vi "CRYO_MASTER_FULL-old.vi"() -> ()   [LabVIEW 2017]
uses:
  LSI218Data.lvclass
  LSI336Data.lvclass
  USBData.lvclass
  6240AData.lvclass
  <vilib>/DAQmx/create/channels.llb/DAQmx Create Channel (DO-Digital Output).vi
  <vilib>/DAQmx/miscellaneous.llb/DAQmx Fill In Error Info.vi
  <vilib>/DAQmx/create/channels.llb/DAQmx Create Channel (AO-Voltage-Basic).vi
  <vilib>/express/express arith-compare/Formula/XNode/ExpressFormulaBlockNode.xnode
  <vilib>/Analysis/NI_AALBase.lvlib
panel:
  in  "Record interval":i64=10
  out "Cycle #":u32=132
  in  "Measurement Interval (s)":dbl=0.3
  in  "Stop Button":bool
  in  "?":T1(tab)
  out "error out (USB6210/6218 AOUT)":errorcluster
  in  "AOUT 1 Label":string="KIKUSUI_I"
  in  "AOUT 0 Label":string="KIKUSUI_V"
  in  "DOUT Labels":string[](array[string])=["D_V1_NO", "D_V2_NC", "D_CV1"]
  in  "AOUT for Current CTRL":tag="Dev1/ao1"
  in  "AOUT For Voltage CTRL":tag="Dev1/ao0"
  out "AO task out":refnum<k21>="20200912_074213_AO"
  in  "Analog Out ON?":bool=TRUE
  in  "InstName (USB6218)":string="USB6218"
  in  "USB6218 Config":T2(array[cluster])=[{"Label"="F_1", "FileFormat"="%5.5f", "Active?"=TRUE, "Physical CH"="Dev1/ai0", " terminal\n type"=10083, "ConversionType"={"Type"=enum."SimpleProp", "ConversionParameters"=[0.0, 5.0, 0.0, 500.0]}, "VoltageLimits"=[0.0, 5.0]}, {"Label"="F_2", "FileFormat"="%5.5f", "Active?"=TRUE, "Physical CH"="Dev1/ai1", " terminal\n type"=10083, "ConversionType"={"Type"=enum."SimpleProp", "ConversionParameters"=[0.0, 5.0, 0.0, 200.0]}, "VoltageLimits"=[0.0, 5.0]}, {"Label"="F_3", "FileFormat"="%5.5f", "Active?"=TRUE, "Physical CH"="Dev1/ai2", " terminal\n type"=10083, "ConversionType"={"Type"=enum."SimpleProp", "ConversionParameters"=[0.0, 5.0, 0.0, 200.0]}, "VoltageLimits"=[0.0, 5.0]}, {"Label"="F_4", "FileFormat"="%5.5f", "Active?"=TRUE, "Physical CH"="Dev1/ai3", " terminal\n type"=10083, "ConversionType"={"Type"=enum."SimpleProp", "ConversionParameters"=[0.0, 5.0, 0.0, 500.0]}, "VoltageLimits"=[0.0, 5.0]}, {"Label"="F_5", "FileFormat"="%5.5f", "Active?"=TRUE, "Physical CH"="Dev1/ai4", " terminal\n type"=10083, "ConversionType"={"Type"=enum."SimpleProp", "ConversionParameters"=[0.0, 5.0, 0.0, 500.0]}, "VoltageLimits"=[0.0, 5.0]}, {"Label"="I_CV", "FileFormat"="%3.5f", "Active?"=TRUE, "Physical CH"="Dev1/ai5", " terminal\n type"=10083, "ConversionType"={"Type"=enum."SimpleProp", "ConversionParameters"=[0.0, 10.0, 0.0, 2000.0]}, "VoltageLimits"=[0.0, 10.0]}, {"Label"="CV1_answer", "FileFormat"="%3.5f", "Active?"=TRUE, "Physical CH"="Dev1/ai6", " terminal\n type"=10083, "ConversionType"={"Type"=enum."SimpleProp", "ConversionParameters"=[1.0, 5.0, 0.0, 100.0]}, "VoltageLimits"=[0.0, 5.0]}] {"terminal\n type" items=["Default"=-1, "RSE"=10083, "NRSE"=10078, "Differential"=10106, "Pseudodifferential"=12529]}
  out "error out (USB6218)":errorcluster
  out "error out (USB6210/6218 DOUT)":errorcluster
  out "DOUT task out":refnum<k21>="20200912_074213_DO"
  in  "DOUT Physical CH":tag[](array[tag])=["Dev1/port1/line0", "Dev1/port1/line1", "Dev1/port1/line2"]
  in  "Digital Out ON?":bool=TRUE
  in  "USB6210 Config":T2(array[cluster])=[{"Label"="P_ins", "FileFormat"="%5.5e", "Active?"=TRUE, "Physical CH"="Dev2/ai0", " terminal\n type"=10083, "ConversionType"={"Type"=enum."CC-10_LOG", "ConversionParameters"=[0.5, 9.0, 0.0, 1.0]}, "VoltageLimits"=[0.0, 10.0]}, {"Label"="P_4Kres", "FileFormat"="%5.5e", "Active?"=TRUE, "Physical CH"="Dev2/ai1", " terminal\n type"=10083, "ConversionType"={"Type"=enum."SimpleProp", "ConversionParameters"=[1.0, 5.0, 0.0, 200000.0]}, "VoltageLimits"=[0.0, 5.0]}, {"Label"="P_3HeIN", "FileFormat"="%5.5e", "Active?"=TRUE, "Physical CH"="Dev2/ai2", " terminal\n type"=10083, "ConversionType"={"Type"=enum."SimpleProp", "ConversionParameters"=[1.0, 5.0, 0.0, 200000.0]}, "VoltageLimits"=[0.0, 5.0]}, {"Label"="P_SldRTN", "FileFormat"="%5.5e", "Active?"=TRUE, "Physical CH"="Dev2/ai3", " terminal\n type"=10083, "ConversionType"={"Type"=enum."SimpleProp", "ConversionParameters"=[1.0, 5.0, 0.0, 200000.0]}, "VoltageLimits"=[0.0, 5.0]}, {"Label"="P_3Hepot", "FileFormat"="%5.5e", "Active?"=TRUE, "Physical CH"="Dev2/ai4", " terminal\n type"=10083, "ConversionType"={"Type"=enum."SimpleProp", "ConversionParameters"=[0.0, 10.0, 0.0, 133320.0]}, "VoltageLimits"=[0.0, 10.0]}, {"Label"="P_1Kpot", "FileFormat"="%5.5e", "Active?"=TRUE, "Physical CH"="Dev2/ai5", " terminal\n type"=10083, "ConversionType"={"Type"=enum."SimpleProp", "ConversionParameters"=[0.0, 10.0, 0.0, 133320.0]}, "VoltageLimits"=[0.0, 10.0]}, {"Label"="P_Dewar", "FileFormat"="%5.5e", "Active?"=TRUE, "Physical CH"="Dev2/ai6", " terminal\n type"=10083, "ConversionType"={"Type"=enum."SimpleProp", "ConversionParameters"=[1.0, 5.0, 0.0, 200000.0]}, "VoltageLimits"=[0.0, 5.0]}, {"Label"="DP_HEX4", "FileFormat"="%5.5e", "Active?"=TRUE, "Physical CH"="Dev2/ai7", " terminal\n type"=10083, "ConversionType"={"Type"=enum."SimpleProp", "ConversionParameters"=[1.0, 5.0, 0.0, 1000.0]}, "VoltageLimits"=[0.0, 5.0]}, {"Label"="DP_HEX5", "FileFormat"="%5.5e", "Active?"=TRUE, "Physical CH"="Dev2/ai8", " terminal\n type"=10083, "ConversionType"={"Type"=enum."SimpleProp", "ConversionParameters"=[1.0, 5.0, 0.0, 20000.0]}, "VoltageLimits"=[0.0, 5.0]}, {"Label"="L1", "FileFormat"="%5.5f", "Active?"=TRUE, "Physical CH"="Dev2/ai9", " terminal\n type"=10083, "ConversionType"={"Type"=enum."SimpleProp", "ConversionParameters"=[0.0, 10.0, 0.0, 100.0]}, "VoltageLimits"=[0.0, 10.0]}, {"Label"="L2-1", "FileFormat"="%5.5f", "Active?"=TRUE, "Physical CH"="Dev2/ai10", " terminal\n type"=10083, "ConversionType"={"Type"=enum."SimpleProp", "ConversionParameters"=[0.0, 10.0, 0.0, 100.0]}, "VoltageLimits"=[0.0, 10.0]}, {"Label"="L2-2", "FileFormat"="%5.5f", "Active?"=TRUE, "Physical CH"="Dev2/ai11", " terminal\n type"=10083, "ConversionType"={"Type"=enum."SimpleProp", "ConversionParameters"=[0.0, 10.0, 0.0, 100.0]}, "VoltageLimits"=[0.0, 10.0]}, {"Label"="L3", "FileFormat"="%5.5f", "Active?"=TRUE, "Physical CH"="Dev2/ai12", " terminal\n type"=10083, "ConversionType"={"Type"=enum."SimpleProp", "ConversionParameters"=[0.0, 10.0, 0.0, 100.0]}, "VoltageLimits"=[0.0, 10.0]}] {"terminal\n type" items=["Default"=-1, "RSE"=10083, "NRSE"=10078, "Differential"=10106, "Pseudodifferential"=12529]}
  in  "RUN identifier":string="PreCooling"
  in  "Base Path":path=path "C:/LabVIEW/DATA/Precooling"
  in  "InstName (USB6210)":string="USB6210"
  out "error out (USB6210)":errorcluster
  out "File Refn USB AO":refnum<file>
  out "File Refn USB DO":refnum<file>
  out "error out (LSI336)":errorcluster
  in  "InstName (LSI336)":string="LSI336"
  in  "FileFormat (336)":string="%4.4f"
  in  "LSI336Settings(X,Y)":T3(array[cluster])=[{"LSIName"="LSi336X", "Labels"=["T1K3-1", "T1K3-2", "T3He5", "T3He8"], "SensorLocations"=[enum."T1K3-1", enum."T1K3-2", enum."T3He5", enum."T3He8"], "Active?"=TRUE, "VISA res. name"="GPIB0::6::INSTR"}, {"LSIName"="LSi336Y", "Labels"=["T3He6-1", "T3He6-2", "T3He7-1", "T3He7-2"], "SensorLocations"=[enum."T3He6-1", enum."T3He6-2", enum."T3He7-1", enum."T3He7-2"], "Active?"=TRUE, "VISA res. name"="GPIB0::2::INSTR"}]
  in  "FileFormat (218)":string="%4.4f"
  in  "InstName (LSI218)":string="LSI218"
  in  "LSI218Settings(A-F)":T3(array[cluster])=[{"LSIName"="LSI218A", "Labels"=["T3He10", "T3He1-1", "TTH3", "TTH4", "TTH1", "TTH2", "T4He1", "T1K1"], "SensorLocations"=[enum."T3He10", enum."T3He1-1", enum."TTH3", enum."TTH4", enum."TTH1", enum."TTH2", enum."T4He1", enum."T1K1"], "Active?"=TRUE, "VISA res. name"="GPIB0::7::INSTR"}, {"LSIName"="LSI218B", "Labels"=["N.C.", "N.C.", "N.C.", "N.C.", "T3He2-1", "T3He2-2", "T3He3", "T3He1-4"], "SensorLocations"=[enum."N.C.", enum."N.C.", enum."N.C.", enum."T3He1-4", enum."T3He2-1", enum."T3He2-2", enum."T3He3", enum."T3He1-4"], "Active?"=TRUE, "VISA res. name"="GPIB0::4::INSTR"}, {"LSIName"="LSI218C", "Labels"=["T4He3-1", "T4He3-2", "T4He3-3", "T4He3-4", "T4He2-1", "T4He2-2", "T4He4", "T4He5"], "SensorLocations"=[enum."T4He3-1", enum."T4He3-2", enum."T4He3-3", enum."T4He3-4", enum."T4He2-1", enum."T4He2-2", enum."T4He4", enum."T4He5"], "Active?"=TRUE, "VISA res. name"="GPIB0::3::INSTR"}, {"LSIName"="LSI218D", "Labels"=["T4He6", "T4He9", "T3He1-2", "T3He1-3", "T4He7", "T4He8", "T4He10", "T1K6"], "SensorLocations"=[enum."T4He6", enum."T4He9", enum."T3He1-2", enum."T3He1-3", enum."T4He7", enum."T4He8", enum."T4He10", enum."T1K6"], "Active?"=TRUE, "VISA res. name"="GPIB0::5::INSTR"}, {"LSIName"="LSI218E", "Labels"=["TIP1", "N.C.", "TIP2", "N.C.", "TIP3", "TIP4", "TIP5", "N.C."], "SensorLocations"=[enum."TIP1", enum."N.C.", enum."TIP2", enum."N.C.", enum."TIP3", enum."TIP4", enum."TIP5", enum."N.C."], "Active?"=TRUE, "VISA res. name"="GPIB0::11::INSTR"}, {"LSIName"="LSI218F", "Labels"=["T1K2", "T1K4", "T1K5", "T3He4", "T3He9", "TIP6", "N.C.", "N.C."], "SensorLocations"=[enum."T1K2", enum."T1K4", enum."T1K5", enum."T3He4", enum."T3He9", enum."TIP6", enum."N.C.", enum."N.C."], "Active?"=TRUE, "VISA res. name"="GPIB0::8::INSTR"}]
  out "error out (LSI218)":errorcluster
  out "Graph 3":T4(graph) caption="XY Graph"
  out "Graph 1":T4(graph)=[{"TimeArray"=[timestamp(3682708934.7497134 s since 1904-01-01), timestamp(3682708935.064348 s since 1904-01-01), timestamp(3682708935.3896832 s since 1904-01-01), timestamp(3682708935.7026334 s since 1904-01-01), timestamp(3682708936.0021167 s since 1904-01-01), timestamp(3682708936.3049774 s since 1904-01-01), timestamp(3682708936.605407 s since 1904-01-01), timestamp(3682708936.903053 s since 1904-01-01), timestamp(3682708937.3067694 s since 1904-01-01), timestamp(3682708937.611465 s since 1904-01-01), timestamp(3682708937.909672 s since 1904-01-01), timestamp(3682708938.228514 s since 1904-01-01), timestamp(3682708938.527811 s since 1904-01-01), timestamp(3682708938.931336 s since 1904-01-01), timestamp(3682708940.012947 s since 1904-01-01), timestamp(3682708940.32849 s since 1904-01-01), timestamp(3682708940.631708 s since 1904-01-01), timestamp(3682708940.946489 s since 1904-01-01), timestamp(3682708941.244303 s since 1904-01-01), timestamp(3682708941.542656 s since 1904-01-01), timestamp(3682708941.8474927 s since 1904-01-01), timestamp(3682708942.3104415 s since 1904-01-01), timestamp(3682708942.6136575 s since 1904-01-01), timestamp(3682708942.916794 s since 1904-01-01), timestamp(3682708943.238447 s since 1904-01-01), timestamp(3682708943.5371313 s since 1904-01-01), timestamp(3682708943.857245 s since 1904-01-01), timestamp(3682708944.1856494 s since 1904-01-01), timestamp(3682708944.4866023 s since 1904-01-01), timestamp(3682708944.805397 s since 1904-01-01), timestamp(3682708945.111448 s since 1904-01-01), timestamp(3682708945.435288 s since 1904-01-01), timestamp(3682708945.7333007 s since 1904-01-01), timestamp(3682708946.0530386 s since 1904-01-01), timestamp(3682708946.4366784 s since 1904-01-01), timestamp(3682708946.732824 s since 1904-01-01), timestamp(3682708947.0537186 s since 1904-01-01), timestamp(3682708947.3846655 s since 1904-01-01), timestamp(3682708947.712872 s since 1904-01-01), timestamp(3682708948.0188503 s since 1904-01-01), timestamp(3682708948.737391 s since 1904-01-01), timestamp(3682708949.201587 s since 1904-01-01), timestamp(3682708949.502657 s since 1904-01-01), timestamp(3682708949.805978 s since 1904-01-01), timestamp(3682708950.1212378 s since 1904-01-01), timestamp(3682708950.4333377 s since 1904-01-01), timestamp(3682708950.732243 s since 1904-01-01), timestamp(3682708951.1057153 s since 1904-01-01), timestamp(3682708951.4068193 s since 1904-01-01), timestamp(3682708951.8357983 s since 1904-01-01), timestamp(3682708952.143476 s since 1904-01-01), timestamp(3682708952.4476566 s since 1904-01-01), timestamp(3682708952.7855697 s since 1904-01-01), timestamp(3682708953.086301 s since 1904-01-01), timestamp(3682708953.4027033 s since 1904-01-01), timestamp(3682708953.706577 s since 1904-01-01), timestamp(3682708954.023016 s since 1904-01-01), timestamp(3682708954.330558 s since 1904-01-01), timestamp(3682708954.643428 s since 1904-01-01), timestamp(3682708955.050496 s since 1904-01-01), timestamp(3682708955.3527017 s since 1904-01-01), timestamp(3682708955.7328424 s since 1904-01-01), timestamp(3682708956.0574985 s since 1904-01-01), timestamp(3682708956.3904 s since 1904-01-01), timestamp(3682708956.7025185 s since 1904-01-01), timestamp(3682708957.032419 s since 1904-01-01), timestamp(3682708957.351427 s since 1904-01-01), timestamp(3682708957.6656775 s since 1904-01-01), timestamp(3682708958.051097 s since 1904-01-01), timestamp(3682708958.4033985 s since 1904-01-01), timestamp(3682708958.7021422 s since 1904-01-01), timestamp(3682708959.004737 s since 1904-01-01), timestamp(3682708959.3058767 s since 1904-01-01), timestamp(3682708959.6056495 s since 1904-01-01), timestamp(3682708959.9347386 s since 1904-01-01), timestamp(3682708960.252382 s since 1904-01-01), timestamp(3682708960.553459 s since 1904-01-01), timestamp(3682708960.8641214 s since 1904-01-01), timestamp(3682708961.160152 s since 1904-01-01), timestamp(3682708961.487622 s since 1904-01-01), timestamp(3682708961.788169 s since 1904-01-01), timestamp(3682708962.0896144 s since 1904-01-01), timestamp(3682708962.406388 s since 1904-01-01), timestamp(3682708962.70866 s since 1904-01-01), timestamp(3682708963.033897 s since 1904-01-01), timestamp(3682708963.3512735 s since 1904-01-01), timestamp(3682708963.668318 s since 1904-01-01), timestamp(3682708963.9877753 s since 1904-01-01), timestamp(3682708964.2907033 s since 1904-01-01), timestamp(3682708964.606549 s since 1904-01-01), timestamp(3682708964.906368 s since 1904-01-01), timestamp(3682708965.217731 s since 1904-01-01), timestamp(3682708965.5397863 s since 1904-01-01), timestamp(3682708965.8690424 s since 1904-01-01), timestamp(3682708966.190765 s since 1904-01-01), timestamp(3682708966.5023417 s since 1904-01-01), timestamp(3682708966.806744 s since 1904-01-01), timestamp(3682708967.1092105 s since 1904-01-01), timestamp(3682708967.406003 s since 1904-01-01), timestamp(3682708967.710469 s since 1904-01-01), timestamp(3682708968.041528 s since 1904-01-01), timestamp(3682708968.365668 s since 1904-01-01), timestamp(3682708968.8523655 s since 1904-01-01), timestamp(3682708969.1540494 s since 1904-01-01), timestamp(3682708969.4895535 s since 1904-01-01), timestamp(3682708969.7907286 s since 1904-01-01), timestamp(3682708970.105831 s since 1904-01-01), timestamp(3682708970.4602976 s since 1904-01-01), timestamp(3682708970.963533 s since 1904-01-01), timestamp(3682708971.301882 s since 1904-01-01), timestamp(3682708971.6079335 s since 1904-01-01), timestamp(3682708971.9060354 s since 1904-01-01), timestamp(3682708972.2345 s since 1904-01-01), timestamp(3682708972.5527015 s since 1904-01-01), timestamp(3682708972.8548064 s since 1904-01-01), timestamp(3682708973.582567 s since 1904-01-01), timestamp(3682708973.8891873 s since 1904-01-01), timestamp(3682708974.1884327 s since 1904-01-01), timestamp(3682708974.5010185 s since 1904-01-01), timestamp(3682708974.8142066 s since 1904-01-01), timestamp(3682708975.1175103 s since 1904-01-01), timestamp(3682708975.4374647 s since 1904-01-01), timestamp(3682708975.7527 s since 1904-01-01), timestamp(3682708976.0583982 s since 1904-01-01), timestamp(3682708976.3644648 s since 1904-01-01), timestamp(3682708976.689261 s since 1904-01-01), timestamp(3682708977.0021367 s since 1904-01-01), timestamp(3682708977.3057 s since 1904-01-01), timestamp(3682708977.6422114 s since 1904-01-01), timestamp(3682708977.9607697 s since 1904-01-01), timestamp(3682708978.2889266 s since 1904-01-01), timestamp(3682708978.7650247 s since 1904-01-01)], "DataArray"=[102202.16534140152, 100161.43201016451, 100789.60275186355, 100345.60782032329, 102337.00779239179, 101526.30582974949, 102083.76617517172, 102660.95994909719, 100931.02351867667, 101384.88517891317, 103307.21992056293, 101878.21277938908, 100806.04675539682]}] caption="XY Graph"
  in  "FIle suffix 4":string="Graph4"
  in  "Take Screenshot! 4":bool
  in  "FIle suffix 3":string="Graph3"
  in  "Take Screenshot! 3":bool
  in  "FIle suffix 2":string="Graph2"
  in  "Take Screenshot! 2":bool
  in  "FIle suffix 1":string="Graph1"
  in  "Take Screenshot! 1":bool
  in  "log/linear 2":bool
  in  "Tab Control 2":T5(tab)
  in  "Plot selecter (USB6210)\n    1      2     3     4":bool[][](array[boolean])=[[FALSE, FALSE, TRUE, FALSE], [FALSE, FALSE, TRUE, FALSE], [FALSE, FALSE, TRUE, FALSE], [FALSE, FALSE, TRUE, FALSE], [FALSE, FALSE, TRUE, FALSE], [FALSE, FALSE, TRUE, FALSE], [TRUE, FALSE, FALSE, FALSE], [FALSE, FALSE, TRUE, FALSE], [FALSE, FALSE, TRUE, FALSE], [FALSE, FALSE, FALSE, TRUE], [FALSE, FALSE, FALSE, TRUE], [FALSE, FALSE, FALSE, TRUE], [FALSE, FALSE, FALSE, TRUE], [FALSE, FALSE, FALSE, FALSE], [FALSE, FALSE, FALSE, FALSE], [FALSE, FALSE, FALSE, FALSE]]
  out "All Labels (USB6210)":string[](array[string])=["P_ins", "P_4Kres", "P_3HeIN", "P_SldRTN", "P_3Hepot", "P_1Kpot", "P_Dewar", "DP_HEX4", "DP_HEX5", "L1", "L2-1", "L2-2", "L3"]
  out "Last Data \n(USB6210)":dbl[](array[numeric])=[0.0002840544512641805, 101675.94822078843, 101115.19883009115, 101138.22078317008, 101187.0271133805, 101386.92986598553, 102226.83192072672, -14.050296706315413, 60.37240293708335, 100.07360118845727, 0.1408656089962046, 0.11784872774401622, 0.16848586636495688] format="%#_6e"
  out "Time of Last Measurement (USB6210)":timestamp=timestamp(3682708978.7650247 s since 1904-01-01)
  out "USB6210 Status":T6(ring)=enum."Ready"
  out "Last Vol\n(USB6210)":dbl[](array[numeric])=[5.726700799630656, 3.0335189644157685, 3.022303976601823, 3.0227644156634015, 7.5897860121047485, 7.604780217970712, 3.0445366384145345, 0.9437988131747383, 1.0120744805874167, 10.007360118845728, 0.01408656089962046, 0.011784872774401623, 0.016848586636495688] format="%_5f"
  out "Time of Last Measurement (USB6218)":timestamp=timestamp(3682708978.761338 s since 1904-01-01)
  out "USB6218 Status":T6(ring)=enum."Ready"
  out "Last Vol \n(USB6218)":dbl[](array[numeric])=[0.11165481522010053, 0.007099956900383277, 0.005192981435202531, -0.08736109093903988, 0.3091911402370971, 0.017826732521314358, -0.0006594605889951533] format="%_5f"
  out "Last Data \n(USB6218)":dbl[](array[numeric])=[11.165481522010053, 0.28399827601533106, 0.20771925740810127, -8.736109093903988, 30.91911402370971, 0.017826732521314358, -25.01648651472488] format="%#_6e"
  out "All Labels (USB6218)":string[](array[string])=["F_1", "F_2", "F_3", "F_4", "F_5", "I_CV", "CV1_answer"]
  in  "Plot selecter (USB6218)\n    1      2     3     4":bool[][](array[boolean])=[[FALSE, FALSE, TRUE, FALSE], [FALSE, FALSE, TRUE, FALSE], [FALSE, FALSE, TRUE, FALSE], [FALSE, FALSE, TRUE, FALSE], [FALSE, FALSE, TRUE, FALSE], [FALSE, FALSE, TRUE, FALSE], [FALSE, FALSE, FALSE, FALSE], [FALSE, FALSE, TRUE, FALSE], [FALSE, FALSE, TRUE, FALSE], [FALSE, FALSE, FALSE, TRUE], [FALSE, FALSE, FALSE, TRUE], [FALSE, FALSE, FALSE, TRUE], [FALSE, FALSE, FALSE, TRUE], [FALSE, FALSE, FALSE, FALSE], [FALSE, FALSE, FALSE, FALSE], [FALSE, FALSE, FALSE, FALSE]]
  out "Time of Last Measurement (LSI218)":timestamp=timestamp(3682708978.761338 s since 1904-01-01)
  out "LSI218 Status":T7(ring)=enum."Measuring"
  out "Last Data \nLSI218 (1)":dbl[](array[numeric])=[284.43, 290.03, 243.23, 256.15, 171.54, 180.77, 63.049, 117.3, 30.0, 0.0, 0.0, 0.0, 202.72, 191.34, 122.93, 289.61, 292.19, 292.34, 291.95, 292.02, 202.48, 197.55, 192.92, 186.55]
  out "Labels LSI218 (1)":string[](array[string])=["T3He10", "T3He1-1", "TTH3", "TTH4", "TTH1", "TTH2", "T4He1", "T1K1", "N.C.", "N.C.", "N.C.", "N.C.", "T3He2-1", "T3He2-2", "T3He3", "T3He1-4", "T4He3-1", "T4He3-2", "T4He3-3", "T4He3-4", "T4He2-1", "T4He2-2", "T4He4", "T4He5"]
  in  "Plot selecter LSI218(1)\n    1      2     3     4":bool[][](array[boolean])=[[FALSE, FALSE, FALSE, FALSE], [FALSE, FALSE, FALSE, FALSE], [FALSE, FALSE, FALSE, FALSE], [FALSE, FALSE, FALSE, FALSE], [FALSE, FALSE, FALSE, FALSE], [FALSE, FALSE, FALSE, FALSE], [FALSE, FALSE, FALSE, FALSE], [FALSE, FALSE, FALSE, FALSE], [FALSE, FALSE, FALSE, FALSE], [FALSE, FALSE, FALSE, FALSE], [FALSE, FALSE, FALSE, FALSE], [FALSE, FALSE, FALSE, FALSE], [FALSE, FALSE, FALSE, FALSE], [FALSE, FALSE, FALSE, FALSE], [FALSE, FALSE, FALSE, FALSE], [FALSE, FALSE, FALSE, FALSE], [FALSE, FALSE, FALSE, FALSE], [FALSE, FALSE, FALSE, FALSE], [FALSE, FALSE, FALSE, FALSE], [FALSE, FALSE, FALSE, FALSE], [FALSE, FALSE, FALSE, FALSE], [FALSE, FALSE, FALSE, FALSE], [FALSE, FALSE, FALSE, FALSE], [FALSE, FALSE, FALSE, FALSE]]
  out "Active?\n (1)":bool[](array[boolean])=[TRUE, TRUE, TRUE, TRUE, TRUE, TRUE, TRUE, TRUE, TRUE, TRUE, TRUE, TRUE, TRUE, TRUE, TRUE, TRUE, TRUE, TRUE, TRUE, TRUE, TRUE, TRUE, TRUE, TRUE]
  out "Labels LSI218 (2)":string[](array[string])=["T4He6", "T4He9", "T3He1-2", "T3He1-3", "T4He7", "T4He8", "T4He10", "T1K6", "TIP1", "N.C.", "TIP2", "N.C.", "TIP3", "TIP4", "TIP5", "N.C.", "T1K2", "T1K4", "T1K5", "T3He4", "T3He9", "TIP6", "N.C.", "N.C."]
  out "Active?\n(2)":bool[](array[boolean])=[TRUE, TRUE, TRUE, TRUE, TRUE, TRUE, TRUE, TRUE, TRUE, TRUE, TRUE, TRUE, TRUE, TRUE, TRUE, TRUE, TRUE, TRUE, TRUE, TRUE, TRUE, TRUE, TRUE, TRUE]
  out "Last Data \nLSI218 (2)":dbl[](array[numeric])=[192.44, 234.78, 290.18, 290.03, 246.41, 271.83, 269.02, 283.26, 278.46, 0.0, 229.12, 688.49, 197.75, 114.09, 159.57, 688.58, 121.27, 92.631, 95.353, 144.45, 121.36, 152.88, 0.433, 0.0]
  in  "Plot selecter LSI218(2)\n    1      2     3     4":bool[][](array[boolean])=[[FALSE, TRUE, FALSE, FALSE], [FALSE, TRUE, FALSE, FALSE], [FALSE, TRUE, FALSE, FALSE], [FALSE, TRUE, FALSE, FALSE], [FALSE, TRUE, FALSE, FALSE], [FALSE, TRUE, FALSE, FALSE], [FALSE, TRUE, FALSE, FALSE], [FALSE, TRUE, FALSE, FALSE], [FALSE, TRUE, FALSE, FALSE], [FALSE, TRUE, FALSE, FALSE], [FALSE, TRUE, FALSE, FALSE], [FALSE, FALSE, FALSE, FALSE], [FALSE, FALSE, FALSE, FALSE], [FALSE, FALSE, FALSE, FALSE], [FALSE, FALSE, FALSE, FALSE], [FALSE, FALSE, FALSE, FALSE], [FALSE, FALSE, FALSE, FALSE], [FALSE, FALSE, FALSE, FALSE], [FALSE, FALSE, FALSE, FALSE], [FALSE, FALSE, FALSE, FALSE], [FALSE, FALSE, FALSE, FALSE], [FALSE, FALSE, FALSE, FALSE], [FALSE, FALSE, FALSE, FALSE], [FALSE, FALSE, FALSE, FALSE]]
  in  "Plot selecter LSI336 \n     1      2     3     4":bool[][](array[boolean])=[[FALSE, TRUE, FALSE, FALSE], [FALSE, TRUE, FALSE, FALSE], [FALSE, TRUE, FALSE, FALSE], [FALSE, TRUE, FALSE, FALSE], [FALSE, TRUE, FALSE, FALSE], [FALSE, TRUE, FALSE, FALSE], [FALSE, TRUE, FALSE, FALSE], [FALSE, TRUE, FALSE, FALSE]]
  out "Time of Last Measurement (LSI336)":timestamp=timestamp(3682708978.761338 s since 1904-01-01)
  out "Last Data \nLSI336":dbl[](array[numeric])=[94.5454, 94.3475, 128.374, 133.795, 135.029, 135.063, 134.969, 134.048]
  out "Active?\n(LSI336)":bool[](array[boolean])=[TRUE, TRUE, TRUE, TRUE, TRUE, TRUE, TRUE, TRUE]
  out "Labels LSI336":string[](array[string])=["T1K3-1", "T1K3-2", "T3He5", "T3He8", "T3He6-1", "T3He6-2", "T3He7-1", "T3He7-2"]
  out "LSI336 Status":T7(ring)=enum."Measuring"
  in  "log/linear 1":bool
  out "Graph 2":T4(graph) caption="XY Graph"
  out "Graph 4":T4(graph)=[{"TimeArray"=[timestamp(3682708934.7497134 s since 1904-01-01), timestamp(3682708935.064348 s since 1904-01-01), timestamp(3682708935.3896832 s since 1904-01-01), timestamp(3682708935.7026334 s since 1904-01-01), timestamp(3682708936.0021167 s since 1904-01-01), timestamp(3682708936.3049774 s since 1904-01-01), timestamp(3682708936.605407 s since 1904-01-01), timestamp(3682708936.903053 s since 1904-01-01), timestamp(3682708937.3067694 s since 1904-01-01), timestamp(3682708937.611465 s since 1904-01-01), timestamp(3682708937.909672 s since 1904-01-01), timestamp(3682708938.228514 s since 1904-01-01), timestamp(3682708938.527811 s since 1904-01-01), timestamp(3682708938.931336 s since 1904-01-01), timestamp(3682708940.012947 s since 1904-01-01), timestamp(3682708940.32849 s since 1904-01-01), timestamp(3682708940.631708 s since 1904-01-01), timestamp(3682708940.946489 s since 1904-01-01), timestamp(3682708941.244303 s since 1904-01-01), timestamp(3682708941.542656 s since 1904-01-01), timestamp(3682708941.8474927 s since 1904-01-01), timestamp(3682708942.3104415 s since 1904-01-01), timestamp(3682708942.6136575 s since 1904-01-01), timestamp(3682708942.916794 s since 1904-01-01), timestamp(3682708943.238447 s since 1904-01-01), timestamp(3682708943.5371313 s since 1904-01-01), timestamp(3682708943.857245 s since 1904-01-01), timestamp(3682708944.1856494 s since 1904-01-01), timestamp(3682708944.4866023 s since 1904-01-01), timestamp(3682708944.805397 s since 1904-01-01), timestamp(3682708945.111448 s since 1904-01-01), timestamp(3682708945.435288 s since 1904-01-01), timestamp(3682708945.7333007 s since 1904-01-01), timestamp(3682708946.0530386 s since 1904-01-01), timestamp(3682708946.4366784 s since 1904-01-01), timestamp(3682708946.732824 s since 1904-01-01), timestamp(3682708947.0537186 s since 1904-01-01), timestamp(3682708947.3846655 s since 1904-01-01), timestamp(3682708947.712872 s since 1904-01-01), timestamp(3682708948.0188503 s since 1904-01-01), timestamp(3682708948.737391 s since 1904-01-01), timestamp(3682708949.201587 s since 1904-01-01), timestamp(3682708949.502657 s since 1904-01-01), timestamp(3682708949.805978 s since 1904-01-01), timestamp(3682708950.1212378 s since 1904-01-01), timestamp(3682708950.4333377 s since 1904-01-01), timestamp(3682708950.732243 s since 1904-01-01), timestamp(3682708951.1057153 s since 1904-01-01), timestamp(3682708951.4068193 s since 1904-01-01), timestamp(3682708951.8357983 s since 1904-01-01), timestamp(3682708952.143476 s since 1904-01-01), timestamp(3682708952.4476566 s since 1904-01-01), timestamp(3682708952.7855697 s since 1904-01-01), timestamp(3682708953.086301 s since 1904-01-01), timestamp(3682708953.4027033 s since 1904-01-01), timestamp(3682708953.706577 s since 1904-01-01), timestamp(3682708954.023016 s since 1904-01-01), timestamp(3682708954.330558 s since 1904-01-01), timestamp(3682708954.643428 s since 1904-01-01), timestamp(3682708955.050496 s since 1904-01-01), timestamp(3682708955.3527017 s since 1904-01-01), timestamp(3682708955.7328424 s since 1904-01-01), timestamp(3682708956.0574985 s since 1904-01-01), timestamp(3682708956.3904 s since 1904-01-01), timestamp(3682708956.7025185 s since 1904-01-01), timestamp(3682708957.032419 s since 1904-01-01), timestamp(3682708957.351427 s since 1904-01-01), timestamp(3682708957.6656775 s since 1904-01-01), timestamp(3682708958.051097 s since 1904-01-01), timestamp(3682708958.4033985 s since 1904-01-01), timestamp(3682708958.7021422 s since 1904-01-01), timestamp(3682708959.004737 s since 1904-01-01), timestamp(3682708959.3058767 s since 1904-01-01), timestamp(3682708959.6056495 s since 1904-01-01), timestamp(3682708959.9347386 s since 1904-01-01), timestamp(3682708960.252382 s since 1904-01-01), timestamp(3682708960.553459 s since 1904-01-01), timestamp(3682708960.8641214 s since 1904-01-01), timestamp(3682708961.160152 s since 1904-01-01), timestamp(3682708961.487622 s since 1904-01-01), timestamp(3682708961.788169 s since 1904-01-01), timestamp(3682708962.0896144 s since 1904-01-01), timestamp(3682708962.406388 s since 1904-01-01), timestamp(3682708962.70866 s since 1904-01-01), timestamp(3682708963.033897 s since 1904-01-01), timestamp(3682708963.3512735 s since 1904-01-01), timestamp(3682708963.668318 s since 1904-01-01), timestamp(3682708963.9877753 s since 1904-01-01), timestamp(3682708964.2907033 s since 1904-01-01), timestamp(3682708964.606549 s since 1904-01-01), timestamp(3682708964.906368 s since 1904-01-01), timestamp(3682708965.217731 s since 1904-01-01), timestamp(3682708965.5397863 s since 1904-01-01), timestamp(3682708965.8690424 s since 1904-01-01), timestamp(3682708966.190765 s since 1904-01-01), timestamp(3682708966.5023417 s since 1904-01-01), timestamp(3682708966.806744 s since 1904-01-01), timestamp(3682708967.1092105 s since 1904-01-01), timestamp(3682708967.406003 s since 1904-01-01), timestamp(3682708967.710469 s since 1904-01-01), timestamp(3682708968.041528 s since 1904-01-01), timestamp(3682708968.365668 s since 1904-01-01), timestamp(3682708968.8523655 s since 1904-01-01), timestamp(3682708969.1540494 s since 1904-01-01), timestamp(3682708969.4895535 s since 1904-01-01), timestamp(3682708969.7907286 s since 1904-01-01), timestamp(3682708970.105831 s since 1904-01-01), timestamp(3682708970.4602976 s since 1904-01-01), timestamp(3682708970.963533 s since 1904-01-01), timestamp(3682708971.301882 s since 1904-01-01), timestamp(3682708971.6079335 s since 1904-01-01), timestamp(3682708971.9060354 s since 1904-01-01), timestamp(3682708972.2345 s since 1904-01-01), timestamp(3682708972.5527015 s since 1904-01-01), timestamp(3682708972.8548064 s since 1904-01-01), timestamp(3682708973.582567 s since 1904-01-01), timestamp(3682708973.8891873 s since 1904-01-01), timestamp(3682708974.1884327 s since 1904-01-01), timestamp(3682708974.5010185 s since 1904-01-01), timestamp(3682708974.8142066 s since 1904-01-01), timestamp(3682708975.1175103 s since 1904-01-01), timestamp(3682708975.4374647 s since 1904-01-01), timestamp(3682708975.7527 s since 1904-01-01), timestamp(3682708976.0583982 s since 1904-01-01), timestamp(3682708976.3644648 s since 1904-01-01), timestamp(3682708976.689261 s since 1904-01-01), timestamp(3682708977.0021367 s since 1904-01-01), timestamp(3682708977.3057 s since 1904-01-01), timestamp(3682708977.6422114 s since 1904-01-01), timestamp(3682708977.9607697 s since 1904-01-01), timestamp(3682708978.2889266 s since 1904-01-01), timestamp(3682708978.7650247 s since 1904-01-01)], "DataArray"=[100.06505169937662, 100.0913578166008, 100.07097057589947, 100.0722858814967, 100.04006088884337, 100.09201547031509, 100.04006088897802, 100.01375477333622, 100.06833996442191, 100.05058333549653, 100.01441242568171, 100.06899761748156, 100.07688945274376]}, {"TimeArray"=[timestamp(3682708934.7497134 s since 1904-01-01), timestamp(3682708935.064348 s since 1904-01-01), timestamp(3682708935.3896832 s since 1904-01-01), timestamp(3682708935.7026334 s since 1904-01-01), timestamp(3682708936.0021167 s since 1904-01-01), timestamp(3682708936.3049774 s since 1904-01-01), timestamp(3682708936.605407 s since 1904-01-01), timestamp(3682708936.903053 s since 1904-01-01), timestamp(3682708937.3067694 s since 1904-01-01), timestamp(3682708937.611465 s since 1904-01-01), timestamp(3682708937.909672 s since 1904-01-01), timestamp(3682708938.228514 s since 1904-01-01), timestamp(3682708938.527811 s since 1904-01-01), timestamp(3682708938.931336 s since 1904-01-01), timestamp(3682708940.012947 s since 1904-01-01), timestamp(3682708940.32849 s since 1904-01-01), timestamp(3682708940.631708 s since 1904-01-01), timestamp(3682708940.946489 s since 1904-01-01), timestamp(3682708941.244303 s since 1904-01-01), timestamp(3682708941.542656 s since 1904-01-01), timestamp(3682708941.8474927 s since 1904-01-01), timestamp(3682708942.3104415 s since 1904-01-01), timestamp(3682708942.6136575 s since 1904-01-01), timestamp(3682708942.916794 s since 1904-01-01), timestamp(3682708943.238447 s since 1904-01-01), timestamp(3682708943.5371313 s since 1904-01-01), timestamp(3682708943.857245 s since 1904-01-01), timestamp(3682708944.1856494 s since 1904-01-01), timestamp(3682708944.4866023 s since 1904-01-01), timestamp(3682708944.805397 s since 1904-01-01), timestamp(3682708945.111448 s since 1904-01-01), timestamp(3682708945.435288 s since 1904-01-01), timestamp(3682708945.7333007 s since 1904-01-01), timestamp(3682708946.0530386 s since 1904-01-01), timestamp(3682708946.4366784 s since 1904-01-01), timestamp(3682708946.732824 s since 1904-01-01), timestamp(3682708947.0537186 s since 1904-01-01), timestamp(3682708947.3846655 s since 1904-01-01), timestamp(3682708947.712872 s since 1904-01-01), timestamp(3682708948.0188503 s since 1904-01-01), timestamp(3682708948.737391 s since 1904-01-01), timestamp(3682708949.201587 s since 1904-01-01), timestamp(3682708949.502657 s since 1904-01-01), timestamp(3682708949.805978 s since 1904-01-01), timestamp(3682708950.1212378 s since 1904-01-01), timestamp(3682708950.4333377 s since 1904-01-01), timestamp(3682708950.732243 s since 1904-01-01), timestamp(3682708951.1057153 s since 1904-01-01), timestamp(3682708951.4068193 s since 1904-01-01), timestamp(3682708951.8357983 s since 1904-01-01), timestamp(3682708952.143476 s since 1904-01-01), timestamp(3682708952.4476566 s since 1904-01-01), timestamp(3682708952.7855697 s since 1904-01-01), timestamp(3682708953.086301 s since 1904-01-01), timestamp(3682708953.4027033 s since 1904-01-01), timestamp(3682708953.706577 s since 1904-01-01), timestamp(3682708954.023016 s since 1904-01-01), timestamp(3682708954.330558 s since 1904-01-01), timestamp(3682708954.643428 s since 1904-01-01), timestamp(3682708955.050496 s since 1904-01-01), timestamp(3682708955.3527017 s since 1904-01-01), timestamp(3682708955.7328424 s since 1904-01-01), timestamp(3682708956.0574985 s since 1904-01-01), timestamp(3682708956.3904 s since 1904-01-01), timestamp(3682708956.7025185 s since 1904-01-01), timestamp(3682708957.032419 s since 1904-01-01), timestamp(3682708957.351427 s since 1904-01-01), timestamp(3682708957.6656775 s since 1904-01-01), timestamp(3682708958.051097 s since 1904-01-01), timestamp(3682708958.4033985 s since 1904-01-01), timestamp(3682708958.7021422 s since 1904-01-01), timestamp(3682708959.004737 s since 1904-01-01), timestamp(3682708959.3058767 s since 1904-01-01), timestamp(3682708959.6056495 s since 1904-01-01), timestamp(3682708959.9347386 s since 1904-01-01), timestamp(3682708960.252382 s since 1904-01-01), timestamp(3682708960.553459 s since 1904-01-01), timestamp(3682708960.8641214 s since 1904-01-01), timestamp(3682708961.160152 s since 1904-01-01), timestamp(3682708961.487622 s since 1904-01-01), timestamp(3682708961.788169 s since 1904-01-01), timestamp(3682708962.0896144 s since 1904-01-01), timestamp(3682708962.406388 s since 1904-01-01), timestamp(3682708962.70866 s since 1904-01-01), timestamp(3682708963.033897 s since 1904-01-01), timestamp(3682708963.3512735 s since 1904-01-01), timestamp(3682708963.668318 s since 1904-01-01), timestamp(3682708963.9877753 s since 1904-01-01), timestamp(3682708964.2907033 s since 1904-01-01), timestamp(3682708964.606549 s since 1904-01-01), timestamp(3682708964.906368 s since 1904-01-01), timestamp(3682708965.217731 s since 1904-01-01), timestamp(3682708965.5397863 s since 1904-01-01), timestamp(3682708965.8690424 s since 1904-01-01), timestamp(3682708966.190765 s since 1904-01-01), timestamp(3682708966.5023417 s since 1904-01-01), timestamp(3682708966.806744 s since 1904-01-01), timestamp(3682708967.1092105 s since 1904-01-01), timestamp(3682708967.406003 s since 1904-01-01), timestamp(3682708967.710469 s since 1904-01-01), timestamp(3682708968.041528 s since 1904-01-01), timestamp(3682708968.365668 s since 1904-01-01), timestamp(3682708968.8523655 s since 1904-01-01), timestamp(3682708969.1540494 s since 1904-01-01), timestamp(3682708969.4895535 s since 1904-01-01), timestamp(3682708969.7907286 s since 1904-01-01), timestamp(3682708970.105831 s since 1904-01-01), timestamp(3682708970.4602976 s since 1904-01-01), timestamp(3682708970.963533 s since 1904-01-01), timestamp(3682708971.301882 s since 1904-01-01), timestamp(3682708971.6079335 s since 1904-01-01), timestamp(3682708971.9060354 s since 1904-01-01), timestamp(3682708972.2345 s since 1904-01-01), timestamp(3682708972.5527015 s since 1904-01-01), timestamp(3682708972.8548064 s since 1904-01-01), timestamp(3682708973.582567 s since 1904-01-01), timestamp(3682708973.8891873 s since 1904-01-01), timestamp(3682708974.1884327 s since 1904-01-01), timestamp(3682708974.5010185 s since 1904-01-01), timestamp(3682708974.8142066 s since 1904-01-01), timestamp(3682708975.1175103 s since 1904-01-01), timestamp(3682708975.4374647 s since 1904-01-01), timestamp(3682708975.7527 s since 1904-01-01), timestamp(3682708976.0583982 s since 1904-01-01), timestamp(3682708976.3644648 s since 1904-01-01), timestamp(3682708976.689261 s since 1904-01-01), timestamp(3682708977.0021367 s since 1904-01-01), timestamp(3682708977.3057 s since 1904-01-01), timestamp(3682708977.6422114 s since 1904-01-01), timestamp(3682708977.9607697 s since 1904-01-01), timestamp(3682708978.2889266 s since 1904-01-01), timestamp(3682708978.7650247 s since 1904-01-01)], "DataArray"=[0.12705548027836072, 0.09285897110907357, 0.10206572350481419, 0.11587585224461763, 0.10666909978290509, 0.11456060191918477, 0.10272334874086991, 0.10403859909462224, 0.11784872780525776, 0.1349469823940256, 0.10929960051338994, 0.09351659627597492, 0.08891322004336702]}, {"TimeArray"=[timestamp(3682708934.7497134 s since 1904-01-01), timestamp(3682708935.064348 s since 1904-01-01), timestamp(3682708935.3896832 s since 1904-01-01), timestamp(3682708935.7026334 s since 1904-01-01), timestamp(3682708936.0021167 s since 1904-01-01), timestamp(3682708936.3049774 s since 1904-01-01), timestamp(3682708936.605407 s since 1904-01-01), timestamp(3682708936.903053 s since 1904-01-01), timestamp(3682708937.3067694 s since 1904-01-01), timestamp(3682708937.611465 s since 1904-01-01), timestamp(3682708937.909672 s since 1904-01-01), timestamp(3682708938.228514 s since 1904-01-01), timestamp(3682708938.527811 s since 1904-01-01), timestamp(3682708938.931336 s since 1904-01-01), timestamp(3682708940.012947 s since 1904-01-01), timestamp(3682708940.32849 s since 1904-01-01), timestamp(3682708940.631708 s since 1904-01-01), timestamp(3682708940.946489 s since 1904-01-01), timestamp(3682708941.244303 s since 1904-01-01), timestamp(3682708941.542656 s since 1904-01-01), timestamp(3682708941.8474927 s since 1904-01-01), timestamp(3682708942.3104415 s since 1904-01-01), timestamp(3682708942.6136575 s since 1904-01-01), timestamp(3682708942.916794 s since 1904-01-01), timestamp(3682708943.238447 s since 1904-01-01), timestamp(3682708943.5371313 s since 1904-01-01), timestamp(3682708943.857245 s since 1904-01-01), timestamp(3682708944.1856494 s since 1904-01-01), timestamp(3682708944.4866023 s since 1904-01-01), timestamp(3682708944.805397 s since 1904-01-01), timestamp(3682708945.111448 s since 1904-01-01), timestamp(3682708945.435288 s since 1904-01-01), timestamp(3682708945.7333007 s since 1904-01-01), timestamp(3682708946.0530386 s since 1904-01-01), timestamp(3682708946.4366784 s since 1904-01-01), timestamp(3682708946.732824 s since 1904-01-01), timestamp(3682708947.0537186 s since 1904-01-01), timestamp(3682708947.3846655 s since 1904-01-01), timestamp(3682708947.712872 s since 1904-01-01), timestamp(3682708948.0188503 s since 1904-01-01), timestamp(3682708948.737391 s since 1904-01-01), timestamp(3682708949.201587 s since 1904-01-01), timestamp(3682708949.502657 s since 1904-01-01), timestamp(3682708949.805978 s since 1904-01-01), timestamp(3682708950.1212378 s since 1904-01-01), timestamp(3682708950.4333377 s since 1904-01-01), timestamp(3682708950.732243 s since 1904-01-01), timestamp(3682708951.1057153 s since 1904-01-01), timestamp(3682708951.4068193 s since 1904-01-01), timestamp(3682708951.8357983 s since 1904-01-01), timestamp(3682708952.143476 s since 1904-01-01), timestamp(3682708952.4476566 s since 1904-01-01), timestamp(3682708952.7855697 s since 1904-01-01), timestamp(3682708953.086301 s since 1904-01-01), timestamp(3682708953.4027033 s since 1904-01-01), timestamp(3682708953.706577 s since 1904-01-01), timestamp(3682708954.023016 s since 1904-01-01), timestamp(3682708954.330558 s since 1904-01-01), timestamp(3682708954.643428 s since 1904-01-01), timestamp(3682708955.050496 s since 1904-01-01), timestamp(3682708955.3527017 s since 1904-01-01), timestamp(3682708955.7328424 s since 1904-01-01), timestamp(3682708956.0574985 s since 1904-01-01), timestamp(3682708956.3904 s since 1904-01-01), timestamp(3682708956.7025185 s since 1904-01-01), timestamp(3682708957.032419 s since 1904-01-01), timestamp(3682708957.351427 s since 1904-01-01), timestamp(3682708957.6656775 s since 1904-01-01), timestamp(3682708958.051097 s since 1904-01-01), timestamp(3682708958.4033985 s since 1904-01-01), timestamp(3682708958.7021422 s since 1904-01-01), timestamp(3682708959.004737 s since 1904-01-01), timestamp(3682708959.3058767 s since 1904-01-01), timestamp(3682708959.6056495 s since 1904-01-01), timestamp(3682708959.9347386 s since 1904-01-01), timestamp(3682708960.252382 s since 1904-01-01), timestamp(3682708960.553459 s since 1904-01-01), timestamp(3682708960.8641214 s since 1904-01-01), timestamp(3682708961.160152 s since 1904-01-01), timestamp(3682708961.487622 s since 1904-01-01), timestamp(3682708961.788169 s since 1904-01-01), timestamp(3682708962.0896144 s since 1904-01-01), timestamp(3682708962.406388 s since 1904-01-01), timestamp(3682708962.70866 s since 1904-01-01), timestamp(3682708963.033897 s since 1904-01-01), timestamp(3682708963.3512735 s since 1904-01-01), timestamp(3682708963.668318 s since 1904-01-01), timestamp(3682708963.9877753 s since 1904-01-01), timestamp(3682708964.2907033 s since 1904-01-01), timestamp(3682708964.606549 s since 1904-01-01), timestamp(3682708964.906368 s since 1904-01-01), timestamp(3682708965.217731 s since 1904-01-01), timestamp(3682708965.5397863 s since 1904-01-01), timestamp(3682708965.8690424 s since 1904-01-01), timestamp(3682708966.190765 s since 1904-01-01), timestamp(3682708966.5023417 s since 1904-01-01), timestamp(3682708966.806744 s since 1904-01-01), timestamp(3682708967.1092105 s since 1904-01-01), timestamp(3682708967.406003 s since 1904-01-01), timestamp(3682708967.710469 s since 1904-01-01), timestamp(3682708968.041528 s since 1904-01-01), timestamp(3682708968.365668 s since 1904-01-01), timestamp(3682708968.8523655 s since 1904-01-01), timestamp(3682708969.1540494 s since 1904-01-01), timestamp(3682708969.4895535 s since 1904-01-01), timestamp(3682708969.7907286 s since 1904-01-01), timestamp(3682708970.105831 s since 1904-01-01), timestamp(3682708970.4602976 s since 1904-01-01), timestamp(3682708970.963533 s since 1904-01-01), timestamp(3682708971.301882 s since 1904-01-01), timestamp(3682708971.6079335 s since 1904-01-01), timestamp(3682708971.9060354 s since 1904-01-01), timestamp(3682708972.2345 s since 1904-01-01), timestamp(3682708972.5527015 s since 1904-01-01), timestamp(3682708972.8548064 s since 1904-01-01), timestamp(3682708973.582567 s since 1904-01-01), timestamp(3682708973.8891873 s since 1904-01-01), timestamp(3682708974.1884327 s since 1904-01-01), timestamp(3682708974.5010185 s since 1904-01-01), timestamp(3682708974.8142066 s since 1904-01-01), timestamp(3682708975.1175103 s since 1904-01-01), timestamp(3682708975.4374647 s since 1904-01-01), timestamp(3682708975.7527 s since 1904-01-01), timestamp(3682708976.0583982 s since 1904-01-01), timestamp(3682708976.3644648 s since 1904-01-01), timestamp(3682708976.689261 s since 1904-01-01), timestamp(3682708977.0021367 s since 1904-01-01), timestamp(3682708977.3057 s since 1904-01-01), timestamp(3682708977.6422114 s since 1904-01-01), timestamp(3682708977.9607697 s since 1904-01-01), timestamp(3682708978.2889266 s since 1904-01-01), timestamp(3682708978.7650247 s since 1904-01-01)], "DataArray"=[0.12442497956407811, 0.11193010123700953, 0.123109729251026, 0.13691985794157618, 0.11850635302256154, 0.10929960052518167, 0.13100123135211023, 0.1500723614418107, 0.10601147463141988, 0.14152323415016094, 0.16190961461275455, 0.10535384946395471, 0.09943522287031531]}, {"TimeArray"=[timestamp(3682708934.7497134 s since 1904-01-01), timestamp(3682708935.064348 s since 1904-01-01), timestamp(3682708935.3896832 s since 1904-01-01), timestamp(3682708935.7026334 s since 1904-01-01), timestamp(3682708936.0021167 s since 1904-01-01), timestamp(3682708936.3049774 s since 1904-01-01), timestamp(3682708936.605407 s since 1904-01-01), timestamp(3682708936.903053 s since 1904-01-01), timestamp(3682708937.3067694 s since 1904-01-01), timestamp(3682708937.611465 s since 1904-01-01), timestamp(3682708937.909672 s since 1904-01-01), timestamp(3682708938.228514 s since 1904-01-01), timestamp(3682708938.527811 s since 1904-01-01), timestamp(3682708938.931336 s since 1904-01-01), timestamp(3682708940.012947 s since 1904-01-01), timestamp(3682708940.32849 s since 1904-01-01), timestamp(3682708940.631708 s since 1904-01-01), timestamp(3682708940.946489 s since 1904-01-01), timestamp(3682708941.244303 s since 1904-01-01), timestamp(3682708941.542656 s since 1904-01-01), timestamp(3682708941.8474927 s since 1904-01-01), timestamp(3682708942.3104415 s since 1904-01-01), timestamp(3682708942.6136575 s since 1904-01-01), timestamp(3682708942.916794 s since 1904-01-01), timestamp(3682708943.238447 s since 1904-01-01), timestamp(3682708943.5371313 s since 1904-01-01), timestamp(3682708943.857245 s since 1904-01-01), timestamp(3682708944.1856494 s since 1904-01-01), timestamp(3682708944.4866023 s since 1904-01-01), timestamp(3682708944.805397 s since 1904-01-01), timestamp(3682708945.111448 s since 1904-01-01), timestamp(3682708945.435288 s since 1904-01-01), timestamp(3682708945.7333007 s since 1904-01-01), timestamp(3682708946.0530386 s since 1904-01-01), timestamp(3682708946.4366784 s since 1904-01-01), timestamp(3682708946.732824 s since 1904-01-01), timestamp(3682708947.0537186 s since 1904-01-01), timestamp(3682708947.3846655 s since 1904-01-01), timestamp(3682708947.712872 s since 1904-01-01), timestamp(3682708948.0188503 s since 1904-01-01), timestamp(3682708948.737391 s since 1904-01-01), timestamp(3682708949.201587 s since 1904-01-01), timestamp(3682708949.502657 s since 1904-01-01), timestamp(3682708949.805978 s since 1904-01-01), timestamp(3682708950.1212378 s since 1904-01-01), timestamp(3682708950.4333377 s since 1904-01-01), timestamp(3682708950.732243 s since 1904-01-01), timestamp(3682708951.1057153 s since 1904-01-01), timestamp(3682708951.4068193 s since 1904-01-01), timestamp(3682708951.8357983 s since 1904-01-01), timestamp(3682708952.143476 s since 1904-01-01), timestamp(3682708952.4476566 s since 1904-01-01), timestamp(3682708952.7855697 s since 1904-01-01), timestamp(3682708953.086301 s since 1904-01-01), timestamp(3682708953.4027033 s since 1904-01-01), timestamp(3682708953.706577 s since 1904-01-01), timestamp(3682708954.023016 s since 1904-01-01), timestamp(3682708954.330558 s since 1904-01-01), timestamp(3682708954.643428 s since 1904-01-01), timestamp(3682708955.050496 s since 1904-01-01), timestamp(3682708955.3527017 s since 1904-01-01), timestamp(3682708955.7328424 s since 1904-01-01), timestamp(3682708956.0574985 s since 1904-01-01), timestamp(3682708956.3904 s since 1904-01-01), timestamp(3682708956.7025185 s since 1904-01-01), timestamp(3682708957.032419 s since 1904-01-01), timestamp(3682708957.351427 s since 1904-01-01), timestamp(3682708957.6656775 s since 1904-01-01), timestamp(3682708958.051097 s since 1904-01-01), timestamp(3682708958.4033985 s since 1904-01-01), timestamp(3682708958.7021422 s since 1904-01-01), timestamp(3682708959.004737 s since 1904-01-01), timestamp(3682708959.3058767 s since 1904-01-01), timestamp(3682708959.6056495 s since 1904-01-01), timestamp(3682708959.9347386 s since 1904-01-01), timestamp(3682708960.252382 s since 1904-01-01), timestamp(3682708960.553459 s since 1904-01-01), timestamp(3682708960.8641214 s since 1904-01-01), timestamp(3682708961.160152 s since 1904-01-01), timestamp(3682708961.487622 s since 1904-01-01), timestamp(3682708961.788169 s since 1904-01-01), timestamp(3682708962.0896144 s since 1904-01-01), timestamp(3682708962.406388 s since 1904-01-01), timestamp(3682708962.70866 s since 1904-01-01), timestamp(3682708963.033897 s since 1904-01-01), timestamp(3682708963.3512735 s since 1904-01-01), timestamp(3682708963.668318 s since 1904-01-01), timestamp(3682708963.9877753 s since 1904-01-01), timestamp(3682708964.2907033 s since 1904-01-01), timestamp(3682708964.606549 s since 1904-01-01), timestamp(3682708964.906368 s since 1904-01-01), timestamp(3682708965.217731 s since 1904-01-01), timestamp(3682708965.5397863 s since 1904-01-01), timestamp(3682708965.8690424 s since 1904-01-01), timestamp(3682708966.190765 s since 1904-01-01), timestamp(3682708966.5023417 s since 1904-01-01), timestamp(3682708966.806744 s since 1904-01-01), timestamp(3682708967.1092105 s since 1904-01-01), timestamp(3682708967.406003 s since 1904-01-01), timestamp(3682708967.710469 s since 1904-01-01), timestamp(3682708968.041528 s since 1904-01-01), timestamp(3682708968.365668 s since 1904-01-01), timestamp(3682708968.8523655 s since 1904-01-01), timestamp(3682708969.1540494 s since 1904-01-01), timestamp(3682708969.4895535 s since 1904-01-01), timestamp(3682708969.7907286 s since 1904-01-01), timestamp(3682708970.105831 s since 1904-01-01), timestamp(3682708970.4602976 s since 1904-01-01), timestamp(3682708970.963533 s since 1904-01-01), timestamp(3682708971.301882 s since 1904-01-01), timestamp(3682708971.6079335 s since 1904-01-01), timestamp(3682708971.9060354 s since 1904-01-01), timestamp(3682708972.2345 s since 1904-01-01), timestamp(3682708972.5527015 s since 1904-01-01), timestamp(3682708972.8548064 s since 1904-01-01), timestamp(3682708973.582567 s since 1904-01-01), timestamp(3682708973.8891873 s since 1904-01-01), timestamp(3682708974.1884327 s since 1904-01-01), timestamp(3682708974.5010185 s since 1904-01-01), timestamp(3682708974.8142066 s since 1904-01-01), timestamp(3682708975.1175103 s since 1904-01-01), timestamp(3682708975.4374647 s since 1904-01-01), timestamp(3682708975.7527 s since 1904-01-01), timestamp(3682708976.0583982 s since 1904-01-01), timestamp(3682708976.3644648 s since 1904-01-01), timestamp(3682708976.689261 s since 1904-01-01), timestamp(3682708977.0021367 s since 1904-01-01), timestamp(3682708977.3057 s since 1904-01-01), timestamp(3682708977.6422114 s since 1904-01-01), timestamp(3682708977.9607697 s since 1904-01-01), timestamp(3682708978.2889266 s since 1904-01-01), timestamp(3682708978.7650247 s since 1904-01-01)], "DataArray"=[0.16256723973563597, 0.19150274749818202, 0.1842688705024636, 0.1559909879764779, 0.1987366243890375, 0.18098074469775668, 0.18755699642782248, 0.1849264957434181, 0.1921603726689468, 0.14283848451544143, 0.14481136006437864, 0.1928179978537674, 0.20728575167685398]}] caption="XY Graph"
  in  "log/linear 4":bool
  in  "log/linear 3":bool
  out "Fill (false)":bool=TRUE
  in  "Fill state":bool
  out "state 1 (false)":bool=TRUE
  out "state 1":bool
  out "state 2":bool
  out "state 2 (false)":bool=TRUE
  out "Status V2 CTRL":enum16{"Pressurize", "Release"}(ring)
  out "Status V1 CTRL":enum16{"Pressurize", "Release"}(ring)
  out "Lav (%)":dbl=-49199.19854911039 format="%0.2f"
  out "Lstd":dbl=554.7391446242465 format="%0.2f"
  out "Last N M.A. Levels":dbl[](array[numeric]) format="%_5e"
  out "Lstd history":dbl(graph)=554.7391446242465
  out "Lav history":dbl(graph)=-49199.19854911039
  out "Target Index (L)":i32=6
  in  "Auto Fll\nHe level label":string="P_Dewar"
  out "Target Index (P)":i32=6
  in  "Auto Fll\nDewar P. label":string="P_Dewar"
  out "He Level":T8(graph) caption="XY Graph"
  in  "P_safelimit_high (Pa)":dbl=300000.0 format="%_4e"
  in  "P_safelimit_low (Pa)":dbl=100.0 format="%_4e"
  in  "Auto Fill ON?":bool
  out "Pstd history":dbl(graph)=554.7391446242465
  out "Pav history":dbl(graph)=-49199.19854911039
  in  "Mov. Avg Interval":i64=4
  in  "V2 (N.C.)":bool
  in  "V1 (N.O.)":bool=TRUE
  in  "N for sampling":i64=7
  in  "L_low (%)":dbl=5000.0 format="%_3f"
  in  "L_high (%)":dbl=5000.0 format="%_3g"
  in  "P_2_low (Pa)":dbl=103000.0 format="%_4e"
  in  "P_1_low (Pa)":dbl=125000.0 format="%_4g"
  in  "P_2_high (Pa)":dbl=120000.0 format="%_4e"
  in  "P_1_high (Pa)":dbl=130000.0 format="%_4e"
  out "Dewar Pressure":T8(graph) caption="XY Graph"
  out "Last N M.A. Pressures":dbl[](array[numeric]) format="%_5e"
  out "Pav (Pa)":dbl=-49199.19854911039 format="%0.4e"
  out "Pstd":dbl=554.7391446242465 format="%0.4e"
  out "File Refn DewarCTRL":refnum<file>
  out "Error Out (Dewar CTRL":errorcluster
  in  "update current":bool
  out "USB AOUT":dbl[](array[numeric])=[0.18461538461538463, 0.07461374136817528]
  out "Monitor Current (mA)":dbl=0.02085221832695692 min=0.0 max=1.9 format="%_4e"
  out "Graph 7":T9(graph)=[{"TimeArray (USB6218)"=[timestamp(3682708962.51632 s since 1904-01-01), timestamp(3682708963.924918 s since 1904-01-01), timestamp(3682708968.4155784 s since 1904-01-01), timestamp(3682708968.847412 s since 1904-01-01), timestamp(3682708970.9545894 s since 1904-01-01)], "DataArrayConv (USB6218)"=[]}, {"TimeArray (USB6218)"=[], "DataArrayConv (USB6218)"=[]}] caption="XY Graph"
  in  "upper limit (V)\n (Kikusui)":dbl=20.0 format="%_3f"
  in  "lower limit (V) \n(Kikusui)":dbl format="%_3f"
  in  "lower limit (mA) \n(Kikusui)":dbl=4.0 format="%_3f"
  in  "upper limit (mA)\n (Kikusui)":dbl=20.0 format="%_3f"
  in  "lower limit (mA)":dbl=4.0 format="%_3f"
  in  "SetCurrent 2 (mA)":dbl=8.0 format="%_3f"
  in  "upper limit (mA)":dbl=20.0 format="%_3f"
  out "error out (KIKUSI CTRL)":errorcluster
  out "ActualVoltage (V)":dbl[](array[numeric]) format="%_6g"
  out "ActualCurrent (A)":dbl[](array[numeric])=[0.004, 0.008] format="%_3e"
  in  "SetCurrent 1 (mA)":dbl=3.9999999999999996 format="%_3g"
  in  "Output\n (ADCMT)":bool[](array[boolean])=[FALSE, FALSE]
  out "error out (ADCMT6420A)":errorcluster
  in  "Voltage limits (V)":dbl[](array[numeric])=[12.0, 12.0] format="%_3f"
  in  "CtrlLabels":string[](array[string])=["CV2", "CV3"]
  in  "VISA":refnum<visa-resource-name>[](array[refnum])=["GPIB0::1::INSTR", "GPIB0::12::INSTR"]
  out "Initialized?":bool=TRUE
  in  "InstName":string="ADCMT"
  out "Graph 6":T8(graph)=[{"TimeArray"=[timestamp(3682708948.680192 s since 1904-01-01), timestamp(3682708950.913432 s since 1904-01-01), timestamp(3682708951.411795 s since 1904-01-01), timestamp(3682708954.6659913 s since 1904-01-01), timestamp(3682708955.4113503 s since 1904-01-01), timestamp(3682708957.6849513 s since 1904-01-01), timestamp(3682708958.090539 s since 1904-01-01)], "Filtered X"=[0.004, 0.004, 0.004, 0.0041, 0.004, 0.004, 0.004]}, {"TimeArray"=[timestamp(3682708948.680192 s since 1904-01-01), timestamp(3682708950.913432 s since 1904-01-01), timestamp(3682708951.411795 s since 1904-01-01), timestamp(3682708954.6659913 s since 1904-01-01), timestamp(3682708955.4113503 s since 1904-01-01), timestamp(3682708957.6849513 s since 1904-01-01), timestamp(3682708958.090539 s since 1904-01-01)], "Filtered X"=[0.008, 0.008, 0.008, 0.008, 0.008, 0.0081, 0.008]}, {"TimeArray"=[timestamp(3682708948.680192 s since 1904-01-01), timestamp(3682708950.913432 s since 1904-01-01), timestamp(3682708951.411795 s since 1904-01-01), timestamp(3682708954.6659913 s since 1904-01-01), timestamp(3682708955.4113503 s since 1904-01-01), timestamp(3682708957.6849513 s since 1904-01-01), timestamp(3682708958.090539 s since 1904-01-01)], "Filtered X"=[0.004, 0.004, 0.004, 0.0040999999999999995, 0.003999999999999999, 0.003999999999999999, 0.003999999999999999]}, {"TimeArray"=[timestamp(3682708948.680192 s since 1904-01-01), timestamp(3682708950.913432 s since 1904-01-01), timestamp(3682708951.411795 s since 1904-01-01), timestamp(3682708954.6659913 s since 1904-01-01), timestamp(3682708955.4113503 s since 1904-01-01), timestamp(3682708957.6849513 s since 1904-01-01), timestamp(3682708958.090539 s since 1904-01-01)], "Filtered X"=[0.008, 0.008, 0.008, 0.008, 0.008, 0.0081, 0.008]}] caption="XY Graph"
  in  "Initialize":bool
  in  "CONTROL KIKUSUI?":bool=TRUE
  in  "OUTPUT\n(Kikusui)":bool
  in  "Set Voltage (V)\n (Kikusui)":dbl=12.0 min=0.0 max=49.0 format="%_3g"
  in  "Set Current (mA)\n (Kikusui)":dbl=4.99 min=0.0 max=1.9 format="%_3g"
  out "Series 1":string[](array[string])=["P_Dewar"]
  out "Series 2":string[](array[string])=["T4He6", "T4He9", "T3He1-2", "T3He1-3", "T4He7", "T4He8", "T4He10", "T1K6", "TIP1", "N.C.", "TIP2", "T1K3-1", "T1K3-2", "T3He5", "T3He8", "T3He6-1", "T3He6-2", "T3He7-1", "T3He7-2"]
  out "Series 3":string[](array[string])=["P_ins", "P_4Kres", "P_3HeIN", "P_SldRTN", "P_3Hepot", "P_1Kpot", "DP_HEX4", "DP_HEX5", "F_1", "F_2", "F_3", "F_4", "F_5", "I_CV"]
  out "Series 4":string[](array[string])=["L1", "L2-1", "L2-2", "L3"]
  out "Plot errors":errorcluster
  out "LastMeasurementConfig (218)":T10(array[cluster])=[{"LSIName"="LSI218A", "Active?"=TRUE, "LastData"=[284.43, 290.03, 243.23, 256.15, 171.54, 180.77, 63.049, 117.3], "Labels"=["T3He10", "T3He1-1", "TTH3", "TTH4", "TTH1", "TTH2", "T4He1", "T1K1"]}, {"LSIName"="LSI218B", "Active?"=TRUE, "LastData"=[30.0, 0.0, 0.0, 0.0, 202.72, 191.34, 122.93, 289.61], "Labels"=["N.C.", "N.C.", "N.C.", "N.C.", "T3He2-1", "T3He2-2", "T3He3", "T3He1-4"]}, {"LSIName"="LSI218C", "Active?"=TRUE, "LastData"=[292.19, 292.34, 291.95, 292.02, 202.48, 197.55, 192.92, 186.55], "Labels"=["T4He3-1", "T4He3-2", "T4He3-3", "T4He3-4", "T4He2-1", "T4He2-2", "T4He4", "T4He5"]}, {"LSIName"="LSI218D", "Active?"=TRUE, "LastData"=[192.44, 234.78, 290.18, 290.03, 246.41, 271.83, 269.02, 283.26], "Labels"=["T4He6", "T4He9", "T3He1-2", "T3He1-3", "T4He7", "T4He8", "T4He10", "T1K6"]}, {"LSIName"="LSI218E", "Active?"=TRUE, "LastData"=[278.46, 0.0, 229.12, 688.49, 197.75, 114.09, 159.57, 688.58], "Labels"=["TIP1", "N.C.", "TIP2", "N.C.", "TIP3", "TIP4", "TIP5", "N.C."]}, {"LSIName"="LSI218F", "Active?"=TRUE, "LastData"=[121.27, 92.631, 95.353, 144.45, 121.36, 152.88, 0.433, 0.0], "Labels"=["T1K2", "T1K4", "T1K5", "T3He4", "T3He9", "TIP6", "N.C.", "N.C."]}]
  out "DataArrayConv (USB6210)":dbl[][](array[numeric])=[[0.0002837964904784882, 101600.30460296334, 101095.46568969214, 101019.82210515348, 101192.28771374167, 101379.03896406938, 102202.16534140152, -11.509692262573202, 72.86987407092438, 100.06505169937662, 0.12705548027836072, 0.12442497956407811, 0.16256723973563597], [0.0002540201950280979, 101869.9905464041, 101508.2167090379, 100756.71389319496, 101087.95251115608, 101496.52568286558, 100161.43201016451, -12.389448520230106, 123.51753179896008, 100.0913578166008, 0.09285897110907357, 0.11193010123700953, 0.19150274749818202], [0.00028482974060555643, 101809.14675876396, 101118.48766948337, 100758.35831891237, 101239.63309866226, 101521.95190753773, 100789.60275186355, -10.465495581526152, 76.81644379327834, 100.07097057589947, 0.10206572350481419, 0.123109729251026, 0.1842688705024636], [0.00027860177910337677, 101866.70169750709, 101185.90913147827, 100815.91325088433, 101173.87561233125, 101470.22268162873, 100345.60782032329, -10.98348292447815, 90.30056156572597, 100.0722858814967, 0.11587585224461763, 0.13691985794157618, 0.1559909879764779], [0.00024577167564576887, 101715.41444453571, 101085.59913013777, 101031.33307660364, 101180.01298304915, 101378.16219418835, 102337.00779239179, -12.167453922019956, 121.54424751544268, 100.04006088884337, 0.10666909978290509, 0.11850635302256154, 0.1987366243890375], [0.00029394366732651253, 101618.39327990329, 101149.73175900572, 101074.08816587094, 101127.40699909146, 101448.30351791858, 101526.30582974949, -10.235278919276947, 74.18539764095011, 100.09201547031509, 0.11456060191918477, 0.10929960052518167, 0.18098074469775668], [0.00030975494520513706, 101695.68133206986, 100738.62519308273, 100784.66913064543, 101330.81680668671, 101438.65908252355, 102083.76617517172, -11.31236370510344, 99.01590690954754, 100.04006088897802, 0.10272334874086991, 0.13100123135211023, 0.18755699642782248], [0.0002726750992747204, 101738.43641408093, 100944.17848178797, 100957.33387783177, 101234.37249974646, 101339.58446725098, 102660.95994909719, -9.659737486239134, 145.881434544608, 100.01375477333622, 0.10403859909462224, 0.1500723614418107, 0.1849264957434181], [0.00027004531380478555, 101822.30217884819, 101235.24192488367, 100883.33470382096, 101158.09381800564, 101479.86711402163, 100931.02351867667, -13.770748002328748, 77.47420657495452, 100.06833996442191, 0.11784872780525776, 0.10601147463141988, 0.1921603726689468], [0.0003241508978015368, 101746.6585576296, 100873.46815027227, 101042.84406634107, 101257.16842432228, 101414.1096273334, 101384.88517891317, -9.963952281609956, 66.29225573632547, 100.05058333549653, 0.1349469823940256, 0.14152323415016094, 0.14283848451544143], [0.000280464221899836, 101662.79279490249, 100758.35831878404, 101144.79847670182, 101282.59464790425, 101304.51381340383, 103307.21992056293, -10.095504639094866, 159.8588737296336, 100.01441242568171, 0.10929960051338994, 0.16190961461275455, 0.14481136006437864], [0.00024786464375754834, 101753.23625632537, 101259.90832448212, 100843.86847527634, 101144.9423243698, 101432.52171747175, 101878.21277938908, -13.458311205900852, 115.45995143998233, 100.06899761748156, 0.09351659627597492, 0.10535384946395471, 0.1928179978537674], [0.0002743317218481517, 101804.21347256108, 101213.86438690027, 100769.8692892141, 101177.38268030914, 101501.78627352713, 100806.04675539682, -14.214737121827303, 66.62113679397174, 100.07688945274376, 0.08891322004336702, 0.09943522287031531, 0.20728575167685398]]
  out "LastMeasurementConfig (336)":T10(array[cluster])=[{"LSIName"="LSi336X", "Active?"=TRUE, "LastData"=[94.5454, 94.3475, 128.374, 133.795], "Labels"=["T1K3-1", "T1K3-2", "T3He5", "T3He8"]}, {"LSIName"="LSi336Y", "Active?"=TRUE, "LastData"=[135.029, 135.063, 134.969, 134.048], "Labels"=["T3He6-1", "T3He6-2", "T3He7-1", "T3He7-2"]}]
  out "DataArrayConv (USB6218)":dbl[][](array[numeric])=[[11.964438420500317, 0.05384606242159112, 0.10908259391557279, -8.499381084067222, 30.55744634457672, -0.002496639642160084, -25.00169101514697], [11.408785269374608, 0.23007690082860877, 0.14853725930302558, -8.696654424159398, 31.129538854122675, -0.0027597253671516027, -24.99347129318512], [11.68825578939364, 0.17484036946958043, 0.06962792873490953, -8.6802149789511, 30.912538247690556, -0.003943611132105104, -25.010732709300708], [11.632361685392253, 0.12617961563309327, 0.21297987945254448, -9.433141566395845, 30.504840138158723, -0.0011154395877097905, -25.01813045908033], [11.329875946073106, 0.08409463913321968, 0.3221377861789966, -8.995852325758753, 30.78102272877803, -0.0032201253887054583, -24.987717487820795], [11.03725387078261, 0.14985241499203045, 0.29714983142290685, -9.087913218234108, 30.32400629791559, -0.0033516682500984328, -25.00415693173725], [11.405497381010084, 0.10908259417261384, 0.1998283241116452, -8.693366535056605, 30.682386088917767, -0.0030885825294485274, -25.00004707075572], [11.34631538832425, 0.2392829894580274, 0.273477032626091, -8.884064098182353, 31.192008726064962, 0.02144416120447479, -25.007444820519524], [11.671816348179764, 0.4089380490601221, 0.039379351999432544, -8.729533314447908, 30.33058207439542, 0.02118107548098528, -24.981963682453948], [11.786892442144707, 0.23796783348741785, 0.20508894555251794, -8.598017754623585, 30.73499229600657, 0.02624547563560286, -24.9794977658719], [12.122257066147943, 0.14064632601173044, 0.13801601525091467, -8.354713967474565, 31.086796311382603, 0.019931418304363107, -24.995937209783964], [11.60277068731648, 0.002554997645770496, 0.24322845562137518, -9.33121700612929, 30.432506602377853, 0.020062961151207755, -25.00826679273129], [11.53043714284093, 0.151167570083921, 0.13538570442875797, -9.35423222985425, 30.863219928706915, 0.020917989763440756, -24.994293265386126]]
  out "TimeArray (USB6218)":timestamp[](array[timestamp])=[timestamp(3682708934.7457247 s since 1904-01-01), timestamp(3682708935.05737 s since 1904-01-01), timestamp(3682708935.381696 s since 1904-01-01), timestamp(3682708935.6976466 s since 1904-01-01), timestamp(3682708935.997305 s since 1904-01-01), timestamp(3682708936.298069 s since 1904-01-01), timestamp(3682708936.598516 s since 1904-01-01), timestamp(3682708936.898253 s since 1904-01-01), timestamp(3682708937.3017807 s since 1904-01-01), timestamp(3682708937.603601 s since 1904-01-01), timestamp(3682708937.9028106 s since 1904-01-01), timestamp(3682708938.2214966 s since 1904-01-01), timestamp(3682708938.523822 s since 1904-01-01), timestamp(3682708938.9273815 s since 1904-01-01), timestamp(3682708940.0082703 s since 1904-01-01), timestamp(3682708940.3241343 s since 1904-01-01), timestamp(3682708940.6267815 s since 1904-01-01), timestamp(3682708940.939516 s since 1904-01-01), timestamp(3682708941.239446 s since 1904-01-01), timestamp(3682708941.538666 s since 1904-01-01), timestamp(3682708941.840121 s since 1904-01-01), timestamp(3682708942.306481 s since 1904-01-01), timestamp(3682708942.607712 s since 1904-01-01), timestamp(3682708942.9108286 s since 1904-01-01), timestamp(3682708943.2304735 s since 1904-01-01), timestamp(3682708943.5302224 s since 1904-01-01), timestamp(3682708943.862504 s since 1904-01-01), timestamp(3682708944.178786 s since 1904-01-01), timestamp(3682708944.479564 s since 1904-01-01), timestamp(3682708944.7974215 s since 1904-01-01), timestamp(3682708945.1064615 s since 1904-01-01), timestamp(3682708945.427227 s since 1904-01-01), timestamp(3682708945.7283096 s since 1904-01-01), timestamp(3682708946.0490494 s since 1904-01-01), timestamp(3682708946.43248 s since 1904-01-01), timestamp(3682708946.7368135 s since 1904-01-01), timestamp(3682708947.049049 s since 1904-01-01), timestamp(3682708947.3797193 s since 1904-01-01), timestamp(3682708947.7079344 s since 1904-01-01), timestamp(3682708948.0078607 s since 1904-01-01), timestamp(3682708948.730386 s since 1904-01-01), timestamp(3682708949.194605 s since 1904-01-01), timestamp(3682708949.4966736 s since 1904-01-01), timestamp(3682708949.799 s since 1904-01-01), timestamp(3682708950.114288 s since 1904-01-01), timestamp(3682708950.426346 s since 1904-01-01), timestamp(3682708950.7263794 s since 1904-01-01), timestamp(3682708951.0997186 s since 1904-01-01), timestamp(3682708951.3999505 s since 1904-01-01), timestamp(3682708951.8269634 s since 1904-01-01), timestamp(3682708952.1394343 s since 1904-01-01), timestamp(3682708952.4414854 s since 1904-01-01), timestamp(3682708952.7784295 s since 1904-01-01), timestamp(3682708953.081291 s since 1904-01-01), timestamp(3682708953.395766 s since 1904-01-01), timestamp(3682708953.6989856 s since 1904-01-01), timestamp(3682708954.018292 s since 1904-01-01), timestamp(3682708954.3266025 s since 1904-01-01), timestamp(3682708954.652079 s since 1904-01-01), timestamp(3682708955.043474 s since 1904-01-01), timestamp(3682708955.346717 s since 1904-01-01), timestamp(3682708955.7265873 s since 1904-01-01), timestamp(3682708956.049494 s since 1904-01-01), timestamp(3682708956.38338 s since 1904-01-01), timestamp(3682708956.6967216 s since 1904-01-01), timestamp(3682708957.0268736 s since 1904-01-01), timestamp(3682708957.344452 s since 1904-01-01), timestamp(3682708957.659692 s since 1904-01-01), timestamp(3682708958.0427456 s since 1904-01-01), timestamp(3682708958.395813 s since 1904-01-01), timestamp(3682708958.6971207 s since 1904-01-01), timestamp(3682708958.997812 s since 1904-01-01), timestamp(3682708959.299009 s since 1904-01-01), timestamp(3682708959.5986657 s since 1904-01-01), timestamp(3682708959.927756 s since 1904-01-01), timestamp(3682708960.2443895 s since 1904-01-01), timestamp(3682708960.5465074 s since 1904-01-01), timestamp(3682708960.8593345 s since 1904-01-01), timestamp(3682708961.1681266 s since 1904-01-01), timestamp(3682708961.48064 s since 1904-01-01), timestamp(3682708961.7831826 s since 1904-01-01), timestamp(3682708962.084628 s since 1904-01-01), timestamp(3682708962.400445 s since 1904-01-01), timestamp(3682708962.7008 s since 1904-01-01), timestamp(3682708963.0295024 s since 1904-01-01), timestamp(3682708963.3452177 s since 1904-01-01), timestamp(3682708963.6609526 s since 1904-01-01), timestamp(3682708963.9819894 s since 1904-01-01), timestamp(3682708964.284719 s since 1904-01-01), timestamp(3682708964.5991874 s since 1904-01-01), timestamp(3682708964.898812 s since 1904-01-01), timestamp(3682708965.212899 s since 1904-01-01), timestamp(3682708965.533695 s since 1904-01-01), timestamp(3682708965.8616786 s since 1904-01-01), timestamp(3682708966.184785 s since 1904-01-01), timestamp(3682708966.4963593 s since 1904-01-01), timestamp(3682708966.8002353 s since 1904-01-01), timestamp(3682708967.102233 s since 1904-01-01), timestamp(3682708967.4009976 s since 1904-01-01), timestamp(3682708967.702599 s since 1904-01-01), timestamp(3682708968.0344696 s since 1904-01-01), timestamp(3682708968.3587327 s since 1904-01-01), timestamp(3682708968.8484025 s since 1904-01-01), timestamp(3682708969.1487703 s since 1904-01-01), timestamp(3682708969.483566 s since 1904-01-01), timestamp(3682708969.7836742 s since 1904-01-01), timestamp(3682708970.0997343 s since 1904-01-01), timestamp(3682708970.456341 s since 1904-01-01), timestamp(3682708970.959581 s since 1904-01-01), timestamp(3682708971.294749 s since 1904-01-01), timestamp(3682708971.600965 s since 1904-01-01), timestamp(3682708971.9014745 s since 1904-01-01), timestamp(3682708972.230295 s since 1904-01-01), timestamp(3682708972.5446954 s since 1904-01-01), timestamp(3682708972.847607 s since 1904-01-01), timestamp(3682708973.5785775 s since 1904-01-01), timestamp(3682708973.883203 s since 1904-01-01), timestamp(3682708974.1835823 s since 1904-01-01), timestamp(3682708974.497029 s since 1904-01-01), timestamp(3682708974.808202 s since 1904-01-01), timestamp(3682708975.1124954 s since 1904-01-01), timestamp(3682708975.430429 s since 1904-01-01), timestamp(3682708975.7479105 s since 1904-01-01), timestamp(3682708976.0485106 s since 1904-01-01), timestamp(3682708976.3573728 s since 1904-01-01), timestamp(3682708976.6827016 s since 1904-01-01), timestamp(3682708976.9976544 s since 1904-01-01), timestamp(3682708977.297767 s since 1904-01-01), timestamp(3682708977.6352234 s since 1904-01-01), timestamp(3682708977.952658 s since 1904-01-01), timestamp(3682708978.2831464 s since 1904-01-01), timestamp(3682708978.761338 s since 1904-01-01)]
  out "Data Array sizes (6210)":i32[](array[numeric])=[13, 13]
  out "DataArraySize (6218)":i32[](array[numeric])=[13, 7]
  out "TimeArray size (6218)":i32=132
  out "TimeArray (LSI336)":timestamp[](array[timestamp])
  out "TimeArray Size (336)":i32
  out "DataArray (336)":dbl[][](array[numeric])
  out "DataArray size (336)":i32[](array[numeric])
  # "GLOBAL STATUS/CONTROL"
  # "USB6210 Analog inputs Settings"
  # "USB6218 Analog inputs Settings"
  # "USB6218 Digital Output Settings"
  # "USB6218 Analog Output Settings"
  # "Global Settings"
  # "LSI218 Settings"
  # "LSI336 Settings"
  # "Graph screenshots"
  # "Configuration"
  # "Activated only when *FIll state* = TRUE"
  # "Activated only when *FIll state* = TRUE"
  # "Vavle Status"
  # "OPEN"
  # "CLOSED"
  # "ADCMT6240A Control/Status"
  # "ADCMT6240A Initialization"
  # "Set Currents (mA)"
  # "KIKUSUI PWR400H CTRL via USB6218"
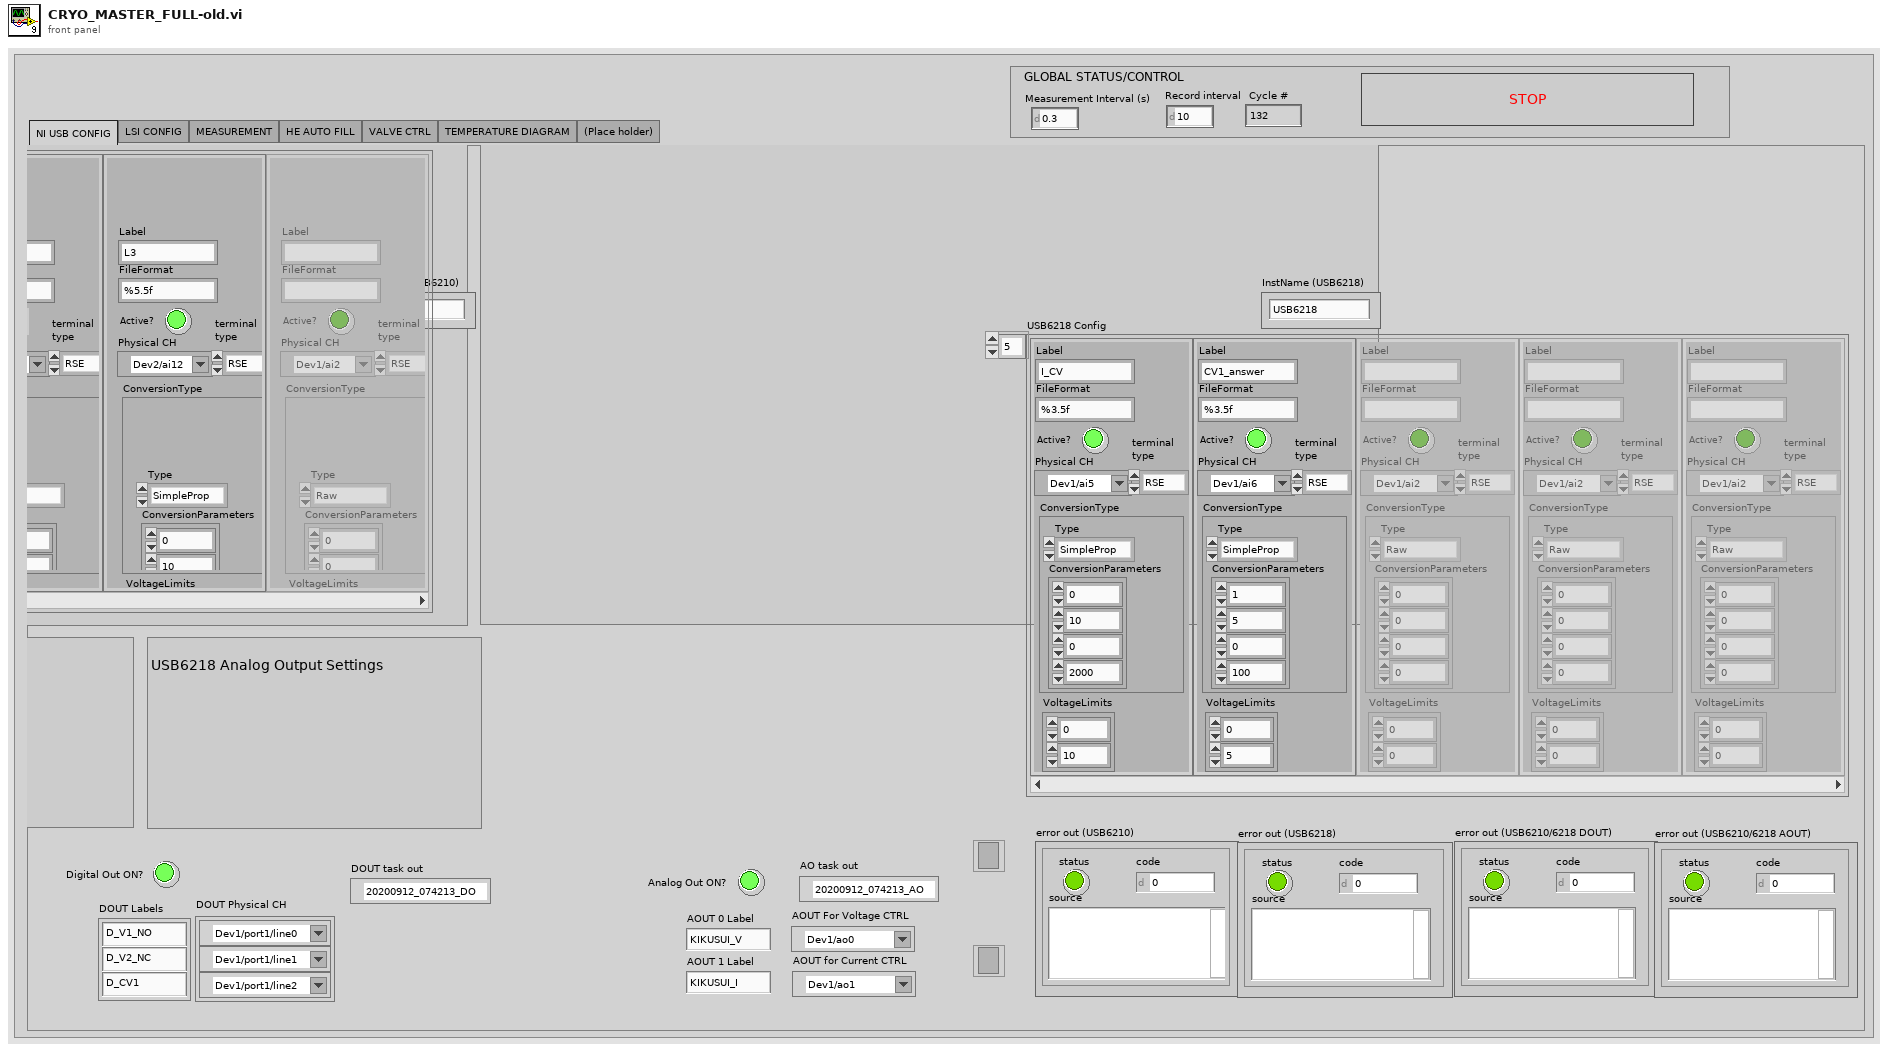
[diagram p1: front panel]
types:
  T1 = enum32{"NI USB CONFIG", "LSI CONFIG", "MEASUREMENT", "HE AUTO FILL", "VALVE CTRL", "TEMPERATURE DIAGRAM", "(Place holder)"}
  T2 = cluster{"Label":string, "FileFormat":string, "Active?":bool, "Physical CH":tag, " terminal\n type":i32, "ConversionType":cluster{"Type":enum16{"Raw", "SimpleProp", "CC-10_COMBINED", "CC-10_LOG", "LeakDet_EXP", "LeakDet_Mantissa", "Baratron"}, "ConversionParameters":dbl[]}, "VoltageLimits":dbl[]}[]
  T3 = cluster{"LSIName":string, "Labels":string[], "SensorLocations":enum16{"N.C.", "T3He1-1", "T3He1-2", "T3He1-3", "T3He1-4", "T3He2-1", "T3He2-2", "T3He3", "T3He4", "T3He5", "T3He6-1", "T3He6-2", "T3He7-1", "T3He7-2", "T3He8", "T3He9", "T3He10", "T4He1", "T4He2-1", "T4He2-2", "T4He3-1", "T4He3-2", "T4He3-3", "T4He3-4", "T4He4", "T4He5", "T4He6", "T4He7", "T4He8", "T4He9", "T4He10", "T1K1", "T1K2", "T1K3-1", "T1K3-2", "T1K4", "T1K5", "T1K6", "TIP1", "TIP2", "TIP3", "TIP4", "TIP5", "TIP6", "TIP7", "TTH1", "TTH2", "TTH3", "TTH4"}[], "Active?":bool, "VISA res. name":refnum<visa-resource-name>}[]
  T4 = cluster{"TimeArray":timestamp[], "DataArray":dbl[]}[]
  T5 = enum32{"USB6210", "USB6218", "Temeprature (1)", "Temperature (2)", "Temperature (3)"}
  T6 = enum16{"Intialized", "Ready", "Measuring", "Terminated"}
  T7 = enum16{"Initialized", "Ready", "Measuring", "Terminated"}
  T8 = cluster{"TimeArray":timestamp[], "Filtered X":dbl[]}[]
  T9 = cluster{"TimeArray (USB6218)":timestamp[], "DataArrayConv (USB6218)":dbl[]}[]
  T10 = cluster{"LSIName":string, "Active?":bool, "LastData":dbl[], "Labels":string[]}[]
  T11 = cluster{"appended array":timestamp[], "ActualCurrentArray":dbl[]}
  T12 = cluster{"appended array":timestamp[], "SetCurrentArray":dbl[]}
  T13 = cluster{"appended array":timestamp[], "SetCurrentArray":dbl[]}[]
  T14 = cluster{"TimeArray (USB6218)":timestamp[], "DataArrayConv (USB6218)":dbl[]}
  T15 = enum16{"open", "replace", "create", "open or create", "replace or create", "replace or create with confirmation"}
  T16 = cluster{"TimeArray":timestamp[], "DataArrayConv":dbl[]}[]
  T17 = cluster{"IndexArray":i64[], "TimeArray":timestamp[], "DataArrayRaw":dbl[][], "DataArrayConv":dbl[][], "LDArray":dbl[]}
  T18 = cluster{"InstName":string, "Active?":bool, "Status":enum16{"Intialized", "Ready", "Measuring", "Terminated"}, "Labels":string[], "LabelLD":string, "FileFormat":string[], "FileFormatLD":string, "ReadLeakDet?":bool}
  T19 = cluster{"TimeArray":timestamp[], "DataArrayConv":dbl[]}
  T20 = cluster{"TimeArray":timestamp[], "M.A. Array":dbl[]}
  T21 = cluster{"TimeArray":timestamp[], "M.A. Array":dbl[]}[]
  T22 = cluster{"TimeArray":timestamp[], "DataArray":dbl[]}
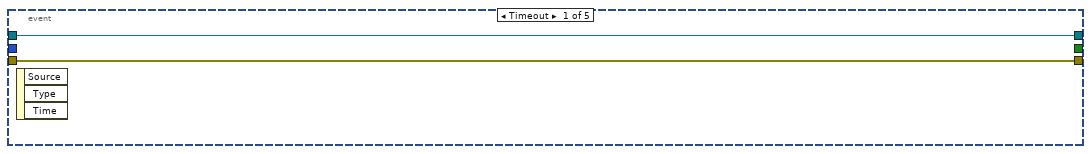
[diagram p3: hidden frame]
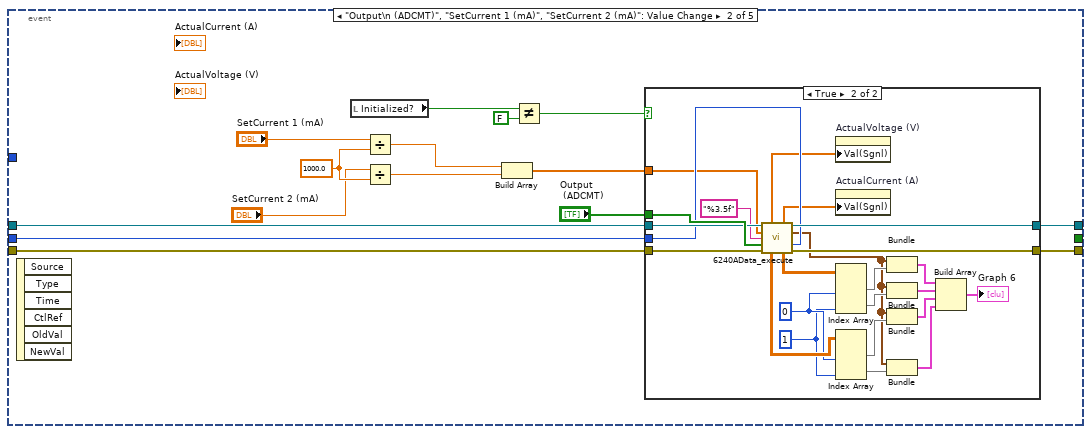
[diagram p4: hidden frame]
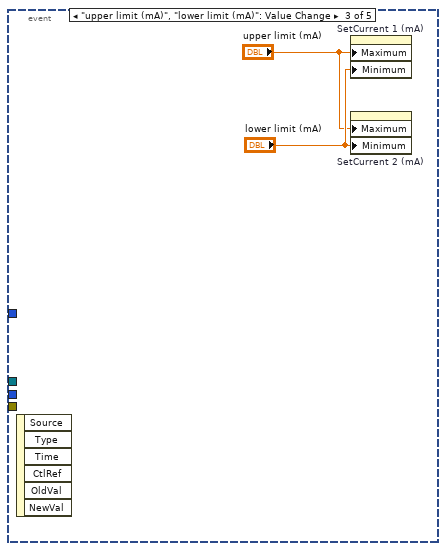
[diagram p6: hidden frame]
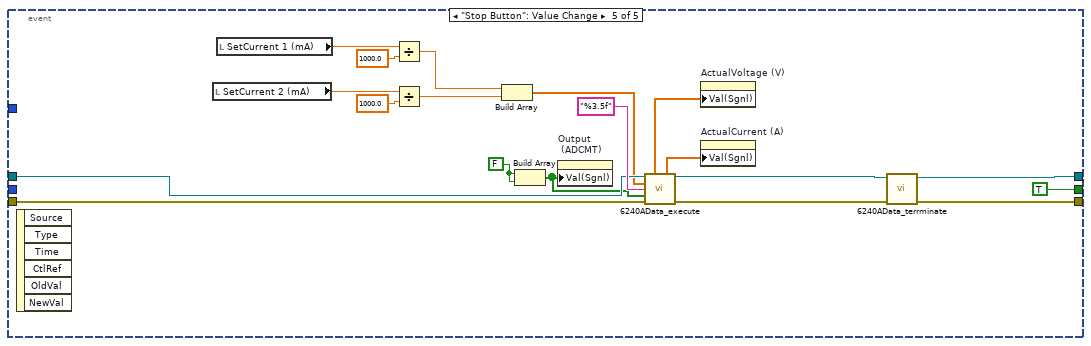
[diagram p8: hidden frame]
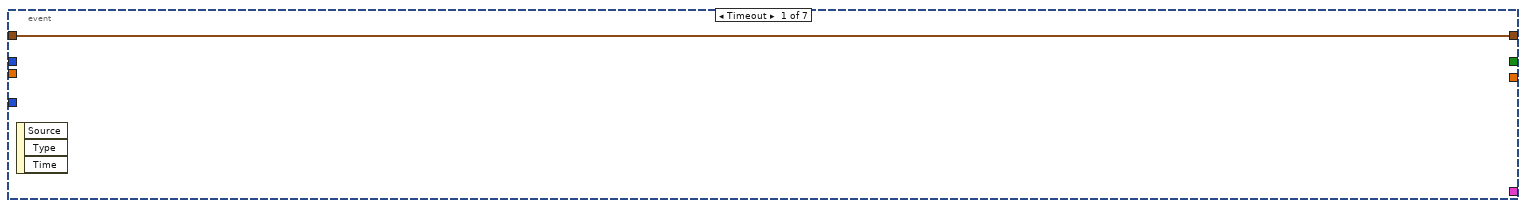
[diagram p9: hidden frame]
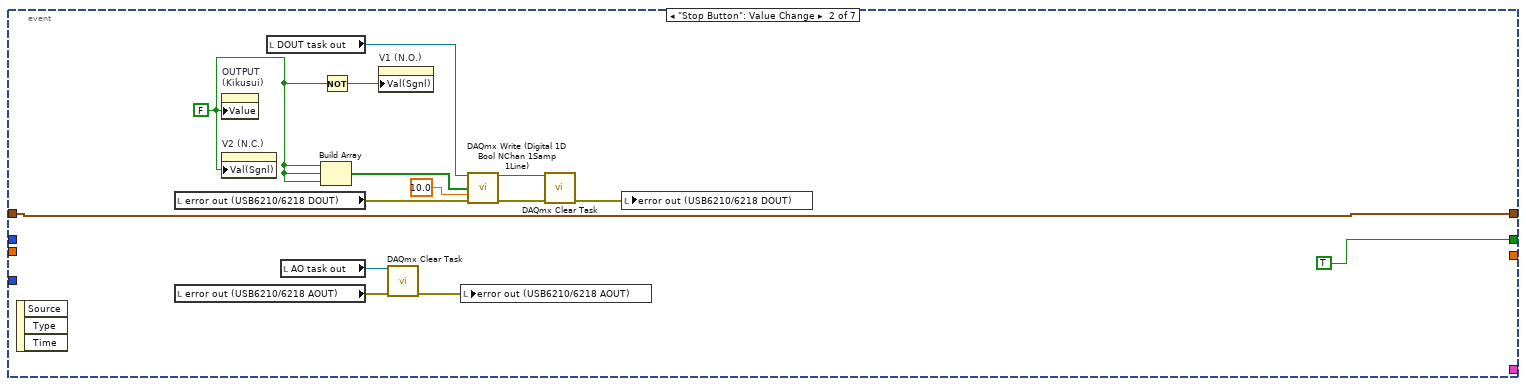
[diagram p10: hidden frame]
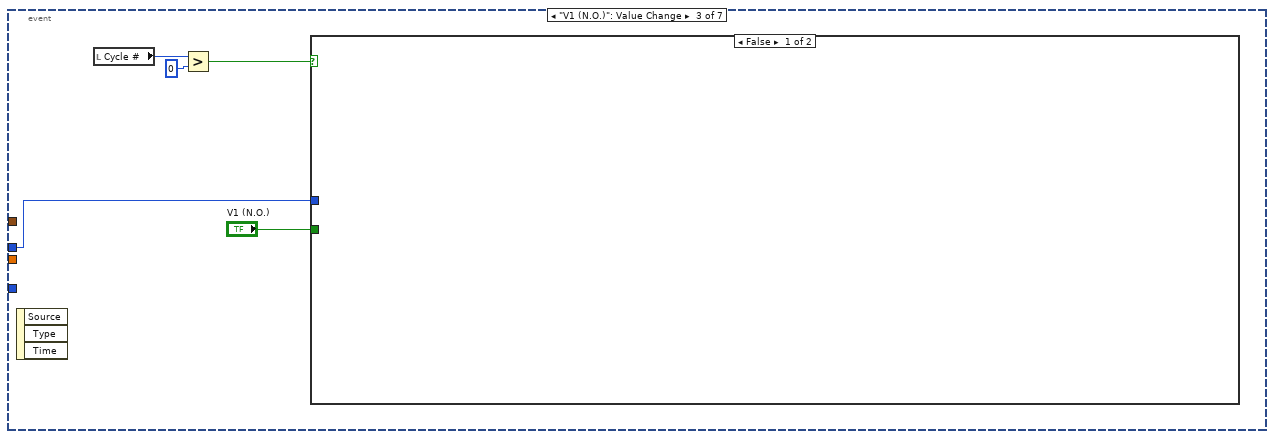
[diagram p11: hidden frame]
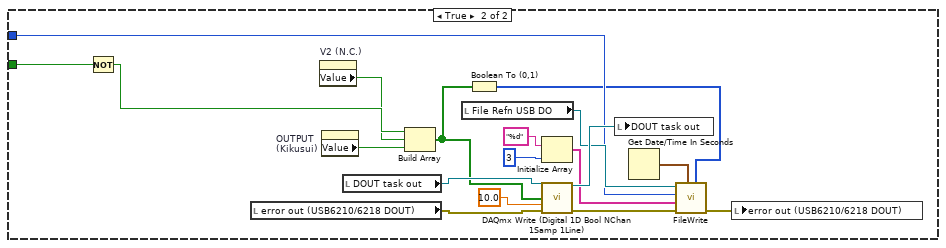
[diagram p12: hidden frame]
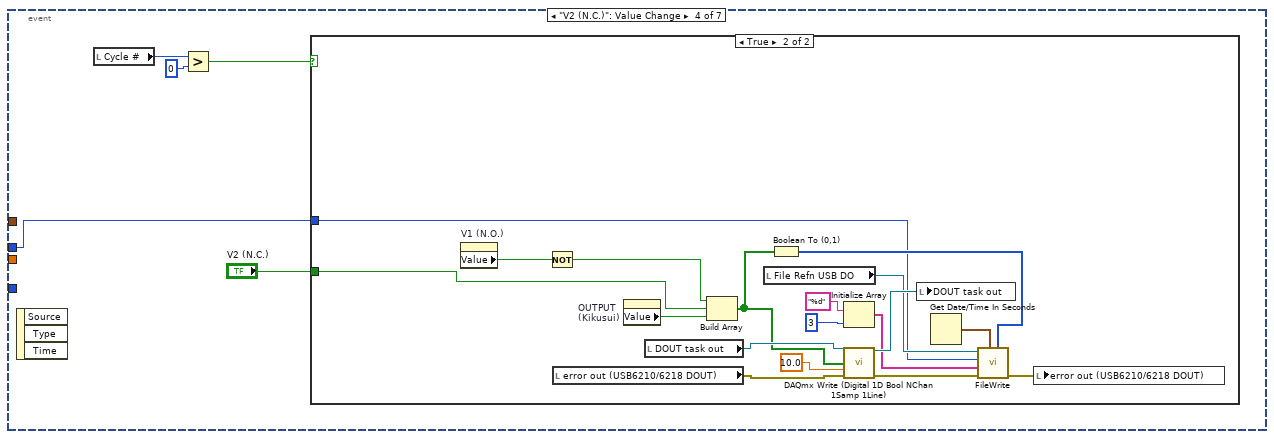
[diagram p13: hidden frame]
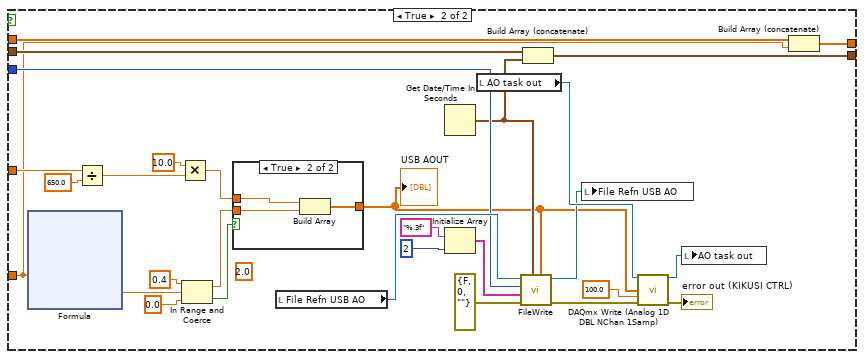
[diagram p15: hidden frame]
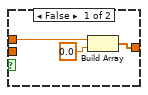
[diagram p16: hidden frame]
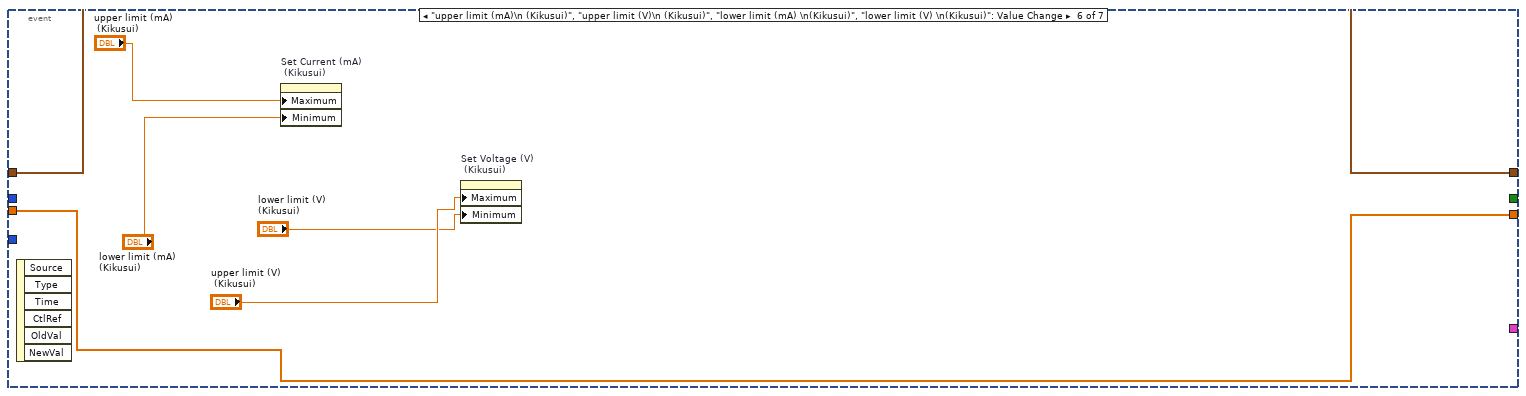
[diagram p17: hidden frame]
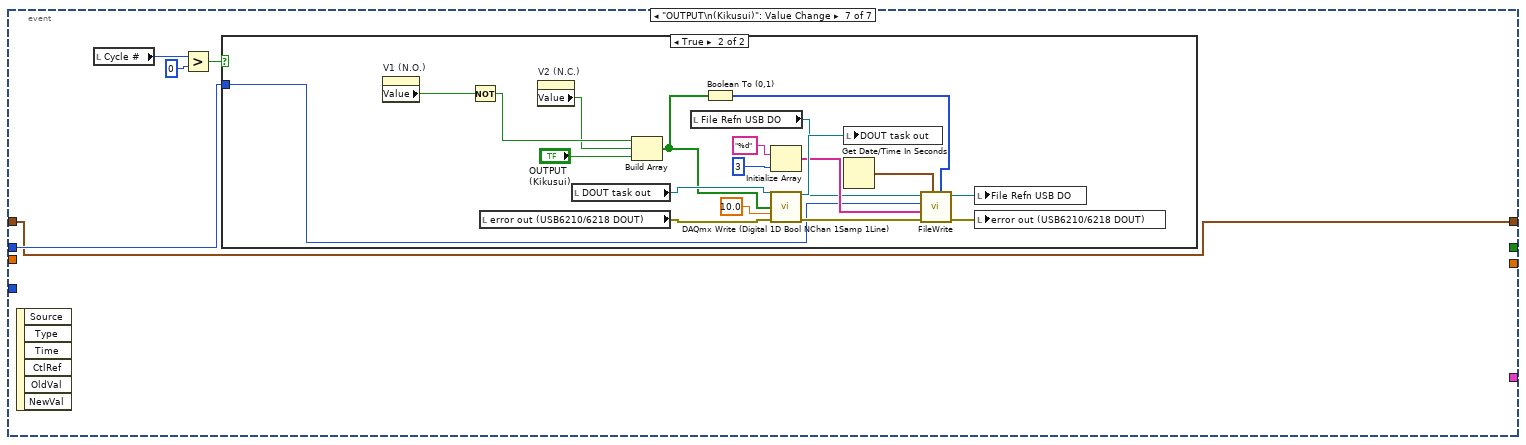
[diagram p18: hidden frame]
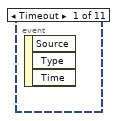
[diagram p20: hidden frame]
diagram:
  w3 = errorcluster {"status"=FALSE, "code"=0, "source"=""} ("error in (no error)")
  n1 = while {
    stop <- w31 stop-if-true
    n2 = event shown="[6] \"Take Screenshot! 1\": Value Change" {
      selector: _ -> [_ _ _ _ _ _ _ _ _ _ _]
      dyn-events: _ -> [_ _ _ _ _ _ _ _ _ _ _]
      timeout: _ -> [_ _ _ _ _ _ _ _ _ _ _]
      tunnel: [_ _ _ _ _ _ _ _ _ _ TRUE] -> w31
      event Timeout {
        n3 = event-data() -> ()  [unwired: 1 in, 3 out]
      }
      event "log/linear 1": Value Change {
        n4 = event-data() -> ()  [unwired: 1 in, 6 out]
        n5 = flat-sequence {
          frame #0 {
            n6 = control-ref of="Graph 1"() -> (w34:refnum<vi>)
            n7 = Boolean To (0,1)(Boolean="log/linear 1") -> (0, 1=w38:i16)
            n8 = property class="XYGraph (strict)"(reference=w34, error in=errorcluster {"status"=FALSE, "code"=0, "source"=""} ("error in (no error)"), "YScale.Mapping Mode"=w38) -> (error out=w36:errorcluster)  [unwired: 1 out]
            n9 = control-ref of="error out (USB6210)"() -> (w37:refnum<vi>)
            n10 = property class="Clust (strict)"(reference=w37, "Val(Sgnl)"=w36) -> ()  [unwired: 1 in, 2 out]
          }
        }
      }
      event "log/linear 2": Value Change {
        n11 = event-data() -> ()  [unwired: 1 in, 6 out]
        n12 = flat-sequence {
          frame #0 {
            n13 = control-ref of="Graph 2"() -> (w42:refnum<vi>)
            n14 = Boolean To (0,1)(Boolean="log/linear 2") -> (0, 1=w44:i16)
            n15 = property class="XYGraph (strict)"(reference=w42, error in=errorcluster {"status"=FALSE, "code"=0, "source"=""} ("error in (no error)"), "YScale.Mapping Mode"=w44) -> (error out=w43:errorcluster)  [unwired: 1 out]
            n16 = control-ref of="error out (USB6210)"() -> (w41:refnum<vi>)
            n17 = property class="Clust (strict)"(reference=w41, "Value"=w43) -> ()  [unwired: 1 in, 2 out]
          }
        }
      }
      event "log/linear 3": Value Change {
        n18 = event-data() -> ()  [unwired: 1 in, 6 out]
        n19 = flat-sequence {
          frame #0 {
            n20 = control-ref of="Graph 3"() -> (w46:refnum<vi>)
            n21 = Boolean To (0,1)(Boolean="log/linear 3") -> (0, 1=w50:i16)
            n22 = property class="XYGraph (strict)"(reference=w46, error in=errorcluster {"status"=FALSE, "code"=0, "source"=""} ("error in (no error)"), "YScale.Mapping Mode"=w50) -> (error out=w49:errorcluster)  [unwired: 1 out]
            n23 = control-ref of="error out (USB6210)"() -> (w48:refnum<vi>)
            n24 = property class="Clust (strict)"(reference=w48, "Value"=w49) -> ()  [unwired: 1 in, 2 out]
          }
        }
      }
      event "log/linear 4": Value Change {
        n25 = event-data() -> ()  [unwired: 1 in, 6 out]
        n26 = flat-sequence {
          frame #0 {
            n27 = control-ref of="Graph 4"() -> (w52:refnum<vi>)
            n28 = Boolean To (0,1)(Boolean="log/linear 4") -> (0, 1=w56:i16)
            n29 = property class="XYGraph (strict)"(reference=w52, error in=errorcluster {"status"=FALSE, "code"=0, "source"=""} ("error in (no error)"), "YScale.Mapping Mode"=w56) -> (error out=w55:errorcluster)  [unwired: 1 out]
            n30 = control-ref of="error out (USB6210)"() -> (w54:refnum<vi>)
            n31 = property class="Clust (strict)"(reference=w54, "Value"=w55) -> ()  [unwired: 1 in, 2 out]
          }
        }
      }
      event "Plot selecter LSI218(1)\n    1      2     3     4", "Plot selecter LSI218(2)\n    1      2     3     4", "Plot selecter (USB6210)\n    1      2     3     4", "Plot selecter LSI336 \n     1      2     3     4", "Plot selecter (USB6218)\n    1      2     3     4": Value Change {
        n32 = event-data() -> ()  [unwired: 1 in, 6 out]
        n33 = local read "All Labels (USB6210)"() -> (w74:string[])
        n34 = local read "All Labels (USB6218)"() -> (w63:string[])
        n35 = local read "Labels LSI218 (1)"() -> (w76:string[])
        n36 = local read "Labels LSI218 (2)"() -> (w77:string[])
        n37 = local read "Labels LSI336"() -> (w69:string[])
        n38 = call "BuildPlotLegends.vi"("Plot selecter \n    1      2     3     4"="Plot selecter (USB6210)\n    1      2     3     4", "AllLabels"=w74) -> ("Series 4"=w86:string[], "Series 3"=w84:string[], "Series 2"=w82:string[], "Series 1"=w80:string[])  [unwired: 6 in]
        n39 = call "BuildPlotLegends_LSI218.vi"("Plot selecter (2)\n    1      2     3     5"="Plot selecter LSI218(2)\n    1      2     3     4", "Plot selecter (1)\n    1      2     3     4"="Plot selecter LSI218(1)\n    1      2     3     4", "Labels (2)"=w77, "Labels (1)"=w76) -> ("Series 4"=w87:string[], "Series 3"=w85:string[], "Series 2"=w83:string[], "Series 1"=w81:string[])  [unwired: 4 in]
        n40 = call "BuildPlotLegends.vi"("Plot selecter \n    1      2     3     4"="Plot selecter LSI336 \n     1      2     3     4", "AllLabels"=w69) -> ("Series 4"=w64:string[], "Series 3"=w65:string[], "Series 2"=w66:string[], "Series 1"=w67:string[])  [unwired: 6 in]
        n41 = call "BuildPlotLegends.vi"("Plot selecter \n    1      2     3     4"="Plot selecter (USB6218)\n    1      2     3     4", "AllLabels"=w63) -> ("Series 4"=w59:string[], "Series 3"=w58:string[], "Series 2"=w60:string[], "Series 1"=w61:string[])  [unwired: 6 in]
        n42 = Build Array (concatenate)(w82, w83, w66, w60) -> (w71:string[])
        "Series 2" <- w71
        n43 = Build Array (concatenate)(w84, w85, w65, w58) -> (w72:string[])
        "Series 3" <- w72
        n44 = Build Array (concatenate)(w86, w87, w64, w59) -> (w73:string[])
        "Series 4" <- w73
        n45 = Build Array (concatenate)(w80, w81, w67, w61) -> (w70:string[])
        "Series 1" <- w70
        n46 = stacked-sequence {
          tunnel: [w97 _ _ _] -> w91
          tunnel: [_ w115 _ _] -> w92
          tunnel: [_ _ w132 _] -> w90
          tunnel: [_ _ _ w148] -> w89
          tunnel: w70 -> [w94 _ _ _]
          tunnel: w71 -> [_ w111 _ _]
          tunnel: w72 -> [_ _ w129 _]
          tunnel: w73 -> [_ _ _ w145]
          frame #0 {
            n47 = Array Size(array=w94) -> (size(s)=w99:i32)
            n48 = control-ref of="Graph 1"() -> (w93:refnum<vi>)
            n49 = for {
              N: 18 -> [_]
              tunnel: w93 -> [w108]
              shift-right: [w106] -> w98
              shift-left: errorcluster {"status"=FALSE, "code"=0, "source"=""} ("error in (no error)") -> [w107]
              i -> [w110]
              n50 = property class="XYGraph (strict)"(reference=w108, error in=w107, "Active Plot"=w110, "Plot.Plot Name"="") -> (error out=w106:errorcluster)  [unwired: 1 out]
            }
            n51 = for {
              N: w99 -> [_]
              tunnel: w93 -> [w104]
              shift-right: [w102] -> w97
              shift-left: w98 -> [w103]
              tunnel: w94 -> [w101] mode=indexing
              i -> [w105]
              n52 = property class="XYGraph (strict)"(reference=w104, error in=w103, "Active Plot"=w105, "Plot.Plot Name"=w101, "Plot.Visible?"=TRUE ("Plot.Visible")) -> (error out=w102:errorcluster)  [unwired: 1 out]
            }
          }
          frame #1 {
            n53 = Array Size(array=w111) -> (size(s)=w117:i32)
            n54 = control-ref of="Graph 2"() -> (w114:refnum<vi>)
            n55 = for {
              N: 18 -> [_]
              shift-right: [w124] -> w116
              shift-left: errorcluster {"status"=FALSE, "code"=0, "source"=""} ("error in (no error)") -> [w125]
              tunnel: w114 -> [w123]
              i -> [w127]
              n56 = property class="XYGraph (strict)"(reference=w123, error in=w125, "Active Plot"=w127, "Plot.Plot Name"="") -> (error out=w124:errorcluster)  [unwired: 1 out]
            }
            n57 = for {
              N: w117 -> [_]
              shift-right: [w120] -> w115
              shift-left: w116 -> [w121]
              tunnel: w111 -> [w119] mode=indexing
              tunnel: w114 -> [w118]
              i -> [w122]
              n58 = property class="XYGraph (strict)"(reference=w118, error in=w121, "Active Plot"=w122, "Plot.Plot Name"=w119) -> (error out=w120:errorcluster)  [unwired: 1 out]
            }
          }
          frame #2 {
            n59 = Array Size(array=w129) -> (size(s)=w134:i32)
            n60 = control-ref of="Graph 3"() -> (w128:refnum<vi>)
            n61 = for {
              N: 18 -> [_]
              tunnel: w128 -> [w142]
              shift-right: [w140] -> w133
              shift-left: errorcluster {"status"=FALSE, "code"=0, "source"=""} ("error in (no error)") -> [w141]
              i -> [w144]
              n62 = property class="XYGraph (strict)"(reference=w142, error in=w141, "Active Plot"=w144, "Plot.Plot Name"="") -> (error out=w140:errorcluster)  [unwired: 1 out]
            }
            n63 = for {
              N: w134 -> [_]
              tunnel: w128 -> [w138]
              shift-right: [w136] -> w132
              shift-left: w133 -> [w137]
              tunnel: w129 -> [w135] mode=indexing
              i -> [w139]
              n64 = property class="XYGraph (strict)"(reference=w138, error in=w137, "Active Plot"=w139, "Plot.Plot Name"=w135) -> (error out=w136:errorcluster)  [unwired: 1 out]
            }
          }
          frame #3 {
            n65 = Array Size(array=w145) -> (size(s)=w151:i32)
            n66 = control-ref of="Graph 4"() -> (w149:refnum<vi>)
            n67 = for {
              N: 18 -> [_]
              tunnel: w149 -> [w159]
              shift-right: [w157] -> w150
              shift-left: errorcluster {"status"=FALSE, "code"=0, "source"=""} ("error in (no error)") -> [w158]
              i -> [w161]
              n68 = property class="XYGraph (strict)"(reference=w159, error in=w158, "Active Plot"=w161, "Plot.Plot Name"="") -> (error out=w157:errorcluster)  [unwired: 1 out]
            }
            n69 = for {
              N: w151 -> [_]
              tunnel: w149 -> [w155]
              shift-right: [w153] -> w148
              shift-left: w150 -> [w154]
              tunnel: w145 -> [w152] mode=indexing
              i -> [w156]
              n70 = property class="XYGraph (strict)"(reference=w155, error in=w154, "Active Plot"=w156, "Plot.Plot Name"=w152) -> (error out=w153:errorcluster)  [unwired: 1 out]
            }
          }
        }
        n71 = Merge Errors(w91, w92, w90, w89) -> (→"Plot errors":errorcluster)
      }
      event "Take Screenshot! 1": Value Change {
        n72 = event-data() -> ()  [unwired: 1 in, 6 out]
        n73 = flat-sequence {
          frame #0 {
            n74 = flat-sequence {
              frame #0 {
                w166 = "_" ("string")
                n75 = Get Date/Time In Seconds() -> (seconds since 1Jan1904=w163:timestamp)
                n76 = local read "RUN identifier"() -> (w169:string)
                n77 = call "LV_UNIXTIME.vi"("current time"=w163) -> ("date/time string"=w167:string)  [unwired: 9 in, 1 out]
                n78 = local read "Base Path"() -> (w170:path)
                n79 = Concatenate Strings(w169, w166, w167, w166, "FIle suffix 1", ".bmp" ("string")) -> (w175:string)
                n80 = control-ref of="Graph 1"() -> (w162:refnum<vi>)
                n81 = Build Path(base path=w170, name or relative path=w175) -> (appended path=w174:path)
                n82 = invoke on="Invoke Node" class="XYGraph (strict)" method="Export Image"(reference=w162, "FileType"=enum32{"BMP", "EPS", "EMF", "PICT"}."BMP" ("File Type"), "Target"=enum32{"File", "Clipboard"}."File", "Path"=w174, "HideGrid"=FALSE ("Hide Grid"), "Overwrite"=TRUE ("Always Overwrite")) -> ()  [unwired: 2 in, 8 out]
              }
              frame #1 {
                n83 = local write "Take Screenshot! 1"(FALSE ("Take Screenshot! 1")) -> ()
              }
            }
          }
        }
      }
      event "Take Screenshot! 2": Value Change {
        n84 = event-data() -> ()  [unwired: 1 in, 6 out]
        n85 = flat-sequence {
          frame #0 {
            n86 = flat-sequence {
              frame #0 {
                w181 = "_" ("string")
                n87 = Get Date/Time In Seconds() -> (seconds since 1Jan1904=w177:timestamp)
                n88 = local read "RUN identifier"() -> (w184:string)
                n89 = call "LV_UNIXTIME.vi"("current time"=w177) -> ("date/time string"=w182:string)  [unwired: 9 in, 1 out]
                n90 = local read "Base Path"() -> (w185:path)
                n91 = Concatenate Strings(w184, w181, w182, w181, "FIle suffix 2", ".bmp" ("string")) -> (w190:string)
                n92 = control-ref of="Graph 2"() -> (w178:refnum<vi>)
                n93 = Build Path(base path=w185, name or relative path=w190) -> (appended path=w189:path)
                n94 = invoke on="Invoke Node" class="XYGraph (strict)" method="Export Image"(reference=w178, "FileType"=enum32{"BMP", "EPS", "EMF", "PICT"}."BMP" ("File Type"), "Target"=enum32{"File", "Clipboard"}."File", "Path"=w189, "HideGrid"=FALSE ("Hide Grid"), "Overwrite"=TRUE ("Always Overwrite")) -> ()  [unwired: 2 in, 8 out]
              }
              frame #1 {
                n95 = local write "Take Screenshot! 2"(FALSE ("Take Screenshot! 1")) -> ()
              }
            }
          }
        }
      }
      event "Take Screenshot! 3": Value Change {
        n96 = event-data() -> ()  [unwired: 1 in, 6 out]
        n97 = flat-sequence {
          frame #0 {
            n98 = flat-sequence {
              frame #0 {
                w196 = "_" ("string")
                n99 = Get Date/Time In Seconds() -> (seconds since 1Jan1904=w194:timestamp)
                n100 = local read "RUN identifier"() -> (w199:string)
                n101 = call "LV_UNIXTIME.vi"("current time"=w194) -> ("date/time string"=w197:string)  [unwired: 9 in, 1 out]
                n102 = local read "Base Path"() -> (w200:path)
                n103 = Concatenate Strings(w199, w196, w197, w196, "FIle suffix 3", ".bmp" ("string")) -> (w205:string)
                n104 = control-ref of="Graph 3"() -> (w192:refnum<vi>)
                n105 = Build Path(base path=w200, name or relative path=w205) -> (appended path=w204:path)
                n106 = invoke on="Invoke Node" class="XYGraph (strict)" method="Export Image"(reference=w192, "FileType"=enum32{"BMP", "EPS", "EMF", "PICT"}."BMP" ("File Type"), "Target"=enum32{"File", "Clipboard"}."File", "Path"=w204, "HideGrid"=FALSE ("Hide Grid"), "Overwrite"=TRUE ("Always Overwrite")) -> ()  [unwired: 2 in, 8 out]
              }
              frame #1 {
                n107 = local write "Take Screenshot! 3"(FALSE ("Take Screenshot! 1")) -> ()
              }
            }
          }
        }
      }
      event "Take Screenshot! 4": Value Change {
        n108 = event-data() -> ()  [unwired: 1 in, 6 out]
        n109 = flat-sequence {
          frame #0 {
            n110 = flat-sequence {
              frame #0 {
                w211 = "_" ("string")
                n111 = Get Date/Time In Seconds() -> (seconds since 1Jan1904=w209:timestamp)
                n112 = local read "RUN identifier"() -> (w214:string)
                n113 = call "LV_UNIXTIME.vi"("current time"=w209) -> ("date/time string"=w212:string)  [unwired: 9 in, 1 out]
                n114 = local read "Base Path"() -> (w215:path)
                n115 = Concatenate Strings(w214, w211, w212, w211, "FIle suffix 4", ".bmp" ("string")) -> (w220:string)
                n116 = control-ref of="Graph 4"() -> (w207:refnum<vi>)
                n117 = Build Path(base path=w215, name or relative path=w220) -> (appended path=w219:path)
                n118 = invoke on="Invoke Node" class="XYGraph (strict)" method="Export Image"(reference=w207, "FileType"=enum32{"BMP", "EPS", "EMF", "PICT"}."BMP" ("File Type"), "Target"=enum32{"File", "Clipboard"}."File", "Path"=w219, "HideGrid"=FALSE ("Hide Grid"), "Overwrite"=TRUE ("Always Overwrite")) -> ()  [unwired: 2 in, 8 out]
              }
              frame #1 {
                n119 = local write "Take Screenshot! 4"(FALSE ("Take Screenshot! 1")) -> ()
              }
            }
          }
        }
      }
      event "Stop Button": Value Change {
        n120 = event-data() -> ()  [unwired: 1 in, 6 out]
      }
    }
    n121 = local write "Take Screenshot! 4"(FALSE ("Take Screenshot! 1")) -> ()
    n122 = local write "Take Screenshot! 1"(FALSE ("Take Screenshot! 1")) -> ()
    n123 = local write "Take Screenshot! 2"(FALSE ("Take Screenshot! 1")) -> ()
    n124 = local write "Take Screenshot! 3"(FALSE ("Take Screenshot! 1")) -> ()
    n125 = Wait (ms)(milliseconds to wait=u32 1000) -> ()  [unwired: 1 out]
  }
  n126 = while {
    shift-right: [w231] -> _
    shift-left: refnum<class "6240AData.lvclass"> refnum ("6240AData.lvclass") -> [w229]
    shift-right: [w227] -> _
    shift-left: errorcluster {"status"=FALSE, "code"=0, "source"=""} ("error in (no error)") -> [w228]
    i -> [w223]
    stop <- w230 stop-if-true
    n127 = Wait (ms)(milliseconds to wait=u32 231) -> ()  [unwired: 1 out]
    n128 = Equal?(x=w223, y=0) -> (x = y?=w225:bool)
    n129 = case shown="True" w225 {
      frame False {
      }
      frame True {
        n130 = property on="Initialized?" class="Bool (strict)"("Val(Sgnl)"=FALSE ("Value (Signaling)")) -> ()  [unwired: 2 in, 2 out]
      }
    }
    n131 = event shown="[3] \"Initialize\": Value Change" {
      selector: _ -> [_ _ _ _ _]
      dyn-events: _ -> [_ _ _ _ _]
      timeout: _ -> [_ _ _ _ _]
      tunnel: [w234 w249 _ w298 w331] -> w231
      tunnel: [_ _ _ _ TRUE ("Value (Signaling)")] -> w230
      tunnel: w229 -> [w234 w248 _ w282 w325]
      tunnel: w228 -> [w233 w247 _ w281 w323]
      tunnel: [w233 w246 _ w296 w330] -> w227
      tunnel: w223 -> [_ w245 _ _ _]
      tunnel: w223 -> [_ _ _ w290 _]
      event Timeout {
        n132 = event-data() -> ()  [unwired: 1 in, 3 out]
      }
      event "Output\n (ADCMT)", "SetCurrent 1 (mA)", "SetCurrent 2 (mA)": Value Change {
        w238 = 1000.0 ("y")
        n133 = event-data() -> ()  [unwired: 1 in, 6 out]
        n134 = local read "Initialized?"() -> (w244:bool)
        n135 = Divide(x="SetCurrent 1 (mA)", y=w238) -> (x/y=w239:dbl)
        n136 = Divide(x="SetCurrent 2 (mA)", y=w238) -> (x/y=w240:dbl)
        n137 = Build Array(w239, w240) -> (w237:dbl[])
        n138 = Not Equal?(x=w244, y=FALSE) -> (x != y?=w242:bool)
        n139 = case shown="True" w242 {
          tunnel: [w251 w275] -> w249
          tunnel: "Output\n (ADCMT)" -> [_ w274]
          tunnel: w248 -> [w251 w273]
          tunnel: w247 -> [w250 w272]
          tunnel: [w250 w271] -> w246
          tunnel: w245 -> [_ w267]
          tunnel: w237 -> [_ w253]
          frame False {
          }
          frame True {
            w260 = 1 ("index (col)")
            w261 = 0 ("disabled index (col)")
            n140 = call-dynamic "6240AData_execute.vi"("6240AData in"=w273, "SetCurrent (A)"=w253, "FileFormat"="%3.5f", "Output status"=w274, "ExecutionIndex"=w267, "error in (no error)"=w272) -> ("ActualVoltage (V)"=w252:dbl[], "ActualCurrent (A)"=w266:dbl[], "6240AData out"=w275:refnum<class "6240AData.lvclass">, "appended array"=w256:timestamp[], "SetCurrentArray"=w262:dbl[][], "ActualCurrentArray"=w269:dbl[][], "error out"=w271:errorcluster)  [unwired: 3 in]
            n141 = property on="ActualVoltage (V)" class="Arr (strict)"("Val(Sgnl)"=w252) -> ()  [unwired: 2 in, 2 out]
            n142 = property on="ActualCurrent (A)" class="Arr (strict)"("Val(Sgnl)"=w266) -> ()  [unwired: 2 in, 2 out]
            n143 = Index Array(array=w269, index (col) #1=w261, index (col) #2=w260) -> (element #1=w270:dbl[], element #2=w264:dbl[])  [unwired: 2 in]
            n144 = Index Array(array=w262, index (col) #1=w261, index (col) #2=w260) -> (element #1=w258:dbl[], element #2=w255:dbl[])  [unwired: 2 in]
            n145 = Bundle("appended array"=w256, "ActualCurrentArray"=w270) -> (w265:T11)  [unwired: 1 in]
            n146 = Bundle("appended array"=w256, "ActualCurrentArray"=w264) -> (w259:T11)  [unwired: 1 in]
            n147 = Bundle("appended array"=w256, "SetCurrentArray"=w258) -> (w257:T12)  [unwired: 1 in]
            n148 = Bundle("appended array"=w256, "SetCurrentArray"=w255) -> (w254:T12)  [unwired: 1 in]
            n149 = Build Array(w265, w259, w257, w254) -> (→"Graph 6":T13)
          }
        }
      }
      event "upper limit (mA)", "lower limit (mA)": Value Change {
        n150 = event-data() -> ()  [unwired: 1 in, 6 out]
        n151 = property on="SetCurrent 1 (mA)" class="DigNum (strict)"("Maximum"="upper limit (mA)", "Minimum"="lower limit (mA)") -> ()  [unwired: 2 in, 2 out]
        n152 = property on="SetCurrent 2 (mA)" class="DigNum (strict)"("Maximum"="upper limit (mA)", "Minimum"="lower limit (mA)") -> ()  [unwired: 2 in, 2 out]
      }
      event "Initialize": Value Change {
        w292 = FALSE
        n153 = event-data() -> ()  [unwired: 1 in, 6 out]
        n154 = local read "Initialized?"() -> (w280:bool)
        n155 = case shown="True" w280 {
          tunnel: w282 -> [w309 w313]
          tunnel: w281 -> [w308 w312]
          tunnel: [w309 w311] -> w279
          tunnel: [w308 w310] -> w278
          frame False {
          }
          frame True {
            n156 = call-dynamic "6240AData_terrminate.vi"("error in (no error)"=w312, "6240AData in"=w313) -> ("error out"=w310:errorcluster, "6240AData out"=w311:refnum<class "6240AData.lvclass">)  [unwired: 8 in]
          }
        }
        n157 = property on="Initialized?" class="Bool (strict)"("Val(Sgnl)"=TRUE ("Value (Signaling)")) -> ()  [unwired: 2 in, 2 out]
        n158 = local read "SetCurrent 1 (mA)"() -> (w288:dbl)
        n159 = local read "SetCurrent 2 (mA)"() -> (w285:dbl)
        n160 = local read "RUN identifier"() -> (w300:string)
        n161 = local read "Base Path"() -> (w301:path)
        n162 = Divide(x=w288, y=1000.0) -> (x/y=w287:dbl)
        n163 = Divide(x=w285, y=1000.0) -> (x/y=w284:dbl)
        n164 = Get Date/Time In Seconds() -> (seconds since 1Jan1904=w307:timestamp)
        n165 = call-dynamic "6240AData_initialize.vi"("6240AData in"=w279, "RunName"=w300, "InstName"="InstName", "start time"=w307, "base path"=w301, "VISA"="VISA", "error in (no error)"=w278, "CtrlLabels"="CtrlLabels", "Voltage limits (V)"="Voltage limits (V)") -> ("6240AData out"=w299:refnum<class "6240AData.lvclass">, "error out"=w297:errorcluster)  [unwired: 5 in]
        n166 = Build Array(w287, w284) -> (w283:dbl[])
        n167 = Build Array(w292, w292) -> (w291:bool[])
        n168 = call-dynamic "6240AData_execute.vi"("6240AData in"=w299, "SetCurrent (A)"=w283, "FileFormat"="%3.5f", "Output status"=w291, "ExecutionIndex"=w290, "error in (no error)"=w297) -> ("ActualVoltage (V)"=w294:dbl[], "ActualCurrent (A)"=w293:dbl[], "6240AData out"=w298:refnum<class "6240AData.lvclass">, "error out"=w296:errorcluster)  [unwired: 3 in, 3 out]
        n169 = property on="ActualVoltage (V)" class="Arr (strict)"("Val(Sgnl)"=w294) -> ()  [unwired: 2 in, 2 out]
        n170 = property on="ActualCurrent (A)" class="Arr (strict)"("Val(Sgnl)"=w293) -> ()  [unwired: 2 in, 2 out]
      }
      event "Stop Button": Value Change {
        w329 = FALSE
        n171 = event-data() -> ()  [unwired: 1 in, 6 out]
        n172 = local read "SetCurrent 2 (mA)"() -> (w315:dbl)
        n173 = local read "SetCurrent 1 (mA)"() -> (w319:dbl)
        n174 = Divide(x=w319, y=1000.0) -> (x/y=w317:dbl)
        n175 = Divide(x=w315, y=1000.0) -> (x/y=w314:dbl)
        n176 = Build Array(w317, w314) -> (w321:dbl[])
        n177 = Build Array(w329, w329) -> (w320:bool[])
        n178 = property on="Output\n (ADCMT)" class="Arr (strict)"("Val(Sgnl)"=w320) -> ()  [unwired: 2 in, 2 out]
        n179 = call-dynamic "6240AData_execute.vi"("6240AData in"=w325, "SetCurrent (A)"=w321, "FileFormat"="%3.5f", "Output status"=w320, "error in (no error)"=w323) -> ("ActualVoltage (V)"=w326:dbl[], "ActualCurrent (A)"=w327:dbl[], "6240AData out"=w324:refnum<class "6240AData.lvclass">, "error out"=w322:errorcluster)  [unwired: 4 in, 3 out]
        n180 = property on="ActualVoltage (V)" class="Arr (strict)"("Val(Sgnl)"=w326) -> ()  [unwired: 2 in, 2 out]
        n181 = property on="ActualCurrent (A)" class="Arr (strict)"("Val(Sgnl)"=w327) -> ()  [unwired: 2 in, 2 out]
        n182 = call-dynamic "6240AData_terrminate.vi"("error in (no error)"=w322, "6240AData in"=w324) -> ("error out"=w330:errorcluster, "6240AData out"=w331:refnum<class "6240AData.lvclass">)  [unwired: 8 in]
      }
    }
    "error out (ADCMT6420A)" <- w227
  }
  n183 = while {
    shift-right: [w334] -> _
    shift-left: dbl[] [] -> [w340]
    shift-right: [w337] -> _
    shift-left: timestamp[] [] -> [w339]
    i -> [w338]
    stop <- w341 stop-if-true
    n184 = Wait (ms)(milliseconds to wait=u32 225) -> ()  [unwired: 1 out]
    n185 = event shown="[4] \"update current\", \"Set Voltage (V)  (Kikusui)\", \"Set Current (mA)  (Kikusui)\": Value Change" {
      selector: _ -> [_ _ _ _ _ _ _]
      dyn-events: _ -> [_ _ _ _ _ _ _]
      timeout: _ -> [_ _ _ _ _ _ _]
      tunnel: [_ TRUE _ _ _ _ _] -> w341
      tunnel: w338 -> [_ _ _ _ w419 _ _]
      tunnel: [_ _ _ _ w418 w477 _] -> w334
      tunnel: w340 -> [_ _ _ _ w415 w477 _]
      tunnel: [w343 w353 _ _ w417 w476 w482] -> w337
      tunnel: w339 -> [w343 w353 _ _ w416 w476 w482]
      tunnel: w338 -> [_ _ w358 w381 _ _ w483]
      tunnel: [_ _ _ _ w404 _ _] -> w333
      event Timeout {
        n186 = event-data() -> ()  [unwired: 1 in, 3 out]
      }
      event "Stop Button": Value Change {
        w344 = FALSE
        n187 = event-data() -> ()  [unwired: 1 in, 3 out]
        n188 = local read "error out (USB6210/6218 DOUT)"() -> (w352:errorcluster)
        n189 = local read "error out (USB6210/6218 AOUT)"() -> (w349:errorcluster)
        n190 = property on="OUTPUT\n(Kikusui)" class="Bool (strict)"("Value"=w344) -> ()  [unwired: 2 in, 2 out]
        n191 = property on="V2 (N.C.)" class="Bool (strict)"("Val(Sgnl)"=w344) -> ()  [unwired: 2 in, 2 out]
        n192 = local read "DOUT task out"() -> (w348:refnum<k21>)
        n193 = local read "AO task out"() -> (w355:refnum<k21>)
        n194 = Build Array(w344, w344, w344) -> (w351:bool[])
        n195 = Not(x=w344) -> (.not. x?=w345:bool)
        n196 = property on="V1 (N.O.)" class="Bool (strict)"("Val(Sgnl)"=w345) -> ()  [unwired: 2 in, 2 out]
        n197 = call <vilib>:"DAQmx Clear Task.vi"("task in"=w355, "error in"=w349) -> ("error out"=w354:errorcluster)  [unwired: 13 in]
        n198 = local write "error out (USB6210/6218 AOUT)"(w354) -> ()
        n199 = call <vilib>:"DAQmx Write (Digital 1D Bool NChan 1Samp 1Line).vi"("task/channels in"=w348, "data"=w351, "timeout"=10.0, "error in"=w352) -> ("task out"=w347:refnum<k21>, "error out"=w346:errorcluster)  [unwired: 9 in, 1 out]
        n200 = call <vilib>:"DAQmx Clear Task.vi"("task in"=w347, "error in"=w346) -> ("error out"=w356:errorcluster)  [unwired: 13 in]
        n201 = local write "error out (USB6210/6218 DOUT)"(w356) -> ()
      }
      event "V1 (N.O.)": Value Change {
        n202 = event-data() -> ()  [unwired: 1 in, 3 out]
        n203 = local read "Cycle #"() -> (w361:u32)
        n204 = Greater?(x=w361, y=u32 0) -> (0:w359:bool)
        n205 = case shown="False" w359 {
          tunnel: "V1 (N.O.)" -> [_ w375]
          tunnel: w358 -> [_ w370]
          frame False {
          }
          frame True {
            n206 = Not(x=w375) -> (.not. x?=w377:bool)
            n207 = local read "error out (USB6210/6218 DOUT)"() -> (w376:errorcluster)
            n208 = property on="V2 (N.C.)" class="Bool (strict)"() -> ("Value"=w374:bool)  [unwired: 2 in, 2 out]
            n209 = property on="OUTPUT\n(Kikusui)" class="Bool (strict)"() -> ("Value"=w373:bool)  [unwired: 2 in, 2 out]
            n210 = local read "DOUT task out"() -> (w380:refnum<k21>)
            n211 = Build Array(w377, w374, w373) -> (w366:bool[])
            n212 = local read "File Refn USB DO"() -> (w371:refnum<file>)
            n213 = Boolean To (0,1)(Boolean=w366) -> (0, 1=w365:i16[])
            n214 = Initialize Array("%d" ("element"), 3 ("dimension size")) -> (w369:string[])
            n215 = call <vilib>:"DAQmx Write (Digital 1D Bool NChan 1Samp 1Line).vi"("task/channels in"=w380, "data"=w366, "timeout"=10.0, "error in"=w376) -> ("task out"=w378:refnum<k21>, "error out"=w364:errorcluster)  [unwired: 9 in, 1 out]
            n216 = local write "DOUT task out"(w378) -> ()
            n217 = Get Date/Time In Seconds() -> (seconds since 1Jan1904=w372:timestamp)
            n218 = call "FileWrite.vi"("DataArray"=w365, "Time Stamp"=w372, "Error In"=w364, "FileFormat"=w369, "Index"=w370, "refnum in"=w371) -> ("Error Out"=w363:errorcluster)  [unwired: 4 in, 1 out]
            n219 = local write "error out (USB6210/6218 DOUT)"(w363) -> ()
          }
        }
      }
      event "V2 (N.C.)": Value Change {
        n220 = event-data() -> ()  [unwired: 1 in, 3 out]
        n221 = local read "Cycle #"() -> (w384:u32)
        n222 = Greater?(x=w384, y=u32 0) -> (0:w382:bool)
        n223 = case shown="True" w382 {
          tunnel: "V2 (N.C.)" -> [_ w399]
          tunnel: w381 -> [_ w391]
          frame False {
          }
          frame True {
            n224 = property on="V1 (N.O.)" class="Bool (strict)"() -> ("Value"=w398:bool)  [unwired: 2 in, 2 out]
            n225 = Not(x=w398) -> (.not. x?=w397:bool)
            n226 = local read "error out (USB6210/6218 DOUT)"() -> (w402:errorcluster)
            n227 = property on="OUTPUT\n(Kikusui)" class="Bool (strict)"() -> ("Value"=w396:bool)  [unwired: 2 in, 2 out]
            n228 = local read "DOUT task out"() -> (w403:refnum<k21>)
            n229 = Build Array(w397, w399, w396) -> (w394:bool[])
            n230 = local read "File Refn USB DO"() -> (w395:refnum<file>)
            n231 = Boolean To (0,1)(Boolean=w394) -> (0, 1=w393:i16[])
            n232 = Initialize Array("%d" ("element"), 3 ("dimension size")) -> (w388:string[])
            n233 = call <vilib>:"DAQmx Write (Digital 1D Bool NChan 1Samp 1Line).vi"("task/channels in"=w403, "data"=w394, "timeout"=10.0, "error in"=w402) -> ("task out"=w400:refnum<k21>, "error out"=w387:errorcluster)  [unwired: 9 in, 1 out]
            n234 = local write "DOUT task out"(w400) -> ()
            n235 = Get Date/Time In Seconds() -> (seconds since 1Jan1904=w392:timestamp)
            n236 = call "FileWrite.vi"("DataArray"=w393, "Time Stamp"=w392, "Error In"=w387, "FileFormat"=w388, "Index"=w391, "refnum in"=w395) -> ("Error Out"=w386:errorcluster)  [unwired: 4 in, 1 out]
            n237 = local write "error out (USB6210/6218 DOUT)"(w386) -> ()
          }
        }
      }
      event "update current", "Set Voltage (V)\n (Kikusui)", "Set Current (mA)\n (Kikusui)": Value Change {
        n238 = event-data() -> ()  [unwired: 1 in, 3 out]
        n239 = case shown="False" "CONTROL KIKUSUI?" {
          tunnel: w419 -> [_ w450]
          tunnel: [w421 w443] -> w418
          tunnel: [w424 w442] -> w417
          tunnel: w416 -> [w426 w445]
          tunnel: w415 -> [w422 w444]
          tunnel: "Set Voltage (V)\n (Kikusui)" -> [_ w435]
          tunnel: "Set Current (mA)\n (Kikusui)" -> [_ w433]
          frame False {
            w423 = 0.0 ("element")
            n240 = Get Date/Time In Seconds() -> (seconds since 1Jan1904=w425:timestamp)
            n241 = local read "AO task out"() -> (w431:refnum<k21>)
            n242 = Build Array (concatenate)(w422, w423) -> (w421:dbl[])
            n243 = Build Array (concatenate)(w426, w425) -> (w424:timestamp[])
            n244 = Build Array(w423, w423) -> (w429:dbl[])
            n245 = call <vilib>:"DAQmx Write (Analog 1D DBL NChan 1Samp).vi"("task/channels in"=w431, "data"=w429, "timeout"=100.0, "error in"=errorcluster {"status"=FALSE, "code"=0, "source"=""}) -> ("task out"=w432:refnum<k21>, "error out"=w427:errorcluster)  [unwired: 9 in, 1 out]
            n246 = local write "AO task out"(w432) -> ()
            n247 = local write "error out (KIKUSI CTRL)"(w427) -> ()
          }
          frame True {
            (unwired) 2.0 ("y")
            n248 = xnode "Formula"("X1"=w433) -> ("Result"=w439:dbl)  [unwired: 1 in, 1 out]
            n249 = Divide(x=w435, y=650.0) -> (x/y=w457:dbl)
            n250 = Multiply(x=10.0 ("y"), y=w457) -> (x*y=w437:dbl)
            n251 = In Range and Coerce(upper limit=0.4, x=w439, lower limit=0.0 ("y")) -> (coerced(x)=w436:dbl, In Range?=w438:bool)
            n252 = case shown="True" w438 {
              tunnel: w437 -> [w464 w467]
              tunnel: w436 -> [_ w466]
              tunnel: [w462 w465] -> w434
              frame False {
                n253 = Build Array(w464, 0.0 ("element")) -> (w462:dbl[])
              }
              frame True {
                n254 = Build Array(w467, w466) -> (w465:dbl[])
              }
            }
            "USB AOUT" <- w434
            n255 = local read "File Refn USB AO"() -> (w451:refnum<file>)
            n256 = Get Date/Time In Seconds() -> (seconds since 1Jan1904=w446:timestamp)
            n257 = Initialize Array("%.3f", 2 ("dimension size")) -> (w452:string[])
            n258 = local read "AO task out"() -> (w459:refnum<k21>)
            n259 = call "FileWrite.vi"("DataArray"=w434, "Time Stamp"=w446, "Error In"=errorcluster {"status"=FALSE, "code"=0, "source"=""} ("error in"), "FileFormat"=w452, "Index"=w450, "refnum in"=w451) -> ("Error Out"=w448:errorcluster, "Byte Stream File Refnum"=w447:refnum<file>)  [unwired: 4 in]
            n260 = Build Array (concatenate)(w445, w446) -> (w442:timestamp[])
            n261 = local write "File Refn USB AO"(w447) -> ()
            n262 = call <vilib>:"DAQmx Write (Analog 1D DBL NChan 1Samp).vi"("task/channels in"=w459, "data"=w434, "timeout"=100.0, "error in"=w448) -> ("task out"=w460:refnum<k21>, "error out"=→"error out (KIKUSI CTRL)":errorcluster)  [unwired: 9 in, 1 out]
            n263 = local write "AO task out"(w460) -> ()
            n264 = Build Array (concatenate)(w444, w433) -> (w443:dbl[])
          }
        }
        n265 = local read "All Labels (USB6218)"() -> (w411:string[])
        n266 = local read "DataArrayConv (USB6218)"() -> (w410:dbl[][])
        n267 = local read "Last Data \n(USB6218)"() -> (w406:dbl[])
        n268 = local read "TimeArray (USB6218)"() -> (w408:timestamp[])
        n269 = Search 1D Array(1D array=w411, element="I_CV") -> (index of element=w412:i32)  [unwired: 1 in]
        n270 = Index Array(array=w410, index (row)=w412) -> (element=w409:dbl[])  [unwired: 1 in]
        n271 = Index Array(array=w406, index=w412) -> (element=→"Monitor Current (mA)":dbl)
        n272 = Bundle("TimeArray (USB6218)"=w408, "DataArrayConv (USB6218)"=w409) -> (w404:T14)  [unwired: 1 in]
      }
      event "upper limit (mA)\n (Kikusui)", "upper limit (V)\n (Kikusui)", "lower limit (mA) \n(Kikusui)", "lower limit (V) \n(Kikusui)": Value Change {
        n273 = event-data() -> ()  [unwired: 1 in, 6 out]
        n274 = property on="Set Current (mA)\n (Kikusui)" class="DigNum (strict)"("Maximum"="upper limit (mA)\n (Kikusui)", "Minimum"="lower limit (mA) \n(Kikusui)") -> ()  [unwired: 2 in, 2 out]
        n275 = property on="Set Voltage (V)\n (Kikusui)" class="DigNum (strict)"("Maximum"="upper limit (V)\n (Kikusui)", "Minimum"="lower limit (V) \n(Kikusui)") -> ()  [unwired: 2 in, 2 out]
      }
      event "OUTPUT\n(Kikusui)": Value Change {
        n276 = event-data() -> ()  [unwired: 1 in, 6 out]
        n277 = local read "Cycle #"() -> (w486:u32)
        n278 = Greater?(x=w486, y=u32 0) -> (0:w484:bool)
        n279 = case shown="True" w484 {
          tunnel: w483 -> [_ w490]
          frame False {
          }
          frame True {
            n280 = property on="V1 (N.O.)" class="Bool (strict)"() -> ("Value"=w501:bool)  [unwired: 2 in, 2 out]
            n281 = Not(x=w501) -> (.not. x?=w500:bool)
            n282 = local read "error out (USB6210/6218 DOUT)"() -> (w504:errorcluster)
            n283 = property on="V2 (N.C.)" class="Bool (strict)"() -> ("Value"=w499:bool)  [unwired: 2 in, 2 out]
            n284 = local read "DOUT task out"() -> (w505:refnum<k21>)
            n285 = Build Array(w500, w499, "OUTPUT\n(Kikusui)") -> (w488:bool[])
            n286 = local read "File Refn USB DO"() -> (w491:refnum<file>)
            n287 = Boolean To (0,1)(Boolean=w488) -> (0, 1=w487:i16[])
            n288 = Initialize Array("%d" ("element"), 3 ("dimension size")) -> (w493:string[])
            n289 = call <vilib>:"DAQmx Write (Digital 1D Bool NChan 1Samp 1Line).vi"("task/channels in"=w505, "data"=w488, "timeout"=10.0, "error in"=w504) -> ("task out"=w502:refnum<k21>, "error out"=w495:errorcluster)  [unwired: 9 in, 1 out]
            n290 = local write "DOUT task out"(w502) -> ()
            n291 = Get Date/Time In Seconds() -> (seconds since 1Jan1904=w492:timestamp)
            n292 = call "FileWrite.vi"("DataArray"=w487, "Time Stamp"=w492, "Error In"=w495, "FileFormat"=w493, "Index"=w490, "refnum in"=w491) -> ("Error Out"=w494:errorcluster, "Byte Stream File Refnum"=w489:refnum<file>)  [unwired: 4 in]
            n293 = local write "File Refn USB DO"(w489) -> ()
            n294 = local write "error out (USB6210/6218 DOUT)"(w494) -> ()
          }
        }
      }
    }
    n295 = Bundle(w337, w334) -> (w336:cluster{timestamp[], dbl[]})  [unwired: 1 in]
    n296 = Build Array(w336, w333) -> (→"Graph 7":T9)
  }
  n297 = while {
    shift-right: [w578] -> w24
    shift-left: refnum<class "USBData.lvclass"> refnum ("USBData.lvclass") -> [w582]
    shift-right: [w574] -> w23
    shift-left: errorcluster {"status"=FALSE, "code"=0, "source"=""} ("error in (no error)") -> [w581]
    tunnel: "RUN identifier" -> [w516]
    tunnel: "Base Path" -> [w515]
    shift-right: [w556] -> w17
    shift-left: errorcluster {"status"=FALSE, "code"=0, "source"=""} ("error in (no error)") -> [w572]
    shift-right: [w557] -> w18
    shift-left: refnum<class "LSI218Data.lvclass"> refnum ("LSI218Data.lvclass") -> [w571]
    shift-right: [w544] -> w14
    shift-left: refnum<class "LSI336Data.lvclass"> refnum ("LSI336Data.lvclass") -> [w553]
    shift-right: [w543] -> w13
    shift-left: w3 -> [w552]
    shift-right: [w532] -> _
    shift-left: errorcluster {"status"=FALSE, "code"=0, "source"=""} ("error in") -> [w533]
    shift-right: [w521] -> w7
    shift-left: refnum<class "USBData.lvclass"> refnum ("USBData.lvclass") -> [w530]
    shift-right: [w520] -> w6
    shift-left: errorcluster {"status"=FALSE, "code"=0, "source"=""} ("error in (no error)") -> [w529]
    shift-right: [w514] -> _
    shift-left: w3 -> [w513]
    i -> [w528]
    stop <- "Stop Button" stop-if-true
    w539 = u32 24 ("Number of Rows")
    w549 = T16 [] ("appended array")
    w566 = T16 [] ("appended array")
    n298 = control-ref of="Plot selecter LSI218(2)\n    1      2     3     4"() -> (w537:refnum<vi>)
    n299 = control-ref of="Plot selecter LSI218(1)\n    1      2     3     4"() -> (w538:refnum<vi>)
    n300 = control-ref of="Plot selecter LSI336 \n     1      2     3     4"() -> (w536:refnum<vi>)
    n301 = Equal?(x=w528, y=0) -> (x = y?=w517:bool)
    n302 = And(x="Analog Out ON?", y=w517) -> (x .and. y?=w518:bool)
    n303 = property on="Property Node" class="Arr (strict)"(reference=w538, "Number of Rows"=w539) -> ()  [unwired: 1 in, 2 out]
    n304 = property on="Property Node" class="Arr (strict)"(reference=w537, "Number of Rows"=w539) -> ()  [unwired: 1 in, 2 out]
    n305 = case shown="False" w517 {
      tunnel: [w1122 w1134] -> w543
      tunnel: [w1112 w1133] -> w551
      tunnel: [w1121 w1132] -> w544
      tunnel: [w1120 timestamp[] [] ("TimeArray")] -> w509
      tunnel: [w1119 dbl[][] [] ("DataArray")] -> w507
      tunnel: w553 -> [w1118 w1129]
      tunnel: w552 -> [w1117 w1128]
      tunnel: w516 -> [_ w1126]
      tunnel: w528 -> [w1113 _]
      tunnel: w515 -> [_ w1123]
      frame False {
        n306 = local read "Record interval"() -> (w1110:i64)
        n307 = call-dynamic "LSI336Data_measure.vi"("LSI336Data in"=w1118, "MeasurementIndex"=w1113, "error in (no error)"=w1117, "save every ... measurements"=w1110) -> ("Active?"=→"Active?\n(LSI336)":bool[], "TimeMeasuremeent"=→"Time of Last Measurement (LSI336)":timestamp, "LSI336Data out"=w1121:refnum<class "LSI336Data.lvclass">, "LastData"=→"Last Data \nLSI336":dbl[], "LastMeasurementConfig"=→"LastMeasurementConfig (336)":T10, "DataArray"=w1119:dbl[][], "Status"=w1112:u16, "TimeArray"=w1120:timestamp[], "error out"=w1122:errorcluster)  [unwired: 3 in]
      }
      frame True {
        n308 = Get Date/Time In Seconds() -> (seconds since 1Jan1904=w1135:timestamp)
        n309 = call-dynamic "LSI336Data_initialize.vi"("LSI336Data in"=w1129, "RunName"=w1126, "InstName"="InstName (LSI336)", "FileFormat"="FileFormat (336)", "LSI336Settings(X, Y)"="LSI336Settings(X,Y)", "RUN start time"=w1135, "error in (no error)"=w1128, "base path"=w1123) -> ("LSI336Data out"=w1132:refnum<class "LSI336Data.lvclass">, "Status"=w1133:T7, "AllLabels"=→"Labels LSI336":string[], "error out"=w1134:errorcluster)  [unwired: 4 in]
      }
    }
    "LSI336 Status" <- w551
    "error out (LSI336)" <- w543
    "TimeArray (LSI336)" <- w509
    "DataArray (336)" <- w507
    n310 = case shown="False" w517 {
      tunnel: w582 -> [w1269 w1293]
      tunnel: w581 -> [w1263 w1291]
      tunnel: w528 -> [w1254 _]
      tunnel: [w1261 w1288] -> w574
      tunnel: [w1258 w1287] -> w531
      tunnel: [w1259 w1286] -> w578
      tunnel: [w1249 w1281] -> w579
      tunnel: w516 -> [_ w1279]
      tunnel: w515 -> [_ w1278]
      tunnel: [w1248 w1275] -> w510
      frame False {
        n311 = call-dynamic "USBData_measure.vi"("USBData in"=w1269, "DAQ sample #"=i64 5, "DAQ timeout"=100.0 ("DAQ timeout (def: 100)"), "MeasurementIndex"=w1254, "error in (no error)"=w1263, "save every ... measurements"="Record interval") -> ("USBData out"=w1268:refnum<class "USBData.lvclass">, "TimeMeasuremeent"=w1265:timestamp, "Status"=→"USB6210 Status":T6, "LastDataAcquired"=w1250:dbl[], "error out"=w1264:errorcluster)  [unwired: 3 in, 2 out]
        "Time of Last Measurement (USB6210)" <- w1265
        "Last Vol\n(USB6210)" <- w1250
        n312 = call-dynamic "USBData_convert.vi"("Save every ... measurements"="Record interval", "MeasurementIndex"=w1254, "error in (no error)"=w1264, "LastDataAcquired"=w1250, "TimeMeasuremeent"=w1265, "USBData in"=w1268) -> ("error out"=w1262:errorcluster, "LeakDet_FULL"=w1257:dbl, "LastDataConverted"=w1251:dbl[], "USBData out"=w1260:refnum<class "USBData.lvclass">)  [unwired: 2 in]
        n313 = call "USBData_read.vi"("USBData in"=w1260, "error in (no error)"=w1262) -> ("Status"=w1252:T6, "USBData out"=w1259:refnum<class "USBData.lvclass">, "Data"=w1258:T17, "Basic"=w1249:T18, "error out"=w1261:errorcluster)  [unwired: 2 in, 2 out]
        n314 = local write "USB6210 Status"(w1252) -> ()
        n315 = Unbundle By Name(w1249) -> ("ReadLeakDet?"=w1256:bool)
        n316 = Unbundle By Name(w1249) -> ("Labels"=w1248:string[])
        n317 = case shown="False" w1256 {
          tunnel: w1251 -> [w1270 w1273]
          tunnel: w1257 -> [_ w1272]
          tunnel: [w1270 w1271] -> w1255
          frame False {
          }
          frame True {
            n318 = Build Array (concatenate)(w1273, w1272) -> (w1271:dbl[])
          }
        }
        "Last Data \n(USB6210)" <- w1255
      }
      frame True {
        n319 = Get Date/Time In Seconds() -> (seconds since 1Jan1904=w1280:timestamp)
        n320 = call-dynamic "USBData_initialize.vi"("USBData in"=w1293, "SeriesSetting"="USB6210 Config", "BasePath"=w1278, "RunName"=w1279, "FileName"="InstName (USB6210)", "error in (no error)"=w1291, "RUN start time"=w1280) -> ("Status"=w1274:T6, "USBData out"=w1289:refnum<class "USBData.lvclass">, "error out"=w1290:errorcluster)  [unwired: 4 in, 2 out]
        n321 = local write "USB6210 Status"(w1274) -> ()
        n322 = call "USBData_read.vi"("USBData in"=w1289, "error in (no error)"=w1290) -> ("Status"=w1277:T6, "USBData out"=w1286:refnum<class "USBData.lvclass">, "Data"=w1287:T17, "Basic"=w1281:T18, "error out"=w1288:errorcluster)  [unwired: 2 in, 2 out]
        n323 = local write "USB6210 Status"(w1277) -> ()
        n324 = Unbundle By Name(w1281) -> ("ReadLeakDet?"=w1285:bool, "Labels"=w1275:string[])
        n325 = Array Size(array=w1275) -> (size(s)=w1284:i32)
        n326 = case shown="True" w1285 {
          tunnel: w1284 -> [w1294 w1296]
          tunnel: [w1294 w1295] -> w1282
          frame False {
          }
          frame True {
            n327 = Add(x=w1296, y=1) -> (x+y=w1295:i32)
          }
        }
        n328 = Initialize Array(TRUE ("Activate 2"), w1282) -> ()  [unwired: 1 out]
      }
    }
    "error out (USB6210)" <- w574
    n329 = case shown="False" w517 {
      tunnel: [w799 w827] -> w520
      tunnel: [w796 w826] -> w527
      tunnel: [w797 w825] -> w521
      tunnel: [w788 w820] -> w526
      tunnel: [w787 w817] -> _
      tunnel: w530 -> [w786 w815]
      tunnel: w515 -> [_ w814]
      tunnel: w516 -> [_ w813]
      tunnel: w529 -> [w785 w812]
      tunnel: w528 -> [w784 _]
      frame False {
        n330 = local read "Record interval"() -> (w783:i64)
        n331 = call-dynamic "USBData_measure.vi"("USBData in"=w786, "DAQ sample #"=i64 5, "DAQ timeout"=100.0 ("DAQ timeout (def: 100)"), "MeasurementIndex"=w784, "error in (no error)"=w785, "save every ... measurements"=w783) -> ("USBData out"=w805:refnum<class "USBData.lvclass">, "TimeMeasuremeent"=w802:timestamp, "Status"=→"USB6218 Status":T6, "LastDataAcquired"=w789:dbl[], "error out"=w801:errorcluster)  [unwired: 3 in, 2 out]
        "Time of Last Measurement (USB6218)" <- w802
        "Last Vol \n(USB6218)" <- w789
        n332 = call-dynamic "USBData_convert.vi"("Save every ... measurements"=w783, "MeasurementIndex"=w784, "error in (no error)"=w801, "LastDataAcquired"=w789, "TimeMeasuremeent"=w802, "USBData in"=w805) -> ("error out"=w800:errorcluster, "LeakDet_FULL"=w795:dbl, "LastDataConverted"=w790:dbl[], "USBData out"=w798:refnum<class "USBData.lvclass">)  [unwired: 2 in]
        n333 = call "USBData_read.vi"("USBData in"=w798, "error in (no error)"=w800) -> ("Status"=w791:T6, "USBData out"=w797:refnum<class "USBData.lvclass">, "Data"=w796:T17, "Basic"=w788:T18, "error out"=w799:errorcluster)  [unwired: 2 in, 2 out]
        n334 = local write "USB6218 Status"(w791) -> ()
        n335 = Unbundle By Name(w788) -> ("ReadLeakDet?"=w794:bool)
        n336 = Unbundle By Name(w788) -> ("Labels"=w787:string[])
        n337 = case shown="True" w794 {
          tunnel: w790 -> [w806 w809]
          tunnel: w795 -> [_ w808]
          tunnel: [w806 w807] -> w793
          frame False {
          }
          frame True {
            n338 = Build Array (concatenate)(w809, w808) -> (w807:dbl[])
          }
        }
        "Last Data \n(USB6218)" <- w793
      }
      frame True {
        n339 = Get Date/Time In Seconds() -> (seconds since 1Jan1904=w819:timestamp)
        n340 = call-dynamic "USBData_initialize.vi"("USBData in"=w815, "SeriesSetting"="USB6218 Config", "BasePath"=w814, "RunName"=w813, "FileName"="InstName (USB6218)", "error in (no error)"=w812, "RUN start time"=w819) -> ("Status"=w810:T6, "USBData out"=w828:refnum<class "USBData.lvclass">, "error out"=w829:errorcluster)  [unwired: 4 in, 2 out]
        n341 = local write "USB6218 Status"(w810) -> ()
        n342 = call "USBData_read.vi"("USBData in"=w828, "error in (no error)"=w829) -> ("Status"=w818:T6, "USBData out"=w825:refnum<class "USBData.lvclass">, "Data"=w826:T17, "Basic"=w820:T18, "error out"=w827:errorcluster)  [unwired: 2 in, 2 out]
        n343 = local write "USB6218 Status"(w818) -> ()
        n344 = Unbundle By Name(w820) -> ("ReadLeakDet?"=w824:bool, "Labels"=w817:string[])
        n345 = Array Size(array=w817) -> (size(s)=w823:i32)
        n346 = case shown="True" w824 {
          tunnel: w823 -> [w830 w832]
          tunnel: [w830 w831] -> w821
          frame False {
          }
          frame True {
            n347 = Add(x=w832, y=1) -> (x+y=w831:i32)
          }
        }
        n348 = Initialize Array(TRUE ("Activate 2"), w821) -> ()  [unwired: 1 out]
      }
    }
    "error out (USB6218)" <- w520
    n349 = case shown="True" w517 {
      tunnel: [w1228 w1243] -> w556
      tunnel: [w1223 w1242] -> w573
      tunnel: [w1226 w1241] -> w557
      tunnel: w528 -> [w1227 _]
      tunnel: w572 -> [w1217 w1236]
      tunnel: w571 -> [w1218 w1235]
      tunnel: w516 -> [_ w1234]
      tunnel: w515 -> [_ w1233]
      tunnel: [w1215 timestamp[] [] ("TimeArray")] -> w570
      tunnel: [w1214 dbl[][] [] ("DataArray")] -> w569
      frame False {
        w1221 = 24 ("index")
        n350 = local read "Record interval"() -> (w1212:i64)
        n351 = call-dynamic "LSI218Data_measure.vi"("LSI218Data in"=w1218, "MeasurementIndex"=w1227, "error in (no error)"=w1217, "save every ... measurements"=w1212) -> ("TimeMeasuremeent"=→"Time of Last Measurement (LSI218)":timestamp, "Active?"=w1222:bool[], "LSI218Data out"=w1226:refnum<class "LSI218Data.lvclass">, "LastMeasurementConfig"=→"LastMeasurementConfig (218)":T10, "LastData"=w1216:dbl[], "Status"=w1223:u16, "TimeArray"=w1215:timestamp[], "DataArray"=w1214:dbl[][], "error out"=w1228:errorcluster)  [unwired: 3 in]
        n352 = Split 1D Array(array=w1222, index=w1221) -> (first subarray=→"Active?\n (1)":bool[], second subarray=→"Active?\n(2)":bool[])
        n353 = Split 1D Array(array=w1216, index=w1221) -> (first subarray=→"Last Data \nLSI218 (1)":dbl[], second subarray=→"Last Data \nLSI218 (2)":dbl[])
      }
      frame True {
        n354 = Get Date/Time In Seconds() -> (seconds since 1Jan1904=w1244:timestamp)
        n355 = call-dynamic "LSI218Data_initialize.vi"("LSI218Settings(A-F)"="LSI218Settings(A-F)", "FileFormat"="FileFormat (218)", "RUN start time"=w1244, "base path"=w1233, "error in (no error)"=w1236, "InstName"="InstName (LSI218)", "RunName"=w1234, "LSI218Data in"=w1235) -> ("error out"=w1243:errorcluster, "Status"=w1242:T7, "AllLabels"=w1232:string[], "LSI218Data out"=w1241:refnum<class "LSI218Data.lvclass">)
        n356 = Split 1D Array(array=w1232, index=24) -> (first subarray=→"Labels LSI218 (1)":string[], second subarray=→"Labels LSI218 (2)":string[])
      }
    }
    "LSI218 Status" <- w573
    "error out (LSI218)" <- w556
    n357 = property on="Property Node" class="Arr (strict)"(reference=w536, "Number of Rows"=u32 8) -> ()  [unwired: 1 in, 2 out]
    n358 = case shown="True" w518 {
      tunnel: w515 -> [_ w599]
      tunnel: w516 -> [_ w598]
      tunnel: [w584 w586] -> w514
      tunnel: w513 -> [w584 w585]
      frame False {
      }
      frame True {
        w597 = "_"
        w607 = 10.0 ("V_lim_max")
        w606 = 0.0 ("V_lim_min")
        w605 = -1 items=["Default"=-1, "RSE"=10083, "Differential"=10106, "Pseudodifferential"=12529] ("output terminal configuration")
        w604 = 10348 items=["Volts"=10348, "From Custom Scale"=10065] ("units")
        n359 = Get Date/Time In Seconds() -> (seconds since 1Jan1904=w602:timestamp)
        n360 = call "LV_UNIXTIME.vi"("current time"=w602) -> ("date/time string"=w595:string)  [unwired: 9 in, 1 out]
        n361 = Concatenate Strings(w595, "_AO" ("string")) -> (w609:string)
        n362 = Concatenate Strings(w598, w597, w595, w597, "USB_AOUT.csv" ("string")) -> (w600:string)
        n363 = Build Path(base path=w599, name or relative path=w600) -> (appended path=w594:path)
        n364 = Open/Create/Replace File(file path (use dialog)=w594, operation (0:open)=T15."open or create") -> (refnum out=w592:refnum<file>)  [unwired: 4 in, 2 out]
        n365 = Build Array("AOUT 0 Label", "AOUT 1 Label") -> (w588:string[])
        n366 = call "FileIntialize.vi"("Error In"=w585, "Labels"=w588, "refnum in"=w592) -> ("Error Out"=w587:errorcluster, "File Refnum"=→"File Refn USB AO":refnum<file>)  [unwired: 7 in]
        n367 = call <vilib>:"DAQmx Create Task.vi"("new task name"=w609, "auto cleanup"=FALSE, "error in"=w587) -> ("task out"=w608:refnum<k21>, "error out"=w610:errorcluster)  [unwired: 11 in]
        n368 = call-poly <vilib>:"DAQmx Create Virtual Channel.vi"("task in"=w608, "maximum value"=w607, "minimum value"=w606, "output terminal configuration"=w605, "physical channels"="AOUT For Voltage CTRL", "units"=w604, "error in"=w610) -> ("task out"=w612:refnum<k21>, "error out"=w613:errorcluster)  [unwired: 7 in]
        n369 = call-poly <vilib>:"DAQmx Create Virtual Channel.vi"("task in"=w612, "maximum value"=w607, "minimum value"=w606, "physical channels"="AOUT for Current CTRL", "error in"=w613) -> ("task out"=w615:refnum<k21>, "error out"=w614:errorcluster)  [unwired: 9 in]
        n370 = call <vilib>:"DAQmx Start Task.vi"("task/channels in"=w615, "error in"=w614) -> ("task out"=→"AO task out":refnum<k21>, "error out"=w586:errorcluster)  [unwired: 12 in]
      }
    }
    "error out (USB6210/6218 AOUT)" <- w514
    n371 = Multiply(x="Measurement Interval (s)", y=u32 1000) -> (x*y=w575:dbl)
    n372 = Wait (ms)(milliseconds to wait=w575) -> ()  [unwired: 1 out]
    n373 = case shown="True" "Digital Out ON?" {
      tunnel: w517 -> [_ w841]
      tunnel: w533 -> [w834 w840]
      tunnel: [w834 w839] -> w532
      tunnel: w531 -> [_ w838]
      tunnel: w516 -> [_ w837]
      tunnel: w515 -> [_ w836]
      tunnel: w510 -> [_ w835]
      frame False {
      }
      frame True {
        n374 = case shown="False" w841 {
          tunnel: w840 -> [w856 w1016]
          tunnel: [w856 w1037] -> w839
          tunnel: w838 -> [w857 _]
          tunnel: w837 -> [_ w1025]
          tunnel: w836 -> [_ w1008]
          tunnel: w835 -> [_ _]
          frame False {
            n375 = flat-sequence {
              frame #0 {
              }
            }
            n376 = local read "All Labels (USB6210)"() -> (w845:string[])
            n377 = Multiply(x="N for sampling", y=i64 2) -> (x*y=w851:i64)
            n378 = local read "Cycle #"() -> (w855:u32)
            n379 = Add(x=w851, y="Mov. Avg Interval") -> (x+y=w853:i64)
            n380 = Search 1D Array(1D array=w845, element="Auto Fll\nDewar P. label") -> (index of element=→"Target Index (P)":i32)  [unwired: 1 in]
            n381 = Search 1D Array(1D array=w845, element="Auto Fll\nHe level label") -> (index of element=→"Target Index (L)":i32)  [unwired: 1 in]
            n382 = Greater?(x=w855, y=w853) -> (0:w849:bool)
            n383 = And(x=w849, y="Auto Fill ON?") -> (x .and. y?=w847:bool)
            n384 = case shown="True" w847 {
              tunnel: w857 -> [_ w888]
              tunnel: "Mov. Avg Interval" -> [_ w872]
              tunnel: w851 -> [_ w868]
              tunnel: "N for sampling" -> [_ w870]
              frame False {
              }
              frame True {
                n385 = local read "Pstd"() -> (→"Pstd history":dbl)
                n386 = local read "Lstd"() -> (→"Lstd history":dbl)
                n387 = local read "Pav (Pa)"() -> (→"Pav history":dbl)
                n388 = local read "Lav (%)"() -> (→"Lav history":dbl)
                n389 = local read "Target Index (P)"() -> (w889:i32)
                n390 = local read "Target Index (L)"() -> (w875:i32)
                n391 = Unbundle By Name(w888) -> ("TimeArray"=w886:timestamp[], "DataArrayConv"=w887:dbl[][])
                n392 = Index Array(array=w887, index (col) #1=w889, index (col) #2=w875) -> (element #1=w874:dbl[], element #2=w869:dbl[])  [unwired: 2 in]
                n393 = Delete From Array(array=w874, length=w868) -> (deleted portion=w883:dbl[])  [unwired: 1 in, 1 out]
                n394 = Delete From Array(array=w869, length=w868) -> (deleted portion=w867:dbl[])  [unwired: 1 in, 1 out]
                n395 = call "MovingAverage.vi"("Moving Average interval"=w872, "Input Array"=w869) -> ("M.A. Array"=w871:dbl[])  [unwired: 9 in]
                n396 = call "MovingAverage.vi"("Moving Average interval"=w872, "Input Array"=w874) -> ("M.A. Array"=w873:dbl[])  [unwired: 9 in]
                n397 = Delete From Array(array=w873, length=w868) -> (deleted portion=w884:dbl[])  [unwired: 1 in, 1 out]
                n398 = Delete From Array(array=w873, length=w870) -> (deleted portion=w880:dbl[])  [unwired: 1 in, 1 out]
                "Last N M.A. Pressures" <- w880
                n399 = Delete From Array(array=w871, length=w870) -> (deleted portion=w862:dbl[])  [unwired: 1 in, 1 out]
                "Last N M.A. Levels" <- w862
                n400 = Delete From Array(array=w886, length=w868) -> (deleted portion=w864:timestamp[])  [unwired: 1 in, 1 out]
                n401 = Bundle("TimeArray"=w864, "DataArrayConv"=w883) -> (w882:T19)  [unwired: 1 in]
                n402 = Bundle("TimeArray"=w864, "M.A. Array"=w884) -> (w885:T20)  [unwired: 1 in]
                n403 = Bundle("TimeArray"=w864, "DataArrayConv"=w867) -> (w866:T19)  [unwired: 1 in]
                n404 = Bundle("TimeArray"=w864, "M.A. Array"=w862) -> (w863:T20)  [unwired: 1 in]
                n405 = Array Size(array=w880) -> (size(s)=w879:i32)
                n406 = Equal?(x=w879, y=w870) -> (x = y?=w878:bool)
                n407 = Build Array(w882, w885) -> (→"Dewar Pressure":T21)
                n408 = Build Array(w866, w863) -> (→"He Level":T21)
                n409 = case shown="True" w878 {
                  tunnel: [w993 w998] -> w861
                  tunnel: w880 -> [_ w999]
                  tunnel: w862 -> [_ w996]
                  tunnel: [w993 w994] -> w860
                  frame False {
                    w993 = nan ("mean")
                  }
                  frame True {
                    n410 = call <vilib>:"Std Deviation and Variance.vi"("X"=w999) -> ("mean"=w998:dbl, "standard deviation"=w997:dbl)  [unwired: 1 in, 1 out]
                    n411 = call <vilib>:"Std Deviation and Variance.vi"("X"=w996) -> ("mean"=w994:dbl, "standard deviation"=w995:dbl)  [unwired: 1 in, 1 out]
                    n412 = local write "Pstd"(w997) -> ()
                    n413 = local write "Lstd"(w995) -> ()
                    n414 = local write "Pav (Pa)"(w998) -> ()
                    n415 = local write "Lav (%)"(w994) -> ()
                  }
                }
                n416 = flat-sequence {
                  tunnel: w861 -> [w890]
                  tunnel: w860 -> [w891]
                  frame #0 {
                    n417 = flat-sequence {
                      tunnel: w891 -> [w893]
                      tunnel: w890 -> [w892]
                      tunnel: w890 -> [w961]
                      frame #0 {
                        n418 = stacked-sequence {
                          tunnel: w893 -> [w900 w904 _ _ _ _]
                          tunnel: w892 -> [_ _ w918 w927 w936 w945]
                          frame #0 {
                            n419 = local read "L_low (%)"() -> (w899:dbl)
                            n420 = local read "Fill state"() -> (w897:bool)
                            n421 = Less?(x=w900, y=w899) -> (x < y?=w896:bool)
                            n422 = Equal?(x=w897, y=FALSE) -> (x = y?=w895:bool)
                            n423 = And(x=w896, y=w895) -> (x .and. y?=w894:bool)
                            n424 = case shown="False" w894 {
                              frame False {
                              }
                              frame True {
                                w902 = TRUE ("Value (Signaling)")
                                n425 = property on="Fill state" class="Bool (strict)"("Val(Sgnl)"=w902) -> ()  [unwired: 2 in, 2 out]
                                n426 = Not(x=w902) -> (.not. x?=w901:bool)
                                n427 = property on="Fill (false)" class="Bool (strict)"("Val(Sgnl)"=w901) -> ()  [unwired: 2 in, 2 out]
                              }
                            }
                          }
                          frame #1 {
                            n428 = local read "L_high (%)"() -> (w905:dbl)
                            n429 = local read "Fill state"() -> (w908:bool)
                            n430 = Greater?(x=w904, y=w905) -> (0:w903:bool)
                            n431 = Equal?(x=w908, y=TRUE) -> (x = y?=w907:bool)
                            n432 = And(x=w903, y=w907) -> (x .and. y?=w906:bool)
                            n433 = case shown="True" w906 {
                              frame False {
                              }
                              frame True {
                                w910 = FALSE ("Value (Signaling)")
                                n434 = property on="Fill state" class="Bool (strict)"("Val(Sgnl)"=w910) -> ()  [unwired: 2 in, 2 out]
                                n435 = Not(x=w910) -> (.not. x?=w911:bool)
                                n436 = property on="Fill (false)" class="Bool (strict)"("Val(Sgnl)"=w911) -> ()  [unwired: 2 in, 2 out]
                              }
                            }
                          }
                          frame #2 {
                            n437 = local read "P_1_low (Pa)"() -> (w917:dbl)
                            n438 = property on="state 1" class="Bool (strict)"() -> ("Value"=w915:bool)  [unwired: 2 in, 2 out]
                            n439 = Less?(x=w918, y=w917) -> (x < y?=w914:bool)
                            n440 = Equal?(x=w915, y=FALSE) -> (x = y?=w913:bool)
                            n441 = And(x=w913, y=w914) -> (x .and. y?=w912:bool)
                            n442 = case shown="True" w912 {
                              frame False {
                              }
                              frame True {
                                w920 = TRUE ("Value (Signaling)")
                                n443 = property on="state 1" class="Bool (strict)"("Val(Sgnl)"=w920) -> ()  [unwired: 2 in, 2 out]
                                n444 = Not(x=w920) -> (.not. x?=w919:bool)
                                n445 = property on="state 1 (false)" class="Bool (strict)"("Val(Sgnl)"=w919) -> ()  [unwired: 2 in, 2 out]
                              }
                            }
                          }
                          frame #3 {
                            n446 = local read "P_1_high (Pa)"() -> (w926:dbl)
                            n447 = property on="state 1" class="Bool (strict)"() -> ("Value"=w924:bool)  [unwired: 2 in, 2 out]
                            n448 = Greater?(x=w927, y=w926) -> (0:w923:bool)
                            n449 = Equal?(x=w924, y=TRUE) -> (x = y?=w922:bool)
                            n450 = And(x=w922, y=w923) -> (x .and. y?=w921:bool)
                            n451 = case shown="True" w921 {
                              frame False {
                              }
                              frame True {
                                w929 = FALSE ("Value (Signaling)")
                                n452 = property on="state 1" class="Bool (strict)"("Val(Sgnl)"=w929) -> ()  [unwired: 2 in, 2 out]
                                n453 = Not(x=w929) -> (.not. x?=w928:bool)
                                n454 = property on="state 1 (false)" class="Bool (strict)"("Val(Sgnl)"=w928) -> ()  [unwired: 2 in, 2 out]
                              }
                            }
                          }
                          frame #4 {
                            n455 = local read "P_2_low (Pa)"() -> (w935:dbl)
                            n456 = property on="state 2" class="Bool (strict)"() -> ("Value"=w930:bool)  [unwired: 2 in, 2 out]
                            n457 = Less?(x=w936, y=w935) -> (x < y?=w933:bool)
                            n458 = Equal?(x=w930, y=FALSE) -> (x = y?=w932:bool)
                            n459 = And(x=w932, y=w933) -> (x .and. y?=w931:bool)
                            n460 = case shown="True" w931 {
                              frame False {
                              }
                              frame True {
                                w937 = TRUE ("Value (Signaling)")
                                n461 = property on="state 2" class="Bool (strict)"("Val(Sgnl)"=w937) -> ()  [unwired: 2 in, 2 out]
                                n462 = Not(x=w937) -> (.not. x?=w938:bool)
                                n463 = property on="state 2 (false)" class="Bool (strict)"("Val(Sgnl)"=w938) -> ()  [unwired: 2 in, 2 out]
                              }
                            }
                          }
                          frame #5 {
                            n464 = local read "P_2_high (Pa)"() -> (w944:dbl)
                            n465 = property on="state 2" class="Bool (strict)"() -> ("Value"=w939:bool)  [unwired: 2 in, 2 out]
                            n466 = Greater?(x=w945, y=w944) -> (0:w942:bool)
                            n467 = Equal?(x=w939, y=TRUE) -> (x = y?=w941:bool)
                            n468 = And(x=w941, y=w942) -> (x .and. y?=w940:bool)
                            n469 = case shown="True" w940 {
                              frame False {
                              }
                              frame True {
                                w946 = FALSE ("Value (Signaling)")
                                n470 = property on="state 2" class="Bool (strict)"("Val(Sgnl)"=w946) -> ()  [unwired: 2 in, 2 out]
                                n471 = Not(x=w946) -> (.not. x?=w947:bool)
                                n472 = property on="state 2 (false)" class="Bool (strict)"("Val(Sgnl)"=w947) -> ()  [unwired: 2 in, 2 out]
                              }
                            }
                          }
                        }
                      }
                      frame #1 {
                        n473 = property on="Fill state" class="Bool (strict)"() -> ("Value"=w948:bool)  [unwired: 2 in, 2 out]
                        n474 = case shown="True" w948 {
                          frame False {
                            n475 = property on="V1 (N.O.)" class="Bool (strict)"("Val(Sgnl)"=TRUE ("V1 (N.O.)")) -> ()  [unwired: 2 in, 2 out]
                            n476 = property on="V2 (N.C.)" class="Bool (strict)"("Val(Sgnl)"=FALSE ("Value (Signaling)")) -> ()  [unwired: 2 in, 2 out]
                          }
                          frame True {
                            n477 = property on="state 1" class="Bool (strict)"() -> ("Value"=w952:bool)  [unwired: 2 in, 2 out]
                            n478 = property on="state 2" class="Bool (strict)"() -> ("Value"=w951:bool)  [unwired: 2 in, 2 out]
                            n479 = case shown="True" w952 {
                              frame False {
                                n480 = property on="V1 (N.O.)" class="Bool (strict)"("Val(Sgnl)"=TRUE ("Value (Signaling)")) -> ()  [unwired: 2 in, 2 out]
                                n481 = local write "Status V1 CTRL"(enum16{"Pressurize", "Release"}."Release" ("Status V1 CTRL")) -> ()
                              }
                              frame True {
                                n482 = property on="V1 (N.O.)" class="Bool (strict)"("Val(Sgnl)"=FALSE ("V1 (N.O.)")) -> ()  [unwired: 2 in, 2 out]
                                n483 = local write "Status V1 CTRL"(enum16{"Pressurize", "Release"}."Pressurize" ("Status V1 CTRL")) -> ()
                              }
                            }
                            n484 = case shown="True" w951 {
                              frame False {
                                n485 = property on="V2 (N.C.)" class="Bool (strict)"("Val(Sgnl)"=FALSE ("Value (Signaling)")) -> ()  [unwired: 2 in, 2 out]
                                n486 = local write "Status V2 CTRL"(enum16{"Pressurize", "Release"}."Release" ("Status V2 CTRL")) -> ()
                              }
                              frame True {
                                n487 = property on="V2 (N.C.)" class="Bool (strict)"("Val(Sgnl)"=TRUE ("Value (Signaling)")) -> ()  [unwired: 2 in, 2 out]
                                n488 = local write "Status V2 CTRL"(enum16{"Pressurize", "Release"}."Pressurize" ("Status V2 CTRL")) -> ()
                              }
                            }
                          }
                        }
                      }
                      frame #2 {
                        n489 = Greater?(x=w961, y="P_safelimit_high (Pa)") -> (0:w963:bool)
                        n490 = Less?(x=w961, y="P_safelimit_low (Pa)") -> (x < y?=w965:bool)
                        n491 = Or(x=w963, y=w965) -> (x .or. y?=w966:bool)
                        n492 = case shown="False" w966 {
                          frame False {
                          }
                          frame True {
                            w967 = FALSE ("Value (Signaling)")
                            w969 = FALSE ("Value (Signaling)")
                            n493 = property on="V2 (N.C.)" class="Bool (strict)"("Val(Sgnl)"=FALSE ("V1 (N.O.)")) -> ()  [unwired: 2 in, 2 out]
                            n494 = property on="V1 (N.O.)" class="Bool (strict)"("Val(Sgnl)"=TRUE ("V1 (N.O.)")) -> ()  [unwired: 2 in, 2 out]
                            n495 = property on="state 1" class="Bool (strict)"("Val(Sgnl)"=w967) -> ()  [unwired: 2 in, 2 out]
                            n496 = property on="state 2" class="Bool (strict)"("Val(Sgnl)"=w969) -> ()  [unwired: 2 in, 2 out]
                            n497 = Not(x=w967) -> (.not. x?=w968:bool)
                            n498 = Not(x=w969) -> (.not. x?=w970:bool)
                            n499 = property on="state 1 (false)" class="Bool (strict)"("Val(Sgnl)"=w968) -> ()  [unwired: 2 in, 2 out]
                            n500 = property on="state 2 (false)" class="Bool (strict)"("Val(Sgnl)"=w970) -> ()  [unwired: 2 in, 2 out]
                          }
                        }
                      }
                    }
                  }
                  frame #1 {
                    n501 = property on="V1 (N.O.)" class="Bool (strict)"() -> ("Value"=w991:bool)  [unwired: 2 in, 2 out]
                    n502 = local read "L_high (%)"() -> (w981:dbl)
                    n503 = property on="V2 (N.C.)" class="Bool (strict)"() -> ("Value"=w980:bool)  [unwired: 2 in, 2 out]
                    n504 = local read "P_1_high (Pa)"() -> (w985:dbl)
                    n505 = local read "P_2_high (Pa)"() -> (w983:dbl)
                    n506 = local read "P_1_low (Pa)"() -> (w986:dbl)
                    n507 = local read "P_2_low (Pa)"() -> (w984:dbl)
                    n508 = local read "L_low (%)"() -> (w982:dbl)
                    n509 = local read "Pav (Pa)"() -> (w974:dbl)
                    n510 = Boolean To (0,1)(Boolean=w991) -> (0, 1=w992:i16)
                    n511 = local read "Lav (%)"() -> (w973:dbl)
                    n512 = Boolean To (0,1)(Boolean=w980) -> (0, 1=w979:i16)
                    n513 = local read "File Refn DewarCTRL"() -> (w987:refnum<file>)
                    n514 = local read "Cycle #"() -> (w990:u32)
                    n515 = Build Array(w974, w973, w986, w985, w984, w983, w982, w981, w992, w979) -> (w978:dbl[])
                    n516 = Get Date/Time In Seconds() -> (seconds since 1Jan1904=w988:timestamp)
                    n517 = call "FileWrite.vi"("DataArray"=w978, "Time Stamp"=w988, "Error In"=errorcluster {"status"=FALSE, "code"=0, "source"=""}, "FileFormat"=string[] ["%4.5e", "%4.2f", "%4.4e", "%4.4e", "%4.4e", "%4.4e", "%4.4e", "%d", "%d"] ("Array"), "Index"=w990, "refnum in"=w987) -> ("Error Out"=→"Error Out (Dewar CTRL":errorcluster, "Byte Stream File Refnum"=w977:refnum<file>)  [unwired: 4 in]
                    n518 = local write "File Refn DewarCTRL"(w977) -> ()
                  }
                }
              }
            }
          }
          frame True {
            w1031 = "_"
            w1000 = FALSE ("auto cleanup")
            w1036 = 1 items=["one channel for each line", "one channel for all lines"] ("line grouping")
            n519 = flat-sequence {
              frame #0 {
                w1051 = FALSE ("V1 (N.O.)")
                n520 = local write "V1 (N.O.)"(TRUE ("V1 (N.O.)")) -> ()
                n521 = local write "V2 (N.C.)"(FALSE ("V1 (N.O.)")) -> ()
                n522 = local write "state 1"(w1051) -> ()
                n523 = local write "state 2"(w1051) -> ()
                n524 = local write "Fill state"(w1051) -> ()
                n525 = Not(x=w1051) -> (.not. x?=w1053:bool)
                n526 = Not(x=w1051) -> (.not. x?=w1052:bool)
                n527 = local write "state 1 (false)"(w1052) -> ()
                n528 = local write "state 2 (false)"(w1052) -> ()
                n529 = local write "Fill (false)"(w1053) -> ()
              }
            }
            n530 = Get Date/Time In Seconds() -> (seconds since 1Jan1904=w1048:timestamp)
            n531 = call "LV_UNIXTIME.vi"("current time"=w1048) -> ("date/time string"=w1026:string)  [unwired: 9 in, 1 out]
            n532 = Concatenate Strings(w1026, "_DO" ("new task name")) -> (w1045:string)
            n533 = Concatenate Strings(w1025, w1031, w1026, w1031) -> (w1007:string)
            n534 = Concatenate Strings(w1007, "DEWAR.csv" ("string")) -> (w1006:string)
            n535 = Concatenate Strings(w1007, "USB_DOUT.csv" ("string")) -> (w1010:string)
            n536 = Build Path(base path=w1008, name or relative path=w1006) -> (appended path=w1005:path)
            n537 = Build Path(base path=w1008, name or relative path=w1010) -> (appended path=w1030:path)
            n538 = Open/Create/Replace File(file path (use dialog)=w1030, error in=w1016, operation (0:open)=T15."open or create") -> (refnum out=w1028:refnum<file>, error out=w1015:errorcluster)  [unwired: 3 in, 1 out]
            n539 = call "FileIntialize.vi"("Error In"=w1015, "Labels"="DOUT Labels", "refnum in"=w1028) -> ("Error Out"=w1002:errorcluster, "File Refnum"=→"File Refn USB DO":refnum<file>)  [unwired: 7 in]
            n540 = Open/Create/Replace File(file path (use dialog)=w1005, error in=w1002, operation (0:open)=T15."open or create") -> (refnum out=w1013:refnum<file>, error out=w1014:errorcluster)  [unwired: 3 in, 1 out]
            n541 = call "FileIntialize.vi"("Error In"=w1014, "Labels"=string[] ["P_av", "L_av", "P_1_low", "P_1_high", "P_2_low", "P_2_high", "L_low", "L_high", "V1(NO)", "V2(NC)"], "refnum in"=w1013) -> ("Error Out"=w1001:errorcluster, "File Refnum"=→"File Refn DewarCTRL":refnum<file>)  [unwired: 7 in]
            n542 = Index Array(array="DOUT Physical CH", index=2) -> (element=w1018:tag)
            n543 = Index Array(array="DOUT Physical CH", index=1) -> (element=w1021:tag)
            n544 = Index Array(array="DOUT Physical CH", index=0) -> (element=w1023:tag)
            n545 = call <vilib>:"DAQmx Create Task.vi"("new task name"=w1045, "auto cleanup"=FALSE, "error in"=w1001) -> ("task out"=w1046:refnum<k21>, "error out"=w1047:errorcluster)  [unwired: 11 in]
            n546 = call-poly <vilib>:"DAQmx Create Virtual Channel.vi"("task in"=w1046, "lines"=w1023, "line grouping"=w1036, "error in"=w1047) -> ("task out"=w1049:refnum<k21>, "error out"=w1050:errorcluster)  [unwired: 10 in]
            n547 = call-poly <vilib>:"DAQmx Create Virtual Channel.vi"("task in"=w1049, "lines"=w1021, "line grouping"=w1036, "error in"=w1050) -> ("task out"=w1035:refnum<k21>, "error out"=w1033:errorcluster)  [unwired: 10 in]
            n548 = call-poly <vilib>:"DAQmx Create Virtual Channel.vi"("task in"=w1035, "lines"=w1018, "line grouping"=w1036, "error in"=w1033) -> ("task out"=w1034:refnum<k21>, "error out"=w1032:errorcluster)  [unwired: 10 in]
            n549 = call <vilib>:"DAQmx Start Task.vi"("task/channels in"=w1034, "error in"=w1032) -> ("task out"=w1040:refnum<k21>, "error out"=w1038:errorcluster)  [unwired: 12 in]
            n550 = Build Array(w1000, w1000, w1000) -> (w1041:bool[])
            n551 = call <vilib>:"DAQmx Write (Digital 1D Bool NChan 1Samp 1Line).vi"("task/channels in"=w1040, "data"=w1041, "timeout"=10.0, "error in"=w1038) -> ("task out"=→"DOUT task out":refnum<k21>, "error out"=w1037:errorcluster)  [unwired: 9 in, 1 out]
          }
        }
      }
    }
    "error out (USB6210/6218 DOUT)" <- w532
    n552 = flat-sequence {
      tunnel: w579 -> [w717]
      tunnel: [w712] -> w567
      tunnel: [w710] -> w565
      tunnel: [w709] -> w562
      tunnel: [w708] -> w560
      tunnel: w531 -> [w703]
      frame #0 {
        w711 = T16 [] ("appended array")
        n553 = Unbundle By Name(w703) -> ("TimeArray"=w720:timestamp[], "DataArrayConv"=w715:dbl[][], "LDArray"=w714:dbl[])
        n554 = Unbundle By Name(w717) -> ("ReadLeakDet?"=w716:bool, "LabelLD"=w719:string, "Labels"=w713:string[])  [unwired: 1 out]
        n555 = case shown="True" w716 {
          tunnel: w719 -> [_ w728]
          tunnel: w715 -> [w722 w727]
          tunnel: w714 -> [_ w726]
          tunnel: [w722 w725] -> w702
          tunnel: w713 -> [w721 w724]
          tunnel: [w721 w723] -> w705
          frame False {
          }
          frame True {
            n556 = Build Array (concatenate)(w727, w726) -> (w725:dbl[][])
            n557 = Build Array (concatenate)(w724, w728) -> (w723:string[])
          }
        }
        "All Labels (USB6210)" <- w705
        "DataArrayConv (USB6210)" <- w702
        n558 = local read "Plot selecter (USB6210)\n    1      2     3     4"() -> (w707:bool[][])
        n559 = control-ref of="Plot selecter (USB6210)\n    1      2     3     4"() -> (w704:refnum<vi>)
        n560 = Array Size(array=w705) -> (size(s)=w718:i32)
        n561 = Array Size(array=w705) -> (size(s)=w706:i32)
        n562 = Array Size(array=w702) -> (size(s)=→"Data Array sizes (6210)":i32[])
        n563 = property on="Property Node" class="Arr (strict)"(reference=w704, "Number of Rows"=w706) -> ()  [unwired: 1 in, 2 out]
        n564 = for {
          N: w718 -> [_]
          tunnel: w702 -> [w749]
          tunnel: w720 -> [w750]
          shift-right: [w745] -> w710
          shift-left: w711 -> [w748]
          shift-right: [w743] -> w708
          shift-left: w711 -> [w746]
          shift-right: [w744] -> w712
          shift-left: w711 -> [w742]
          shift-right: [w741] -> w709
          shift-left: w711 -> [w740]
          tunnel: w707 -> [w739]
          i -> [w734]
          n565 = Index Array(array=w749, index (col)=w734) -> (element=w729:dbl[])  [unwired: 1 in]
          n566 = Index Array(array=w739, index (row) #1=w734, index (col) #1=0 ("index (row)"), index (row) #2=w734, index (col) #2=1 ("index (row)"), index (row) #3=w734, index (col) #3=2 ("index (row)"), index (row) #4=w734, index (col) #4=3 ("index (row)")) -> (element #1=w733:bool, element #2=w732:bool, element #3=w731:bool, element #4=w730:bool)
          n567 = Bundle("TimeArray"=w750, "DataArrayConv"=w729) -> (w747:T19)  [unwired: 1 in]
          n568 = stacked-sequence {
            tunnel: w733 -> [w754 _ _ _]
            tunnel: w748 -> [_ w762 _ _]
            tunnel: w731 -> [_ _ w770 _]
            tunnel: w747 -> [w751 w760 w769 w775]
            tunnel: w730 -> [_ _ _ w778]
            tunnel: w746 -> [_ _ _ w777]
            tunnel: [_ _ _ w776] -> w743
            tunnel: [_ w761 _ _] -> w745
            tunnel: [w753 _ _ _] -> w744
            tunnel: w742 -> [w752 _ _ _]
            tunnel: [_ _ w768 _] -> w741
            tunnel: w740 -> [_ _ w767 _]
            tunnel: w732 -> [_ w759 _ _]
            frame #0 {
              n569 = case shown="True" w754 {
                tunnel: [w755 w758] -> w753
                tunnel: w751 -> [_ w757]
                tunnel: w752 -> [w755 w756]
                frame False {
                }
                frame True {
                  n570 = Build Array (concatenate)(w756, w757) -> (w758:T16)
                }
              }
            }
            frame #1 {
              n571 = case shown="True" w759 {
                tunnel: w762 -> [w763 w766]
                tunnel: [w763 w765] -> w761
                tunnel: w760 -> [_ w764]
                frame False {
                }
                frame True {
                  n572 = Build Array (concatenate)(w766, w764) -> (w765:T16)
                }
              }
            }
            frame #2 {
              n573 = case shown="True" w770 {
                tunnel: [w771 w774] -> w768
                tunnel: w769 -> [_ w773]
                tunnel: w767 -> [w771 w772]
                frame False {
                }
                frame True {
                  n574 = Build Array (concatenate)(w772, w773) -> (w774:T16)
                }
              }
            }
            frame #3 {
              n575 = case shown="True" w778 {
                tunnel: [w779 w782] -> w776
                tunnel: w775 -> [_ w781]
                tunnel: w777 -> [w779 w780]
                frame False {
                }
                frame True {
                  n576 = Build Array (concatenate)(w780, w781) -> (w782:T16)
                }
              }
            }
          }
        }
      }
    }
    n577 = flat-sequence {
      tunnel: w526 -> [w636]
      tunnel: [w631] -> w525
      tunnel: [w629] -> w524
      tunnel: [w628] -> w523
      tunnel: [w627] -> w522
      tunnel: w527 -> [w623]
      frame #0 {
        w630 = T16 [] ("appended array")
        n578 = Unbundle By Name(w623) -> ("TimeArray"=w619:timestamp[], "DataArrayConv"=w634:dbl[][], "LDArray"=w633:dbl[])
        "TimeArray (USB6218)" <- w619
        n579 = Unbundle By Name(w636) -> ("ReadLeakDet?"=w635:bool, "LabelLD"=w638:string, "Labels"=w632:string[])  [unwired: 1 out]
        n580 = case shown="True" w635 {
          tunnel: w638 -> [_ w646]
          tunnel: w634 -> [w640 w645]
          tunnel: w633 -> [_ w644]
          tunnel: [w640 w643] -> w621
          tunnel: w632 -> [w639 w642]
          tunnel: [w639 w641] -> w624
          frame False {
          }
          frame True {
            n581 = Build Array (concatenate)(w645, w644) -> (w643:dbl[][])
            n582 = Build Array (concatenate)(w642, w646) -> (w641:string[])
          }
        }
        "All Labels (USB6218)" <- w624
        "DataArrayConv (USB6218)" <- w621
        n583 = Array Size(array=w619) -> (size(s)=→"TimeArray size (6218)":i32)
        n584 = local read "Plot selecter (USB6218)\n    1      2     3     4"() -> (w626:bool[][])
        n585 = control-ref of="Plot selecter (USB6218)\n    1      2     3     4"() -> (w622:refnum<vi>)
        n586 = Array Size(array=w624) -> (size(s)=w637:i32)
        n587 = Array Size(array=w624) -> (size(s)=w625:i32)
        n588 = property on="Property Node" class="Arr (strict)"(reference=w622, "Number of Rows"=w625) -> ()  [unwired: 1 in, 2 out]
        n589 = for {
          N: w637 -> [_]
          tunnel: w621 -> [w667]
          tunnel: w619 -> [w668]
          shift-right: [w662] -> w629
          shift-left: w630 -> [w665]
          shift-right: [w660] -> w627
          shift-left: w630 -> [w663]
          shift-right: [w661] -> w631
          shift-left: w630 -> [w659]
          shift-right: [w658] -> w628
          shift-left: w630 -> [w657]
          tunnel: w626 -> [w656]
          i -> [w651]
          n590 = Index Array(array=w667, index (col)=w651) -> (element=w666:dbl[])  [unwired: 1 in]
          n591 = Index Array(array=w656, index (row) #1=w651, index (col) #1=0 ("index (row)"), index (row) #2=w651, index (col) #2=1 ("index (row)"), index (row) #3=w651, index (col) #3=2 ("index (row)"), index (row) #4=w651, index (col) #4=3 ("index (row)")) -> (element #1=w650:bool, element #2=w649:bool, element #3=w648:bool, element #4=w647:bool)
          n592 = Bundle("TimeArray"=w668, "DataArrayConv"=w666) -> (w664:T19)  [unwired: 1 in]
          n593 = stacked-sequence {
            tunnel: w650 -> [w672 _ _ _]
            tunnel: w665 -> [_ w680 _ _]
            tunnel: w648 -> [_ _ w688 _]
            tunnel: w664 -> [w669 w678 w687 w693]
            tunnel: w647 -> [_ _ _ w696]
            tunnel: w663 -> [_ _ _ w695]
            tunnel: [_ _ _ w694] -> w660
            tunnel: [_ w679 _ _] -> w662
            tunnel: [w671 _ _ _] -> w661
            tunnel: w659 -> [w670 _ _ _]
            tunnel: [_ _ w686 _] -> w658
            tunnel: w657 -> [_ _ w685 _]
            tunnel: w649 -> [_ w677 _ _]
            frame #0 {
              n594 = case shown="True" w672 {
                tunnel: [w673 w676] -> w671
                tunnel: w669 -> [_ w675]
                tunnel: w670 -> [w673 w674]
                frame False {
                }
                frame True {
                  n595 = Build Array (concatenate)(w674, w675) -> (w676:T16)
                }
              }
            }
            frame #1 {
              n596 = case shown="True" w677 {
                tunnel: w680 -> [w681 w684]
                tunnel: [w681 w683] -> w679
                tunnel: w678 -> [_ w682]
                frame False {
                }
                frame True {
                  n597 = Build Array (concatenate)(w684, w682) -> (w683:T16)
                }
              }
            }
            frame #2 {
              n598 = case shown="True" w688 {
                tunnel: [w689 w692] -> w686
                tunnel: w687 -> [_ w691]
                tunnel: w685 -> [w689 w690]
                frame False {
                }
                frame True {
                  n599 = Build Array (concatenate)(w690, w691) -> (w692:T16)
                }
              }
            }
            frame #3 {
              n600 = case shown="True" w696 {
                tunnel: [w697 w700] -> w694
                tunnel: w693 -> [_ w699]
                tunnel: w695 -> [w697 w698]
                frame False {
                }
                frame True {
                  n601 = Build Array (concatenate)(w698, w699) -> (w700:T16)
                }
              }
            }
          }
        }
        n602 = Array Size(array=w621) -> (size(s)=→"DataArraySize (6218)":i32[])
      }
    }
    n603 = local read "Plot selecter LSI218(1)\n    1      2     3     4"() -> (w555:bool[][])
    n604 = local read "Plot selecter LSI218(2)\n    1      2     3     4"() -> (w554:bool[][])
    n605 = Array Size(array=w509) -> (size(s)=→"TimeArray Size (336)":i32)
    n606 = Array Size(array=w507) -> (size(s)=→"DataArray size (336)":i32[])
    n607 = for {
      N: 48 -> [_]
      tunnel: w570 -> [w1156]
      tunnel: w569 -> [w1153]
      tunnel: w555 -> [w1137]
      tunnel: w554 -> [w1138]
      shift-right: [w1154] -> w568
      shift-left: w566 -> [w1155]
      shift-right: [w1149] -> w563
      shift-left: w566 -> [w1150]
      shift-right: [w1148] -> w561
      shift-left: w566 -> [w1147]
      shift-right: [w1146] -> w559
      shift-left: w566 -> [w1145]
      i -> [w1143]
      n608 = Index Array(array=w1153, index (col)=w1143) -> (element=w1152:dbl[])  [unwired: 1 in]
      n609 = Less?(x=w1143, y=24) -> (x < y?=w1144:bool)
      n610 = case shown="True" w1144 {
        tunnel: [w1161 w1179] -> w1142
        tunnel: [w1160 w1178] -> w1141
        tunnel: [w1159 w1176] -> w1140
        tunnel: [w1158 w1175] -> w1139
        tunnel: w1137 -> [_ w1174]
        tunnel: w1138 -> [w1168 _]
        tunnel: w1143 -> [w1163 w1171]
        frame False {
          n611 = Subtract(x=w1163, y=24) -> (x-y=w1167:i32)
          n612 = Index Array(array=w1168, index (row) #1=w1167, index (col) #1=0 ("index (row)"), index (row) #2=w1167, index (col) #2=1 ("index (row)"), index (row) #3=w1167, index (col) #3=2 ("index (row)"), index (row) #4=w1167, index (col) #4=3 ("index (row)")) -> (element #1=w1161:bool, element #2=w1160:bool, element #3=w1159:bool, element #4=w1158:bool)
        }
        frame True {
          n613 = Index Array(array=w1174, index (row) #1=w1171, index (col) #1=0 ("index (row)"), index (row) #2=w1171, index (col) #2=1 ("index (row)"), index (row) #3=w1171, index (col) #3=2 ("index (row)"), index (row) #4=w1171, index (col) #4=3 ("index (row)")) -> (element #1=w1179:bool, element #2=w1178:bool, element #3=w1176:bool, element #4=w1175:bool)
        }
      }
      n614 = Bundle("TimeArray"=w1156, "DataArray"=w1152) -> (w1151:T22)  [unwired: 1 in]
      n615 = stacked-sequence {
        tunnel: w1155 -> [w1183 _ _ _]
        tunnel: [w1182 _ _ _] -> w1154
        tunnel: w1151 -> [w1181 w1191 w1199 w1207]
        tunnel: w1150 -> [_ w1190 _ _]
        tunnel: [_ w1189 _ _] -> w1149
        tunnel: [_ _ w1198 _] -> w1148
        tunnel: w1147 -> [_ _ w1197 _]
        tunnel: [_ _ _ w1206] -> w1146
        tunnel: w1145 -> [_ _ _ w1205]
        tunnel: w1142 -> [w1180 _ _ _]
        tunnel: w1141 -> [_ w1188 _ _]
        tunnel: w1140 -> [_ _ w1196 _]
        tunnel: w1139 -> [_ _ _ w1204]
        frame #0 {
          n616 = case shown="False" w1180 {
            tunnel: w1181 -> [_ w1185]
            tunnel: w1183 -> [w1184 w1187]
            tunnel: [w1184 w1186] -> w1182
            frame False {
            }
            frame True {
              n617 = Build Array (concatenate)(w1187, w1185) -> (w1186:T4)
            }
          }
        }
        frame #1 {
          n618 = case shown="True" w1188 {
            tunnel: [w1192 w1195] -> w1189
            tunnel: w1191 -> [_ w1194]
            tunnel: w1190 -> [w1192 w1193]
            frame False {
            }
            frame True {
              n619 = Build Array (concatenate)(w1193, w1194) -> (w1195:T4)
            }
          }
        }
        frame #2 {
          n620 = case shown="True" w1196 {
            tunnel: [w1200 w1203] -> w1198
            tunnel: w1199 -> [_ w1202]
            tunnel: w1197 -> [w1200 w1201]
            frame False {
            }
            frame True {
              n621 = Build Array (concatenate)(w1201, w1202) -> (w1203:T4)
            }
          }
        }
        frame #3 {
          n622 = case shown="True" w1204 {
            tunnel: [w1208 w1211] -> w1206
            tunnel: w1207 -> [_ w1210]
            tunnel: w1205 -> [w1208 w1209]
            frame False {
            }
            frame True {
              n623 = Build Array (concatenate)(w1209, w1210) -> (w1211:T4)
            }
          }
        }
      }
    }
    n624 = local read "Plot selecter LSI336 \n     1      2     3     4"() -> (w550:bool[][])
    n625 = local read "Labels LSI336"() -> (w542:string[])
    n626 = Array Size(array=w542) -> (size(s)=w541:i32)
    n627 = for {
      N: w541 -> [_]
      tunnel: w550 -> [w1068]
      shift-right: [w1062] -> w548
      shift-left: w549 -> [w1077]
      shift-right: [w1058] -> w547
      shift-left: w549 -> [w1075]
      shift-right: [w1059] -> w546
      shift-left: w549 -> [w1074]
      shift-right: [w1057] -> w545
      shift-left: w549 -> [w1073]
      tunnel: w507 -> [w1065]
      tunnel: w509 -> [w1063]
      i -> [w1066]
      n628 = Index Array(array=w1065, index (col)=w1066) -> (element=w1064:dbl[])  [unwired: 1 in]
      n629 = Index Array(array=w1068, index (row) #1=w1066, index (col) #1=0 ("index (row)"), index (row) #2=w1066, index (col) #2=1 ("index (row)"), index (row) #3=w1066, index (col) #3=2 ("index (row)"), index (row) #4=w1066, index (col) #4=3 ("index (row)")) -> (element #1=w1067:bool, element #2=w1061:bool, element #3=w1060:bool, element #4=w1056:bool)
      n630 = Bundle("TimeArray"=w1063, "DataArray"=w1064) -> (w1076:T22)  [unwired: 1 in]
      n631 = stacked-sequence {
        tunnel: w1077 -> [w1081 _ _ _]
        tunnel: [w1080 _ _ _] -> w1062
        tunnel: w1076 -> [w1079 w1089 w1097 w1105]
        tunnel: w1075 -> [_ w1088 _ _]
        tunnel: [_ w1087 _ _] -> w1058
        tunnel: [_ _ w1096 _] -> w1059
        tunnel: w1074 -> [_ _ w1095 _]
        tunnel: [_ _ _ w1104] -> w1057
        tunnel: w1073 -> [_ _ _ w1103]
        tunnel: w1067 -> [w1078 _ _ _]
        tunnel: w1061 -> [_ w1086 _ _]
        tunnel: w1060 -> [_ _ w1094 _]
        tunnel: w1056 -> [_ _ _ w1102]
        frame #0 {
          n632 = case shown="False" w1078 {
            tunnel: w1079 -> [_ w1083]
            tunnel: w1081 -> [w1082 w1085]
            tunnel: [w1082 w1084] -> w1080
            frame False {
            }
            frame True {
              n633 = Build Array (concatenate)(w1085, w1083) -> (w1084:T4)
            }
          }
        }
        frame #1 {
          n634 = case shown="True" w1086 {
            tunnel: [w1090 w1093] -> w1087
            tunnel: w1089 -> [_ w1091]
            tunnel: w1088 -> [w1090 w1092]
            frame False {
            }
            frame True {
              n635 = Build Array (concatenate)(w1092, w1091) -> (w1093:T4)
            }
          }
        }
        frame #2 {
          n636 = case shown="True" w1094 {
            tunnel: [w1098 w1101] -> w1096
            tunnel: w1097 -> [_ w1099]
            tunnel: w1095 -> [w1098 w1100]
            frame False {
            }
            frame True {
              n637 = Build Array (concatenate)(w1100, w1099) -> (w1101:T4)
            }
          }
        }
        frame #3 {
          n638 = case shown="True" w1102 {
            tunnel: [w1106 w1109] -> w1104
            tunnel: w1105 -> [_ w1107]
            tunnel: w1103 -> [w1106 w1108]
            frame False {
            }
            frame True {
              n639 = Build Array (concatenate)(w1108, w1107) -> (w1109:T4)
            }
          }
        }
      }
    }
    n640 = Build Array (concatenate)(w567, w568, w548, w525) -> (→"Graph 1":T16)
    n641 = Build Array (concatenate)(w565, w563, w547, w524) -> (→"Graph 2":T16)
    n642 = Build Array (concatenate)(w560, w559, w545, w522) -> (→"Graph 4":T16)
    n643 = Build Array (concatenate)(w562, w561, w546, w523) -> (→"Graph 3":T16)
    "Cycle #" <- w528
  }
  n644 = call-dynamic "USBData_terminate.vi"("error in (no error)"=w23, "USBData in"=w24) -> ("error out"=w25:errorcluster)  [unwired: 8 in, 1 out]
  n645 = call-dynamic "LSI336Data_terminate.vi"("error in (no error)"=w13, "LSI336Data in"=w14) -> ("error out"=w12:errorcluster)  [unwired: 8 in, 1 out]
  n646 = call-dynamic "USBData_terminate.vi"("error in (no error)"=w6, "USBData in"=w7) -> ("error out"=w8:errorcluster)  [unwired: 8 in, 1 out]
  n647 = call "LSI218Data_terminate.vi"("error in (no error)"=w17, "LSI218Data in"=w18) -> ("error out"=w16:errorcluster)  [unwired: 8 in, 1 out]
  n648 = local write "error out (USB6210)"(w25) -> ()
  n649 = local write "error out (LSI336)"(w12) -> ()
  n650 = local write "error out (USB6210)"(w8) -> ()
  n651 = local write "error out (LSI218)"(w16) -> ()
